vi "Civ idle3_1.vi"() -> ()   [LabVIEW 2013]
uses:
  <vilib>/Analysis/Matrix/Numeric/Conversions/Matrix To Array - RM.vi
  <vilib>/Analysis/Matrix/NI_Matrix.lvlib
panel:
  out "Base dissent":dbl format="%#_4g"
  out "Gold":i64 format="%^#.4g"
  out "Dissent \nmultiplication\nmodifier":dbl
  out "SP income":dbl format="%^#.3g"
  out "EP income":dbl format="%^#.3g"
  out "Land conversion rate":dbl format="%#_4e"
  out "BP income":dbl format="%^#.3g"
  in  "Ticks/s":i32
  out "Gold upkeep":dbl format="%^#_4g"
  out "Gold income/s":dbl format="%^#_4g"
  out "BP upkeep":dbl format="%^#.3g"
  out "Trading level":i32
  out "Build points":dbl format="%^#.3g"
  in  "?":T1(tab)
  out "%Hunters":dbl format="%#_3g"
  in  "%Crafters":dbl
  in  "%Engineers":dbl
  in  "%Scientists":dbl
  in  "%Builders":dbl
  in  "%Warriors":dbl
  in  "Taxes level 0":bool
  in  "Taxes level 1":bool
  in  "Taxes level 2":bool
  in  "Taxes level 3":bool
  out "Taxation\nlevel":dbl format="%#_13g"
  in  "Taxes level 4":bool
  out "Food consumption\nmultiplier":dbl
  out "Food dissent mod":dbl
  in  "Normal food\nconsumption":bool
  in  "Highest food\nconsumption":bool
  in  "Higher food\nconsumption":bool
  in  "Taxes level 5":bool
  in  "Taxes level 6":bool
  out "Military\nScience level":i32
  out "Governance\nlevel":i32
  in  "Military science":bool
  in  "Governance":bool
  in  "Physics":bool
  in  "Construction":bool
  out "Physics level":i32
  out "Construction\nlevel":i32
  out "Economics\nlevel":i32
  in  "Economics":bool
  in  "Biology":bool
  out "Biology\nlevel":i32
  out "# of level 1 sciences":i32
  out "# of level 2 sciences":i32
  out "# of level 3 sciences":i32
  out "# of level 4 sciences":i32
  out "# of level 5 sciences":i32
  out "# of level 6 sciences":i32
  out "# of level 7 sciences":i32
  out "# of level 8 sciences":i32
  out "# of level 9 sciences":i32
  out "# of level 10 sciences":i32
  out "Production\nlevel":i32
  in  "Production":bool
  out "Level 2 science price":i32 format="%^.0g"
  out "Level 1 science price":i32 format="%^.0g"
  out "Level 6 science price":i64 format="%^#.1g"
  out "Level 5 science price":i32 format="%^.0g"
  out "Level 4 science price":i32 format="%^.0g"
  out "Level 7 science price":i64 format="%^.0g"
  out "Level 3 science price":i32 format="%^#.1g"
  out "Level 8 science price":i64 format="%^.0g"
  out "Level 9 science price":i64 format="%^#.1g"
  out "Level 10 science price":i64 format="%.0g"
  out "Spear level":i32
  out "Net level":i32
  in  "Sharpened stick":bool
  in  "Net 1":bool
  in  "Net 2":bool
  in  "Stone\nspear":bool
  in  "Bronze\nSpear":bool
  in  "Iron\nSpear":bool
  out "Construction\ntools level":i32
  in  "Stone tools":bool
  in  "Basic\nmetal\ntools":bool
  in  "Advanced\nmetal\ntools":bool
  in  "Horses":bool
  in  "Selective\nbreeding":bool
  in  "Livestock":bool
  out "Animal\ndomestication\nlevel":i32
  in  "Parchment":bool
  in  "Paper":bool
  in  "Movable typeset":bool
  out "Writing level":i32
  in  "Medicine 3":bool
  in  "Medicine 2":bool
  in  "Medicine 1":bool
  out "Medicine level":i32
  in  "Medicine 4":bool
  in  "Printing\nPress":bool
  in  "Crossbow":bool
  out "Bow level":i32
  in  "Bow 1":bool
  in  "Bow 2":bool
  in  "Longbow":bool
  in  "Farming 1":bool
  out "Farming level":i32
  in  "Farming 2":bool
  out "Sword level":i32
  in  "Steel sword":bool
  in  "Iron sword":bool
  in  "Bronze sword":bool
  out "Tax method\nlevel":i32
  in  "Income tax":bool
  in  "Sales tax":bool
  in  "Tariffs":bool
  out "Siege weapon\nlevel":i32
  in  "Trebuchet":bool
  in  "Catapult":bool
  in  "Ballista":bool
  in  "Cannon":bool
  in  "Howitzer":bool
  in  "Rocket artillery":bool
  in  "Trireme":bool
  in  "Raft":bool
  out "Boat level":i32
  out "Chariot level":i32
  in  "Reinforced\nchariot":bool
  in  "Simple\nchariot":bool
  in  "Caravan":bool
  in  "Caravel":bool
  in  "Steamship":bool
  in  "Mechanical\nTelevision":bool
  out "Optics\nlevel":i32
  in  "Telescope":bool
  in  "Light bulb":bool
  in  "Camera":bool
  in  "LCD monitor":bool
  out "Electronics\nlevel":i32
  in  "Radio":bool
  in  "Computer":bool
  out "Vehicle\nlevel":i32
  in  "Steam Powered Train":bool
  in  "Internal combustion engine (cars)":bool
  in  "Aircraft":bool
  in  "Rocket":bool
  in  "Unlock brick house":bool
  in  "Unlock concrete house":bool
  in  "Unlock paved tar roads":bool
  in  "Unlock multilayer stone roads":bool
  in  "Democracy":bool
  in  "Theocracy":bool
  in  "Warrior\nSociety":bool
  in  "Democracy 2":bool
  in  "Theocracy 2":bool
  in  "Warrior\nSociety 2":bool
  in  "Kingdom":bool
  in  "Republic":bool
  in  "Confederacy":bool
  in  "Senate":bool
  in  "Caste system":bool
  in  "Feudalism":bool
  in  "Empire":bool
  in  "Imperialism":bool
  in  "Free market capitalism":bool
  in  "Harbor level 0":bool
  in  "Harbor level 3":bool
  in  "Harbor level 2":bool
  in  "Harbor level 1":bool
  out "Road level":i32
  out "Hut level":i32
  in  "Hut level 0":bool
  in  "Hut level 1":bool
  in  "Hut level 2":bool
  in  "Hut level 3":bool
  out "Road invested points":dbl
  out "Hut invested points":dbl
  in  "Road level 0":bool
  in  "Road level 3":bool
  in  "Road level 2":bool
  in  "Road level 1":bool
  out "Aqueduct level":i32
  out "Market\ninvested points":dbl
  out "Market level":i32
  out "Aqueduct\ninvested points":dbl
  out "Harbor\ninvested points":dbl
  out "Harbor level":i32
  in  "Aqueduct\nlevel 0":bool
  in  "Aqueduct\nlevel 3":bool
  in  "Aqueduct\nlevel 2":bool
  in  "Aqueduct\nlevel 1":bool
  in  "Switch to brick house":bool
  in  "Switch to hut":bool
  out "Brick house\nunlocked":bool=TRUE
  out "Concrete house\nunlocked":bool=TRUE
  in  "Switch to concrete housing":bool
  out "Paved tar roads\nunlocked":bool=TRUE
  out "Mutilayer\nStone roads\nunlocked":bool=TRUE
  in  "Switch to Paved tar roads":bool
  in  "Switch to Multilayer stone road":bool
  in  "Switch to Stone road":bool
  out "Housing type":string="a"
  out "Road type":string="a"
  in  "Market\nlevel 0":bool
  in  "Market\nlevel 3":bool
  in  "Market\nlevel 2":bool
  in  "Market\nlevel 1":bool
  out "School invested points":dbl
  in  "School\nlevel 1":bool
  in  "School\nlevel 2":bool
  in  "School\nlevel 3":bool
  in  "School\nlevel 0":bool
  out "School level":i32
  in  "Wall level 1":bool
  in  "Wall level 2":bool
  in  "Wall level 3":bool
  in  "Wall level 0":bool
  out "Barracks level":i32
  out "Walls level":i32
  out "Wall invested points":dbl
  out "Barracks\ninvested points":dbl
  in  "Barracks\nlevel 3":bool
  in  "Barracks\nlevel 1":bool
  in  "Barracks\nlevel 0":bool
  in  "Barracks\nlevel 2":bool
  out "University level":i32
  in  "University\nlevel 0":bool
  in  "University\nlevel 3":bool
  in  "University\nlevel 2":bool
  in  "University\nlevel 1":bool
  out "University\ninvested points":dbl
  out "Police force level":i32
  out "Temple level":i32
  out "Police force\ninvested points":dbl
  out "Temple\ninvested points":dbl
  in  "Temple\nlevel 0":bool
  in  "Temple\nlevel 3":bool
  in  "Temple\nlevel 2":bool
  in  "Temple\nlevel 1":bool
  in  "Police force 0":bool
  in  "Police force 3":bool
  in  "Police force 2":bool
  in  "Police force 1":bool
  in  "Make Tier 2\nproducts":bool
  out "Tier 2\nproducts\nupkeep":dbl format="%#_13g"
  out "Tier 3\nproducts\nupkeep":dbl format="%#_13g"
  out "Tier 4\nproducts\nupkeep":dbl format="%#_13g"
  out "Tier 1\nproducts":dbl format="%#_4p"
  out "Tier 2\nproducts":dbl format="%#_13g"
  out "Tier 3\nproducts":dbl format="%#_13g"
  out "Tier 4\nproducts":dbl format="%#_13g"
  out "Tier 1\nproducts\nupkeep":dbl format="%#_13g"
  in  "Make Tier3\nproducts":bool
  in  "Make Tier 4\nproducts":bool
  out "hunting b":dbl
  out "hunting a":dbl
  out "warrior a":dbl
  out "warrior b":dbl
  out "warrior c":dbl
  out "1-Dissent/100":dbl format="%#_13g"
  out "Land conv mult":dbl
  out "Warrior b Gov mult":dbl
  out "Gov Economy\nbuildings mod":dbl
  out "Dissent mult per\nmilitary building":dbl
  out "Gov food mult":dbl
  out "Temp land change/s":dbl
  out "Year":i32
  out "Day":i32
  out "Military Modifier":dbl format="%#_13g"
  out "Taxation\nModifier":dbl format="%#_13g"
  out "Non-land production multiplier":dbl
  out "Hut non-land prod mod":dbl
  out "Hut upkeep":dbl
  out "Hut dissent mod":dbl
  out "Road land prod mod":dbl
  out "Road upkeep":dbl
  out "Road expansion bonus":dbl
  out "Trading level no mod":i32
  out "Taxes dissent mod":dbl
  out "Barracks military bonus":dbl
  out "Barracks upkeep":dbl
  out "Wall upkeep":dbl
  out "Wall dissent mod":dbl
  out "Construction multiplier":dbl
  out "Wall warrior % equivalent":dbl
  out "Gov building\nupkeep mod":dbl
  out "School dissent mod":dbl
  out "School upkeep":dbl
  out "School engineer equivalent":dbl
  out "School SP/EP multiplier":dbl
  out "Medicine dissent mod":dbl
  out "Gov populist\nbuildings mod":dbl
  out "Gov elitist\nbuildings mod":dbl
  out "University SP multiplier":dbl
  out "University dissent mod":dbl
  out "University upkeep":dbl
  out "University scientist equivalent":dbl
  out "Food income":dbl
  out "Gold dbl":dbl format="%#_13g"
  out "Road trade modifier":dbl
  out "Market domestic gold mult":dbl
  out "Aqueduct dissent mod":dbl
  out "Aqueduct upkeep":dbl
  out "Police force dissent mult":dbl
  out "Police force upkeep":dbl
  out "Harbor expansion bonus":dbl
  out "Harbor upkeep":dbl
  out "Market trade gold mult":dbl
  out "Market upkeep":dbl
  out "Temple dissent mod":dbl
  out "Temple upkeep":dbl
  out "Harbor military mod":dbl
  out "SP/EP multiplier":dbl
  out "Temple SP/EP multiplier":dbl
  out "Aqueduct food multiplier":dbl
  out "Police force base dissent mod":dbl
  out "Government":string
  out "Dissent":dbl format="%#_4g"
  out "SP":dbl format="%^#.3g"
  out "EP":dbl format="%^#.3g"
  in  "Percentage or absolute":bool
  out "Engineers":i32 format="%^#.3g"
  out "Crafters":i32 format="%^#.3g"
  out "Scientists":i32 format="%^#.3g"
  in  "#Merchants":dbl
  in  "Assign Merchant":bool
  in  "#Engineers":dbl
  in  "Assign Engineer":bool
  in  "#Scientists":dbl
  in  "Assign Scientist":bool
  out "Warriors":i32 format="%^#.3g"
  in  "Assign Builder":bool
  in  "#Builders":dbl
  out "Builders":i32 format="%^#.3g"
  in  "Assign Warrior":bool
  in  "#Warriors":dbl
  out "Unassigned workers":i32
  in  "Assign Hunters":bool
  in  "#Hunters":dbl
  in  "# people":i32
  in  "Increase\nPopulation":bool
  out "Conquered\nland":dbl format="%^#.3g"
  out "Max hunters":i32 format="%^#.3g"
  out "Hunters":i32 format="%^#.3g"
  out "Food/s":dbl format="%^#_5g"
  out "Permanent\nland":dbl format="%^#.3g"
  out "People":i64 format="%^#.3g"
  in  "Stop Loop":bool
  out "Food":dbl format="%^#_5g"
  # "Produces food, but your permanent land cannot support too many hunters"
  # "Unlock after population hits 25"
  # "Conquers land, starting at 1km^2 per warrior, but has diminishing returns"
  # "Unlock after construction 1"
  # "Produces 1 BP/tick, needed for buildings\nand for building upkeep"
  # "Unlock after population hits 100"
  # "Produces 0.1 SP/tick, used for abstract research which unlock upgrades and provide bonuses"
  # "Unlock after population hits 50"
  # "Produces 0.1 EP/tick, used for designing useful tools and upgrades"
  # "Produces Products, used mostly for late game upgrades.  Production scales with permanent land"
  # "Not yet implemented"
  # "Small income from population, 8% dissent before modifiers"
  # "Medium income from population, 15% dissent before modifiers"
  # "Higher  income from population, 25% dissent before modifiers"
  # "Higher  income from population, 40% dissent before modifiers"
  # "Highest  income from population, 60% dissent before modifiers"
  # "No income from population, no dissent added"
  # "Lowest income from population, 3% dissent before modifiers"
  # "Requires Economics 1"
  # "2 food/s/person,\n-30% dissent"
  # "1 food/s/person, no dissent mod"
  # "1.5 food/s/person,\n-15% dissent"
  # "Requires Governance 2"
  # "Each level costs 1000 *10^current level SP"
  # "Reduces diminishing returns \nfrom military size, unlocks \nnew weapons/tactics"
  # "-5% dissent per level,\nunlocks new governments"
  # "Increases EP and SP generation, \nunlocks various upgrades"
  # "Decreases building upkeep costs,\nunlocks buildings"
  # "Increase gold generation,\nunlocks gold and taxation"
  # "Increase food production,\nunlocks farming and medicine"
  # "Increases production by 20%\nper tier per level"
  # "Costs 2M EP\nRequires military 4,\nWarriors are more effective"
  # "Costs 250EP\nHunters and warriors are more effective"
  # "Costs 3000EP\nRequires military 1,\nHunters and warriors are more effective"
  # "Costs 50k EP\nRequires military 2,\nWarriors are more effective"
  # "Costs 3k EP\nRequires biology 1,\nreduces dissent by 10%"
  # "Costs 30k EP\nRequires biology 2,\nreduces dissent by another 5% (15% total)"
  # "Costs 3M EP\nRequires biology 4,\nreduces dissent by another 5% (20% total)"
  # "Costs 300M EP\nRequires biology 6,\nreduces dissent by another 5% (25% total)"
  # "Costs 10k EP\nHunters can produce more food"
  # "Costs 100k EP\nHunters can produce more food"
  # "Costs 10k EP\nImproves EP and SP production by 10%"
  # "Costs 1M EP\nImproves EP and SP production by 10%"
  # "Costs 100M EP\nImproves EP and SP production by 10%"
  # "Costs 10B EP\nImproves EP and SP production by 10%"
  # "Costs 30k EP\nRequires physics 2, construction 2\nBuilders produce 0.25 more BP/tick"
  # "Costs 500k EP\nRequires physics 3,\nconstruction 3,Builders produce 0.25 more BP/tick"
  # "Costs 200M EP\nRequires physics 5,\nconstruction 5,Builders produce 0.5 more BP/tick"
  # "Costs 30M EP\nRequires Biology 3\nImproves warrior effectiveness,  builder BP/tick by 0.25"
  # "Costs 30k EP\nRequires Biology 1\nImproves hunter food production"
  # "Costs 1M EP\nRequires Biology 2\nImproves warrior effectiveness,  builder BP/tick by 0.25"
  # "Costs 200k EP\nRequires military 2,\nWarriors are much more effective, hunters can produce more food"
  # "Costs 300k EP\nRequires military 3, physics 3\nWarriors and Hunters are more effective"
  # "Costs 30M EP\nRequires military 5, physics 4\nWarriors are more effective"
  # "Costs 1B EP\nRequires military 6, physics 5\nWarriors are more effective"
  # "Costs 300k EP\nRequires physics 3,\nImproves trade and hunting"
  # "Costs 3M EP\nRequires physics 4, military 3\nImproves trade and warriors"
  # "Costs 10B EP\nRequires physics 7\nIncreases trade level by 2 and improves warriors"
  # "Costs 100B EP\nRequires physics 8, military 8\nIncreases trade level by 2 and improves warriors"
  # "Costs 500k EP\nRequires Military 3, Physics 3, Improves warrior effectiveness"
  # "Costs 5M EP\nRequires Military 3, Physics 4, Improves warrior effectiveness"
  # "Costs 10M EP\nRequires Economics 4, Physics 4, Increases trade level"
  # "Costs 1M EP\nRequires Military 3\nImproves warrior effectiveness"
  # "Costs 30M EP\nRequires Military 4\nImproves warrior effectiveness"
  # "Costs 1B EP\nRequires Military 6\nImproves warrior effectiveness"
  # "Costs 1M EP\nRequires Economics 3\nImproves taxation effectiveness by 50%"
  # "Costs 30M EP\nRequires Economics 4\nImproves taxation effectiveness by 50%"
  # "Costs 1B EP\nRequires Economics 6\nImproves taxation effectiveness by 50%"
  # "Costs 10M EP\nRequires Biology 3\nRenames hunters to farmers, massive improvements to food production, increases food from tribute"
  # "Costs 100M EP\nRequires Biology 4\nLarge improvements to food production, increases food from tribute"
  # "Costs 5M EP\nRequires Military 3, Physics 4, Improves\nwarrior effectiveness"
  # "Costs 30M EP\nRequires Military 3, Physics 5, Improves\nwarrior effectiveness"
  # "Costs 300M EP\nRequires Military 4, Physics 6, Improves\nwarrior effectiveness"
  # "Costs 3B EP\nRequires Military 6, Physics 7, Improves\nwarrior effectiveness"
  # "Costs 300B EP\nRequires Military 8, Physics 9, Improves\nwarrior effectiveness"
  # "Costs 3T EP\nRequires Military 9, Physics 9, Improves\nwarrior effectiveness"
  # "Internet, not sure if invention or building"
  # "Unlock sattelite network structure"
  # "Costs 300k, requires construction 3"
  # "Costs 10M, requires construction 5"
  # "Costs 1M, requires construction 3"
  # "Costs 30M, requires construction 5"
  # "Requires Governance 1"
  # "Costs 500M SP\nRequires Governance 6"
  # "Costs 100k SP\nRequires Governance 2"
  # "Costs 5M SP\nRequires Governance 4"
  # "All governments gain base dissent as population increases"
  # "Free market capitalism doubles domestic gold produced by the market"
  # "These 3 have not yet been rebalanced"
  # "Government descriptions"
  # "Government playstyle"
  # "Democracy focuses on permanent land and hunters for its main source of food, and will have to rely on taxes, and eventually markets, for its source of gold income.  Even though the military is weak, it is still necessary to be abel to convert land."
  # "Top row governments belong to the democracy path, and get a large bonus to land conversion, and dissent decreases as permanent land increases.  These governments have a slight reduction to their military effectiveness."
  # "Empire can focus either on benefits from conquered land, benefits from permanent land, or a combination of both.  The production bonuses allow you to maintain more high level buildings."
  # "Middle row governments belong to the empire path, and get bonuses to BP point production and food production.  Later levels get small military bonuses."
  # "Bottom row governments belong to the oligarchy path, and get a massive boost to their military, but have a very small land conversion rate.  Conquering more land reduces dissent for these governments."
  # "Oligarchies focus on their powerful military, and have an economy dependent on tribute and trade from conquered land.  Any sort of military upgrade will provide benefits to all parts of your economy, and the extra conquered land will decrease your dissent"
  # "Reduces dissent by 5,10,15%\nImproves non-land production by 10,20,30%\nRequires Construction 1"
  # "Upkeep:        0                          0.01BP                0.03BP              0.15BP"
  # "Cost:             0                          10k   BP              30k BP             150k BP"
  # "Multiply all hut bonuses by 1.2"
  # "Upkeep:        0                          0.015BP              0.045BP            0.225BP"
  # "Cost:             0                          100k   BP             300k BP           1.5M BP"
  # "Upkeep:        0                           0.01BP                0.03BP              0.15BP"
  # "Multiply all hut bonuses by 1.3"
  # "Cost:             0                          1M   BP               3M BP             15M BP"
  # "Increases trade level by 1,2,3\nImproves land production\n by 10,20,30%\nImproves land conversion\nrate by 20,50,100%\nRequires Construction 1"
  # "Upkeep:        0                          0.02BP                0.06BP              0.2BP"
  # "Cost:             0                          50k BP              150k BP             500k BP"
  # "Increases trade level by 2,4,6"
  # "Upkeep:        0                          0.04BP                0.12BP              0.4BP"
  # "Cost:             0                          500k BP             1.5M BP            5M BP"
  # "Increases trade level by 2,4,6\nImproves land production\nby 15,30,45%\nImproves land conversion by 30,75,150%"
  # "Upkeep:        0                          0.06BP                0.18BP              0.6BP"
  # "Cost:             0                          50M BP             150M BP           500M BP"
  # "Improves food output\n by 10,20,30%\nReduced dissent by 2,4,6%\nRequires Construction 3"
  # "Upkeep:              0                     0.01BP             0.03BP                0.15BP"
  # "Cost:                   0                     500k BP           1.5M BP             5M BP"
  # "Improves gold from trade by 15,30,45%\nGives a gold income from permanent land equal to 1,2,3 times the trade income from conquered land\nRequires construction 2, economics 3"
  # "Upkeep:              0                     0.04BP             0.12BP                0.4BP"
  # "Cost:                   0                     5M BP             15M BP              50M BP"
  # "Increases trade level by 1,2,3\nIncreases military effectiveness (b) by 10,20,30%\nImproves land conversion\nrate by 10,25,50%\nRequires Boat level 1"
  # "Upkeep:             0                     0.04BP                0.12BP              0.4BP"
  # "Cost:                  0                     500k BP              1.5M BP           5M BP"
  # "Increases military effectiveness (b) by 10,20,30%\nRequires Construction 2, Military 2"
  # "Upkeep:        0                          0.001GP             0.003GP           0.01GP"
  # "Cost:             0                          100k BP             300k BP            1M BP"
  # "Adds to the base strength of your military, giving the equivalent of 2,4,6% of your population as warriors\nReduces dissent by 5,10,15%\nRequires Construction 3, Military 2"
  # "Upkeep:        0                          0.002GP            0.006GP           0.02GP"
  # "Cost:             0                          1M BP              3M BP              10M BP"
  # "Provides a 5,10,15% bonus to SP/EP production, reduces dissent by 2,4,6%, adds 1,2,3% of population to base  engineers\nRequires Construction 2, Governance 2"
  # "Upkeep:        0                          0.001GP             0.003GP           0.01GP"
  # "Cost:             0                          200k BP             600k BP            2M BP"
  # "Provides a 15,30,45% bonus to SP production, reduces dissent by 2,4,6%, adds 2,4,6% of population to base  scientists\nRequires Construction 2, Governance 2"
  # "Upkeep:        0                          0.005GP             0.015GP          0.05GP"
  # "Cost:             0                          600k BP             2M BP             5M BP"
  # "Use only when base dissent is high"
  # "Increases base dissent by 5, 20, 50%\nDecreases dissent multiplier by 13, 26, 40%\nRequires Governance 3"
  # "Upkeep:        0                          0.002GP             0.006GP          0.02 GP"
  # "Cost:             0                          100k GP             1M GP             10M GP"
  # "Reduces dissent by 3,6,9%,\nRequires Construction 1\n3 times as effective if you\nare a theocracy"
  # "Upkeep:        0                          0.001GP             0.003GP           0.01GP"
  # "Cost:             0                          500 GP               10k GP             500k GP"
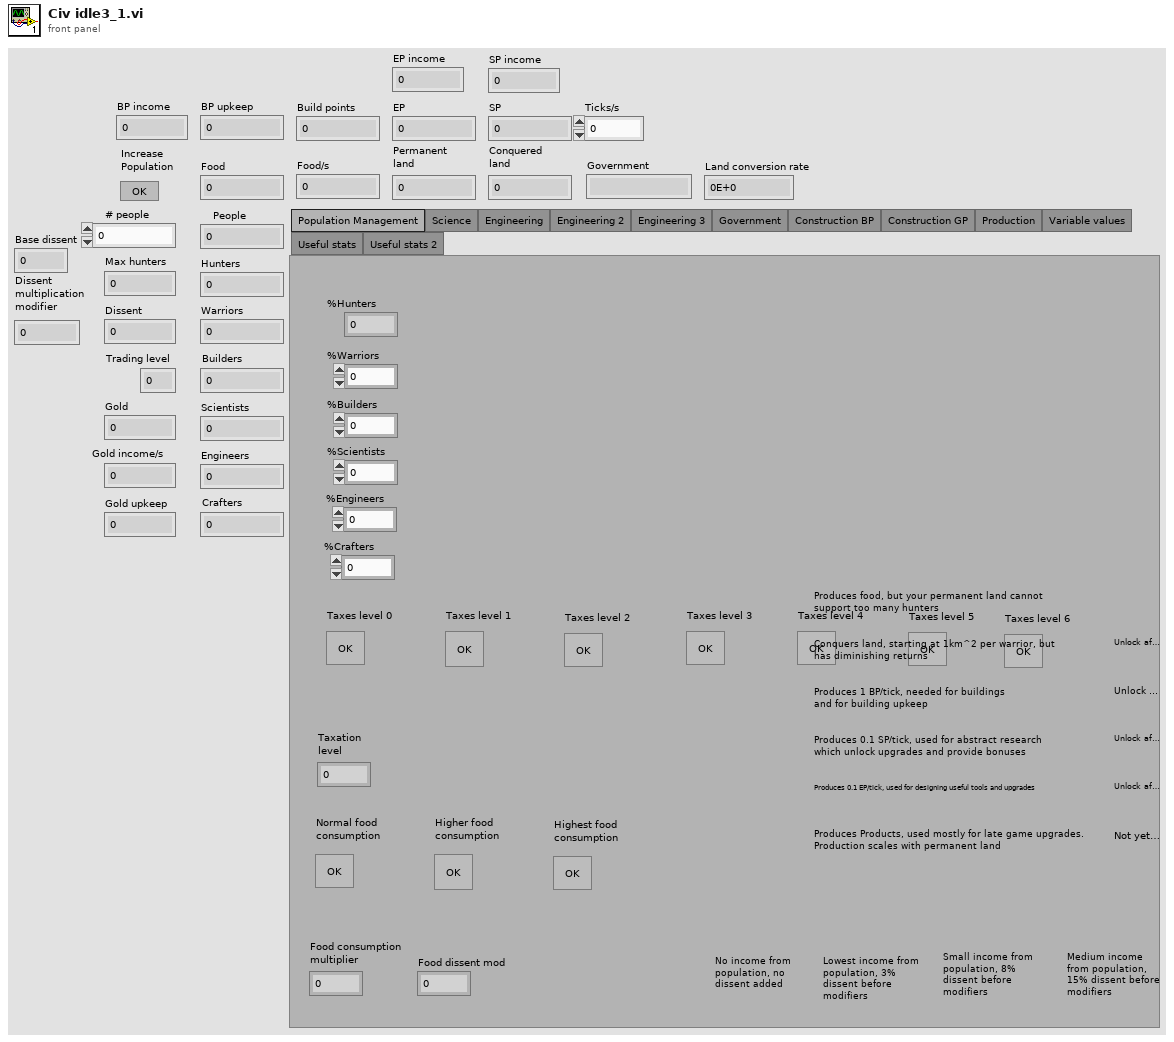
[diagram p1: front panel]
types:
  T1 = enum32{"Population Management", "Science", "Engineering", "Engineering 2", "Engineering 3", "Government", "Construction BP", "Construction GP", "Production", "Variable values", "Useful stats", "Useful stats 2"}
  T2 = typedef "NI_Matrix.lvlib/RealMatrix.ctl" = dbl[][]
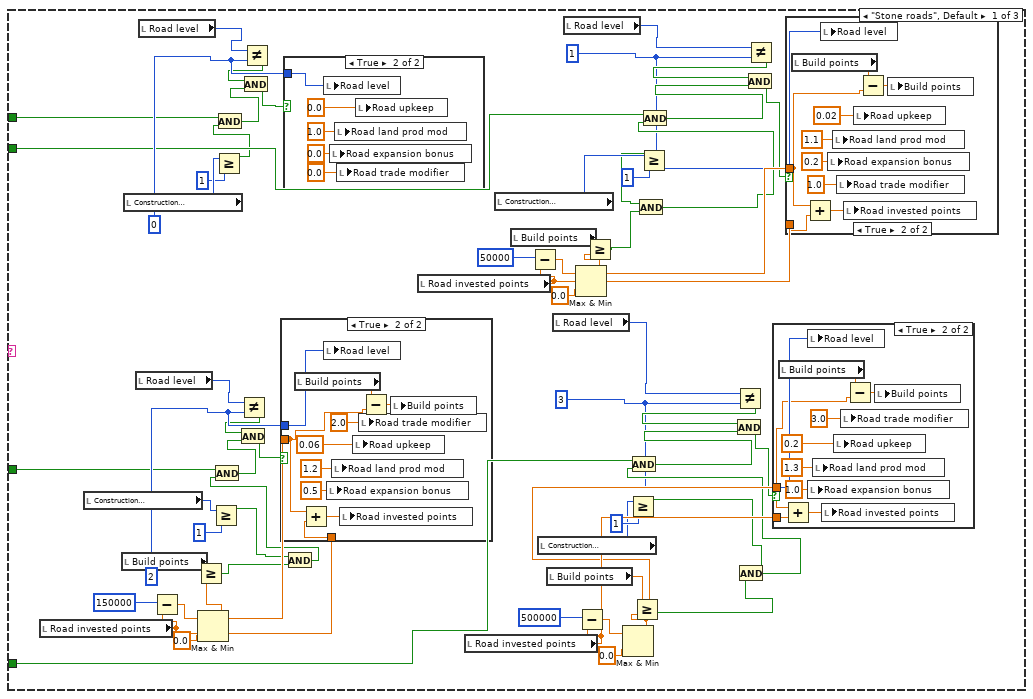
[diagram p18: hidden frame]
diagram:
  n1 = while {
    i -> [w2088]
    stop <- "Stop Loop" stop-if-true
    w220 = 0 ("y")
    w219 = 3 ("y")
    w202 = 2 ("y")
    w201 = 1 ("y")
    w234 = 0 ("y")
    w235 = 3 ("y")
    w252 = 2 ("y")
    w253 = 1 ("y")
    w296 = 500000000 ("y")
    w331 = "Empire" ("y")
    w295 = 500000000 ("y")
    w309 = "Imperialism" ("y")
    w294 = 500000000 ("y")
    w297 = "Free market capitalism" ("y")
    w355 = 30000000 ("y")
    w334 = 1000000 ("y")
    w373 = 10000000 ("y")
    w396 = 300000 ("y")
    w413 = 30000000 ("y")
    w422 = 30000000 ("y")
    w439 = 30000000 ("y")
    w448 = 30000000 ("y")
    w465 = 30000000 ("y")
    w480 = 30000000 ("y")
    w499 = 300000000 ("y")
    w510 = 300000000 ("y")
    w537 = 300000000 ("y")
    w548 = 30000000 ("y")
    w557 = 5000000 ("y")
    w588 = 3000000 ("y")
    w577 = 300000 ("y")
    w603 = 100000000 ("y")
    w614 = 300000000 ("y")
    w569 = 1000000000 ("y")
    w652 = 6 ("y")
    w655 = 5 ("y")
    w715 = 0 ("y")
    w714 = 3 ("y")
    w697 = 2 ("y")
    w696 = 1 ("y")
    w731 = 0 ("y")
    w732 = 3 ("y")
    w749 = 2 ("y")
    w750 = 1 ("y")
    w839 = 0 ("y")
    w838 = 3 ("y")
    w821 = 2 ("y")
    w820 = 1 ("y")
    w873 = i64 3000000000000 ("y")
    w884 = i64 300000000000 ("y")
    w905 = i64 3000000000 ("y")
    w942 = 300000000 ("y")
    w931 = 30000000 ("y")
    w922 = 5000000 ("y")
    w975 = 10000000 ("y")
    w986 = 5000000 ("y")
    w995 = 500000 ("y")
    w1011 = 1000000000 ("y")
    w1022 = 30000000 ("y")
    w1031 = 1000000 ("y")
    w1089 = 1000000000 ("y")
    w1078 = 30000000 ("y")
    w1069 = 1000000 ("y")
    w1098 = 30000000 ("y")
    w1109 = 1000000 ("y")
    w1118 = 30000 ("y")
    w1149 = 100000000 ("y")
    w1138 = 1000000 ("y")
    w1129 = 10000 ("y")
    w1177 = 1 ("y")
    w1169 = 2 ("y")
    w1168 = 1.5 ("y")
    w1209 = 0 ("y")
    w1210 = 3 ("y")
    w1229 = 2 ("y")
    w1230 = 1 ("y")
    w1268 = 30000000 ("y")
    w1284 = 500000 ("y")
    w1302 = 3000000 ("y")
    w1313 = 30000 ("y")
    w1328 = 3000 ("y")
    w1385 = 0 ("y")
    w1384 = 3 ("y")
    w1365 = 2 ("y")
    w1364 = 1 ("y")
    w1408 = "Senate" ("y")
    w1432 = "Caste system" ("y")
    w1445 = "Feudalism" ("y")
    w1483 = "Kingdom" ("y")
    w1459 = "Republic" ("y")
    w1446 = "Confederacy" ("y")
    w1498 = 4 ("y")
    w1515 = 500000 ("y")
    w1526 = 30000 ("y")
    w1571 = 0 ("y")
    w1572 = 3 ("y")
    w1591 = 2 ("y")
    w1592 = 1 ("y")
    w1634 = 0 ("y")
    w1635 = 3 ("y")
    w1650 = 2 ("y")
    w1651 = 1 ("y")
    w1766 = 0 ("y")
    w1765 = 3 ("y")
    w1746 = 2 ("y")
    w1745 = 1 ("y")
    w1781 = 100000000 ("y")
    w1807 = 10000000 ("y")
    w1830 = 3000000 ("y")
    w1841 = 300000 ("y")
    w1873 = 300000 ("y")
    w1899 = 200000 ("y")
    w1902 = 2000000 ("y")
    w1901 = 50000 ("y")
    w1965 = "Warrior Society 2" ("y")
    w1989 = "Theocracy 2" ("y")
    w2002 = "Democracy 2" ("y")
    w2008 = "Warrior Society" ("y")
    w2021 = "Theocracy" ("y")
    w2035 = "Democracy" ("y")
    w2058 = 250 ("y")
    # "SCIENCES"
    # "GOVERNMENTS"
    # "ENGINEERING"
    n2 = local read "Police force\ninvested points"() -> (w274:dbl)
    n3 = local read "Barracks\ninvested points"() -> (w1666:dbl)
    n4 = local read "Food consumption\nmultiplier"() -> (w1178:dbl)
    n5 = local read "Wall invested points"() -> (w1615:dbl)
    n6 = local read "Aqueduct\ninvested points"() -> (w674:dbl)
    n7 = local read "Food consumption\nmultiplier"() -> (w1170:dbl)
    n8 = local read "Governance\nlevel"() -> (w1175:i32)
    n9 = local read "Governance\nlevel"() -> (w1183:i32)
    n10 = local read "Governance\nlevel"() -> (w245:i32)
    n11 = local read "Construction\nlevel"() -> (w1754:i32)
    n12 = local read "Construction\nlevel"() -> (w1774:i32)
    n13 = local read "Construction\nlevel"() -> (w1583:i32)
    n14 = local read "Military\nScience level"() -> (w1560:i32)
    n15 = local read "Construction\nlevel"() -> (w704:i32)
    n16 = local read "Police force level"() -> (w249:i32)
    n17 = local read "Gold dbl"() -> (w641:dbl)
    n18 = local read "Police force level"() -> (w233:i32)
    n19 = local read "Governance\nlevel"() -> (w229:i32)
    n20 = local read "Build points"() -> (w1670:dbl)
    n21 = local read "Military\nScience level"() -> (w1547:i32)
    n22 = local read "Gold dbl"() -> (w270:dbl)
    n23 = local read "Construction\nlevel"() -> (w1563:i32)
    n24 = local read "Barracks level"() -> (w1749:i32)
    n25 = local read "Build points"() -> (w1611:dbl)
    n26 = local read "Barracks level"() -> (w1769:i32)
    n27 = Subtract(x=1000000 ("y"), y=w274) -> (x-y=w267:dbl)
    n28 = local read "Military\nScience level"() -> (w1541:i32)
    n29 = local read "Walls level"() -> (w1568:i32)
    n30 = Subtract(x=300000 ("y"), y=w1666) -> (x-y=w1673:dbl)
    n31 = local read "Walls level"() -> (w1588:i32)
    n32 = local read "Build points"() -> (w678:dbl)
    n33 = Subtract(x=3000000 ("y"), y=w1615) -> (x-y=w1608:dbl)
    n34 = local read "Construction\nlevel"() -> (w720:i32)
    n35 = local read "Aqueduct level"() -> (w700:i32)
    n36 = local read "Aqueduct level"() -> (w716:i32)
    n37 = Greater Or Equal?(x=w1183, y=2) -> (x >= y?=w1185:bool)
    n38 = And(x="Normal food\nconsumption", y=w1185) -> (x .and. y?=w1181:bool)
    n39 = Subtract(x=1500000 ("y"), y=w674) -> (x-y=w681:dbl)
    n40 = Greater Or Equal?(x=w1175, y=2) -> (x >= y?=w1187:bool)
    n41 = And(x="Highest food\nconsumption", y=w1187) -> (x .and. y?=w1173:bool)
    n42 = local read "Ticks/s"() -> (w1489:i32)
    n43 = Not Equal?(x=w1178, y=w1177) -> (x != y?=w1180:bool)
    n44 = And(x=w1180, y=w1181) -> (x .and. y?=w1179:bool)
    n45 = Max & Min(x=w1673, y=0.0) -> (max(x,y)=w1668:dbl)  [unwired: 1 out]
    n46 = Max & Min(x=w1608, y=0.0) -> (max(x,y)=w1613:dbl)  [unwired: 1 out]
    n47 = Not Equal?(x=w1170, y=w1169) -> (x != y?=w1172:bool)
    n48 = And(x=w1172, y=w1173) -> (x .and. y?=w1171:bool)
    n49 = Max & Min(x=w267, y=0.0) -> (max(x,y)=w272:dbl)  [unwired: 1 out]
    n50 = Greater Or Equal?(x=w1611, y=w1613) -> (x >= y?=w1612:bool)
    n51 = for {
      N: 1 -> [_]
      tunnel: [w3602] -> w1735 mode=indexing
      n52 = local read "Market domestic gold mult"() -> (w3547:dbl)
      n53 = local read "Permanent\nland"() -> (w3541:dbl)
      n54 = local read "Gov building\nupkeep mod"() -> (w3537:dbl)
      n55 = local read "Market trade gold mult"() -> (w3543:dbl)
      n56 = local read "Conquered\nland"() -> (w3546:dbl)
      n57 = local read "Construction multiplier"() -> (w3624:dbl)
      n58 = local read "Production\nlevel"() -> (w3598:i32)
      n59 = local read "Permanent\nland"() -> (w3599:dbl)
      n60 = local read "University scientist equivalent"() -> (w3615:dbl)
      n61 = local read "Taxation\nlevel"() -> (w3659:dbl)
      n62 = local read "1-Dissent/100"() -> (w3597:dbl)
      n63 = local read "Conquered\nland"() -> (w3673:dbl)
      n64 = local read "Government"() -> (w3539:string)
      n65 = case shown="\"Free market capitalism\"" w3539 {
        tunnel: [1.0 2.0] -> w3538
        frame "False", Default {
        }
        frame "Free market capitalism" {
        }
      }
      n66 = Multiply(x=w3538, y=w3541) -> (x*y=w3540:dbl)
      n67 = Multiply(x=w3547, y=w3540) -> (x*y=w3545:dbl)
      n68 = local read "Non-land production multiplier"() -> (w3573:dbl)
      n69 = local read "Tier 2\nproducts"() -> (w3588:dbl)
      n70 = local read "SP/EP multiplier"() -> (w3618:dbl)
      n71 = local read "University SP multiplier"() -> (w3612:dbl)
      n72 = local read "Economics\nlevel"() -> (w3660:i32)
      n73 = local read "People"() -> (w3602:i64)
      n74 = local read "Crafters"() -> (w3603:i32)
      n75 = Add(x=w3546, y=w3545) -> (x+y=w3544:dbl)
      n76 = local read "Economics\nlevel"() -> (w3664:i32)
      n77 = local read "Trading level"() -> (w3663:i32)
      n78 = Divide(x=1.0, y=w3537) -> (x/y=w3535:dbl)
      n79 = local read "Taxation\nModifier"() -> (w3657:dbl)
      n80 = local read "Tax method\nlevel"() -> (w3606:i32)
      n81 = local read "Non-land production multiplier"() -> (w3648:dbl)
      n82 = local read "School engineer equivalent"() -> (w3621:dbl)
      n83 = Multiply(x=w3543, y=w3544) -> (x*y=w3542:dbl)
      n84 = local read "1-Dissent/100"() -> (w3650:dbl)
      n85 = local read "Physics level"() -> (w3651:i32)
      n86 = local read "Tier 2\nproducts\nupkeep"() -> (w3579:dbl)
      n87 = case shown="\"Confederacy\"" w3539 {
        tunnel: w3602 -> [w3726 w3737 w3759 w3778 w3787 w3807 w3819 w3842 w3858 w3881 w3895 w3916 w3932 w3962 w3975 w3991 _ _ _ _ _ _ _ _ _ _ _ _]
        tunnel: w3599 -> [_ w3746 w3760 _ _ _ _ w3847 w3857 _ w3900 _ w3934 _ _ w3993 _ _ _ _ _ _ _ _ _ _ _ _]
        tunnel: [w3729 w3731 w3750 w3775 w3790 w3800 w3821 w3839 w3856 w3870 w3888 w3910 w3925 w3950 w3971 w3976 _ _ _ _ _ _ _ _ _ _ _ _] -> w3674
        tunnel: w3673 -> [_ _ _ _ _ w3811 w3820 w3846 _ _ w3899 w3919 _ w3958 _ _ _ _ _ _ _ _ _ _ _ _ _ _]
        tunnel: [1.0 0.85 0.7 1 1 2 3 1.5 ("y") 1.0 ("y") 1.5 ("y") 3.0 ("y") 4.0 ("y") 0.7 ("y") 5.0 ("y") 2.0 ("y") 0.8 ("y") _ _ _ _ _ _ _ _ _ _ _ _] -> w3672
        tunnel: [1.0 2.0 4.0 1.0 1.0 0.1 0.025 1.5 ("y") 3.0 ("y") 1.0 ("y") 0.1 ("y") 0.025 ("y") 8.0 ("y") 0.015 ("y") 1.0 ("y") 8.0 ("y") _ _ _ _ _ _ _ _ _ _ _ _] -> w3671
        tunnel: [1 1 1 0.666 0.5 1 1 1.0 ("y") 0.5 ("y") 0.5 ("y") 1.0 ("y") 1.0 ("y") 1.0 ("y") 1.0 ("y") 0.5 ("y") 1.0 ("y") _ _ _ _ _ _ _ _ _ _ _ _] -> w3550
        tunnel: [1.0 ("y") 1.25 ("y") 1.5 ("y") 0.75 ("y") 0.5 ("y") 0.8 ("y") 0.7 ("y") 1.25 ("y") 2.0 ("y") 1.0 ("y") 0.5 ("y") 0.5 ("y") 2.5 ("y") 0.5 ("y") 1.0 ("y") 2.5 ("y") _ _ _ _ _ _ _ _ _ _ _ _] -> _
        tunnel: [1.0 ("y") 0.75 ("y") 0.5 ("y") 1.5 ("y") 2.0 ("y") 1.5 ("y") 1.5 ("y") 1.25 ("y") 0.5 ("y") 1.0 ("y") 1.5 ("y") 2.0 ("y") 0.5 ("y") 2.0 ("y") 1.0 ("y") 0.5 ("y") _ _ _ _ _ _ _ _ _ _ _ _] -> _
        tunnel: [1.0 ("y") 1.0 ("y") 1.0 ("y") 0.98 ("y") 0.98 ("y") 0.96 ("y") 0.96 ("y") 0.96 ("y") 1.0 ("y") 0.98 ("y") 0.96 ("y") 1.0 ("y") 1.0 ("y") 1.0 ("y") 0.98 ("y") 1.0 ("y") _ _ _ _ _ _ _ _ _ _ _ _] -> _
        tunnel: [1.0 ("y") _ _ _ _ _ _ 1.25 ("y") 1.5 ("y") 0.7 ("y") 0.5 ("y") 0.5 ("y") 1.0 ("y") 0.5 ("y") 0.7 ("y") 2.0 ("y") _ _ _ _ _ _ _ _ _ _ _ _] -> _
        tunnel: [1.0 ("y") 1.0 ("y") 1.0 ("y") 1.1 ("y") 1.15 ("y") 1.0 ("y") 1.0 ("y") 1.0 ("y") 1.0 ("y") 1.15 ("y") 1.0 ("y") 1.0 ("y") 1.0 ("y") 1.0 ("y") 1.2 ("y") 1.0 ("y") _ _ _ _ _ _ _ _ _ _ _ _] -> w3549
        frame "Tribe", Default {
          n88 = Divide(x=w3726, y=i64 4) -> (x/y=w3724:dbl)
          n89 = Subtract(x=w3724, y=i64 25) -> (x-y=w3729:dbl)
        }
        frame "Democracy" {
          n90 = Power Of X(1:w3737, 2:1.1 ("y")) -> (0:w3735:dbl)
          n91 = Square Root(x=w3746) -> (sqrt(x)=w3745:dbl)
          n92 = Divide(x=w3735, y=w3745) -> (x/y=w3744:dbl)
          n93 = Square Root(x=w3744) -> (sqrt(x)=w3748:dbl)
          n94 = Multiply(x=2, y=w3748) -> (x*y=w3733:dbl)
          n95 = Subtract(x=w3733, y=10.0) -> (x-y=w3731:dbl)
        }
        frame "Democracy 2" {
          n96 = Square Root(x=w3760) -> (sqrt(x)=w3764:dbl)
          n97 = Divide(x=w3759, y=w3764) -> (x/y=w3763:dbl)
          n98 = Square Root(x=w3763) -> (sqrt(x)=w3754:dbl)
          n99 = Multiply(x=w3754, y=1.9) -> (x*y=w3751:dbl)
          n100 = Subtract(x=w3751, y=10.0) -> (x-y=w3750:dbl)
        }
        frame "Theocracy" {
          n101 = Y-th Root of X(1:w3778, 2:2.8 ("y")) -> (0:w3768:dbl)
          n102 = Multiply(x=w3768, y=2.0) -> (x*y=w3766:dbl)
          n103 = Add(x=w3766, y=10.0) -> (x+y=w3775:dbl)
        }
        frame "Theocracy 2" {
          n104 = Y-th Root of X(1:w3787, 2:3.3 ("y")) -> (0:w3781:dbl)
          n105 = Multiply(x=w3781, y=1.5) -> (x*y=w3782:dbl)
          n106 = Add(x=w3782, y=15.0) -> (x+y=w3790:dbl)
        }
        frame "Warrior Society" {
          n107 = Y-th Root of X(1:w3807, 2:i64 3 ("y")) -> (0:w3804:dbl)
          n108 = Y-th Root of X(1:w3811, 2:3.0 ("y")) -> (0:w3810:dbl)
          n109 = Multiply(x=3.5, y=w3804) -> (x*y=w3803:dbl)
          n110 = Add(x=w3803, y=5.0) -> (x+y=w3802:dbl)
          n111 = Multiply(x=w3810, y=2.0) -> (x*y=w3801:dbl)
          n112 = Subtract(x=w3802, y=w3801) -> (x-y=w3800:dbl)
        }
        frame "Warrior Society 2" {
          n113 = Y-th Root of X(1:w3819, 2:i64 3 ("y")) -> (0:w3829:dbl)
          n114 = Y-th Root of X(1:w3820, 2:3.0 ("y")) -> (0:w3825:dbl)
          n115 = Multiply(x=2.2, y=w3829) -> (x*y=w3830:dbl)
          n116 = Add(x=w3830, y=5.0) -> (x+y=w3831:dbl)
          n117 = Multiply(x=w3825, y=2.0) -> (x*y=w3832:dbl)
          n118 = Subtract(x=w3831, y=w3832) -> (x-y=w3821:dbl)
        }
        frame "Senate" {
          n119 = Multiply(x=w3847, y=w3846) -> (x*y=w3845:dbl)
          n120 = Power Of X(1:w3845, 2:0.3 ("y")) -> (0:w3843:dbl)
          n121 = Divide(x=w3842, y=w3843) -> (x/y=w3841:dbl)
          n122 = Y-th Root of X(1:w3841, 2:2.0 ("y")) -> (0:w3837:dbl)
          n123 = Multiply(x=1.5, y=w3837) -> (x*y=w3839:dbl)
        }
        frame "Republic" {
          n124 = Power Of X(1:w3857, 2:0.6 ("y")) -> (0:w3863:dbl)
          n125 = Divide(x=w3858, y=w3863) -> (x/y=w3862:dbl)
          n126 = Y-th Root of X(1:w3862, 2:2.0 ("y")) -> (0:w3859:dbl)
          n127 = Multiply(x=1.5, y=w3859) -> (x*y=w3856:dbl)
        }
        frame "Kingdom" {
          n128 = Y-th Root of X(1:w3881, 2:3.8 ("y")) -> (0:w3872:dbl)
          n129 = Multiply(x=2.0, y=w3872) -> (x*y=w3870:dbl)
        }
        frame "Feudalism" {
          n130 = Multiply(x=w3900, y=w3899) -> (x*y=w3898:dbl)
          n131 = Y-th Root of X(1:w3895, 2:3.0 ("y")) -> (0:w3894:dbl)
          n132 = Y-th Root of X(1:w3898, 2:7.0 ("y")) -> (0:w3889:dbl)
          n133 = Divide(x=w3894, y=2.0) -> (x/y=w3892:dbl)
          n134 = Add(x=w3892, y=5.0) -> (x+y=w3890:dbl)
          n135 = Subtract(x=w3890, y=w3889) -> (x-y=w3888:dbl)
        }
        frame "Caste system" {
          n136 = Y-th Root of X(1:w3919, 2:3.5 ("y")) -> (0:w3906:dbl)
          n137 = Y-th Root of X(1:w3916, 2:3.5 ("y")) -> (0:w3915:dbl)
          n138 = Multiply(x=w3915, y=2.5) -> (x*y=w3913:dbl)
          n139 = Multiply(x=w3906, y=2.0) -> (x*y=w3905:dbl)
          n140 = Add(x=w3913, y=5.0) -> (x+y=w3911:dbl)
          n141 = Subtract(x=w3911, y=w3905) -> (x-y=w3910:dbl)
        }
        frame "Confederacy" {
          n142 = Power Of X(1:w3934, 2:0.58 ("y")) -> (0:w3931:dbl)
          n143 = Divide(x=w3932, y=w3931) -> (x/y=w3930:dbl)
          n144 = Square Root(x=w3930) -> (sqrt(x)=w3929:dbl)
          n145 = Multiply(x=1.7, y=w3929) -> (x*y=w3926:dbl)
          n146 = Subtract(x=w3926, y=10.0) -> (x-y=w3925:dbl)
        }
        frame "Imperialism" {
          n147 = Y-th Root of X(1:w3962, 2:3.75 ("y")) -> (0:w3960:dbl)
          n148 = Y-th Root of X(1:w3958, 2:3.75 ("y")) -> (0:w3956:dbl)
          n149 = Multiply(x=w3960, y=2.5) -> (x*y=w3954:dbl)
          n150 = Multiply(x=w3956, y=2.2) -> (x*y=w3953:dbl)
          n151 = Subtract(x=w3954, y=w3953) -> (x-y=w3952:dbl)
          n152 = Add(x=w3952, y=5.0) -> (x+y=w3950:dbl)
        }
        frame "Empire" {
          n153 = Y-th Root of X(1:w3975, 2:4.0 ("y")) -> (0:w3973:dbl)
          n154 = Multiply(x=w3973, y=1.5) -> (x*y=w3971:dbl)
        }
        frame "Free market capitalism" {
          n155 = Power Of X(1:w3993, 2:0.6 ("y")) -> (0:w3990:dbl)
          n156 = Divide(x=w3991, y=w3990) -> (x/y=w3989:dbl)
          n157 = Square Root(x=w3989) -> (sqrt(x)=w3988:dbl)
          n158 = Multiply(x=1.3, y=w3988) -> (x*y=w3978:dbl)
          n159 = Subtract(x=w3978, y=10.0) -> (x-y=w3976:dbl)
        }
        frame "Corporatism" {
        }
        frame "Fascism" {
        }
        frame "Communist dictatorship" {
        }
        frame "Socialism" {
        }
        frame "Advanced democracy?" {
        }
        frame "Advanced imperialism?" {
        }
        frame "Meritocracy" {
        }
        frame "Genetically optimized workforce" {
        }
        frame "Future democracy?" {
        }
        frame "Hivemind" {
        }
        frame "AI overlord" {
        }
        frame "Robots do all work" {
        }
      }
      n160 = local read "Builders"() -> (w3634:i32)
      n161 = Power Of X(1:w3602, 2:-0.5 ("y")) -> (0:w3600:dbl)
      n162 = Power Of X(1:1.2 ("x"), 2:w3598) -> (0:w3587:dbl)
      n163 = local read "Build points"() -> (w3626:dbl)
      n164 = local read "Build points"() -> (w3632:dbl)
      n165 = Compound Arithmetic op=MULTIPLY(w3603, w3573, w3600, w3599, w3587, w3597, 0.001 ("x")) -> (w3595:dbl)
      n166 = local read "Tier 3\nproducts"() -> (w3585:dbl)
      n167 = local read "Tier 1\nproducts"() -> (w3594:dbl)
      n168 = Add(x=w3595, y=w3594) -> (x+y=w3592:dbl)
      n169 = local read "Tier 1\nproducts\nupkeep"() -> (w3591:dbl)
      n170 = local read "Dissent"() -> (w3668:dbl)
      n171 = local read "Tier 3\nproducts\nupkeep"() -> (w3577:dbl)
      n172 = Power Of X(1:1.5 ("x"), 2:w3606) -> (0:w3604:dbl)
      n173 = local read "Tier 4\nproducts\nupkeep"() -> (w3576:dbl)
      n174 = Compound Arithmetic op=MULTIPLY(w3664, w3663, w3542, 0.001 ("value")) -> (w3631:dbl)
      n175 = local write "Dissent mult per\nmilitary building"(1.0 ("y")) -> ()
      n176 = local read "Gold dbl"() -> (w3661:dbl)
      n177 = Compound Arithmetic op=MULTIPLY(w3602, w3660, w3659, w3657, 0.0005 ("value"), w3604) -> (w3630:dbl)
      n178 = local write "Gov populist\nbuildings mod"(1.0 ("y")) -> ()
      n179 = local write "Gov elitist\nbuildings mod"(1.0 ("y")) -> ()
      n180 = Power Of X(1:1.1 ("x"), 2:w3651) -> (0:w3636:dbl)
      n181 = Subtract(x=w3592, y=w3591) -> (x-y=w3572:dbl)
      n182 = Divide(x=w3626, y=10.0) -> (x/y=w3625:dbl)
      n183 = Compound Arithmetic op=ADD(w3661, w3631, w3630) -> (w3652:dbl)
      n184 = Divide(x=w3668, y=100.0) -> (x/y=w3670:dbl)
      n185 = local write "Gov food mult"(w3549) -> ()
      n186 = local read "Dissent \nmultiplication\nmodifier"() -> (w3645:dbl)
      n187 = Compound Arithmetic op=MULTIPLY(w3636, w3650, 0.1, w3648, w3618) -> (w3637:dbl)
      n188 = Divide(x=w3637, y=w3636) -> (x/y=w3635:dbl)
      n189 = Compound Arithmetic op=MULTIPLY(w3635, 10.0 ("value"), w3634, w3624, w3535) -> (w3623:dbl)
      n190 = Add(x=w3623, y=w3632) -> (x+y=w3633:dbl)
      n191 = Less?(x=w3652, y=-50.0) -> (x < y?=w3655:bool)
      n192 = local read "Tier 4\nproducts"() -> (w3582:dbl)
      n193 = Greater?(x=w3572, y=0.0) -> (0:w3570:bool)
      n194 = Subtract(x=1.0, y=w3670) -> (x-y=w3666:dbl)
      n195 = Add(x=w3631, y=w3630) -> (x+y=w3629:dbl)
      n196 = local read "Engineers"() -> (w3620:i32)
      n197 = And(x="Make Tier 2\nproducts", y=w3570) -> (x .and. y?=w3568:bool)
      n198 = local write "Build points"(w3633) -> ()
      n199 = local write "Gold dbl"(w3652) -> ()
      n200 = local write "Gold income/s"(w3629) -> ()
      n201 = case shown="True" w3655 {
        tunnel: w3652 -> [_ w3713]
        tunnel: w3602 -> [_ w3717]
        tunnel: [0 w3714] -> w3642
        frame False {
        }
        frame True {
          n202 = Negate(x=w3713) -> (-x=w3712:dbl)
          n203 = Divide(x=w3712, y=w3717) -> (x/y=w3716:dbl)
          n204 = Max & Min(x=w3716, y=20.0) -> (min(x,y)=w3714:dbl)  [unwired: 1 out]
        }
      }
      n205 = local read "Scientists"() -> (w3616:i32)
      n206 = local read "Police force base dissent mod"() -> (w3548:dbl)
      n207 = Less?(x=w3625, y=-50.0) -> (x < y?=w3644:bool)
      n208 = local write "1-Dissent/100"(w3666) -> ()
      n209 = local read "Taxes dissent mod"() -> (w3675:dbl)
      n210 = local write "Warrior b Gov mult"(w3672) -> ()
      n211 = case shown="True" w3568 {
        tunnel: w3572 -> [w3697 w3703]
        tunnel: w3587 -> [_ w3700]
        tunnel: [w3697 w3699] -> w3593
        tunnel: [0.0 w3698] -> w3589
        frame False {
        }
        frame True {
          n212 = Divide(x=100.0 ("y"), y=w3700) -> (x/y=w3702:dbl)
          n213 = Quotient & Remainder(x=w3703, y=w3702) -> (x-y*floor(x/y)=w3699:dbl, floor(x/y)=w3698:dbl)
        }
      }
      n214 = Add(x=w3589, y=w3588) -> (x+y=w3580:dbl)
      n215 = Subtract(x=w3580, y=w3579) -> (x-y=w3566:dbl)
      n216 = Greater?(x=w3566, y=0.0) -> (0:w3565:bool)
      n217 = And(x="Make Tier3\nproducts", y=w3565) -> (x .and. y?=w3563:bool)
      n218 = case shown="True" w3563 {
        tunnel: w3566 -> [w3689 w3695]
        tunnel: w3587 -> [_ w3692]
        tunnel: [w3689 w3691] -> w3586
        tunnel: [0.0 w3690] -> w3584
        frame False {
        }
        frame True {
          n219 = Divide(x=100.0 ("y"), y=w3692) -> (x/y=w3694:dbl)
          n220 = Quotient & Remainder(x=w3695, y=w3694) -> (x-y*floor(x/y)=w3691:dbl, floor(x/y)=w3690:dbl)
        }
      }
      n221 = local write "Tier 2\nproducts"(w3586) -> ()
      n222 = Add(x=w3584, y=w3585) -> (x+y=w3578:dbl)
      n223 = Subtract(x=w3578, y=w3577) -> (x-y=w3558:dbl)
      n224 = Greater?(x=w3558, y=0.0) -> (0:w3562:bool)
      n225 = And(x="Make Tier 4\nproducts", y=w3562) -> (x .and. y?=w3559:bool)
      n226 = case shown="True" w3559 {
        tunnel: w3558 -> [w3681 w3687]
        tunnel: w3587 -> [_ w3685]
        tunnel: [w3681 w3684] -> w3583
        tunnel: [0.0 w3683] -> w3575
        frame False {
        }
        frame True {
          n227 = Divide(x=100.0 ("y"), y=w3685) -> (x/y=w3682:dbl)
          n228 = Quotient & Remainder(x=w3687, y=w3682) -> (x-y*floor(x/y)=w3684:dbl, floor(x/y)=w3683:dbl)
        }
      }
      n229 = Compound Arithmetic op=ADD(w3674, w3675, w3548) -> (w3557:dbl)
      n230 = local write "Land conv mult"(w3671) -> ()
      n231 = Multiply(x=w3602, y=w3615) -> (x*y=w3614:dbl)
      n232 = case shown="True" w3644 {
        tunnel: w3602 -> [_ w3710]
        tunnel: [0 w3707] -> w3638
        tunnel: w3625 -> [_ w3705]
        frame False {
        }
        frame True {
          n233 = Negate(x=w3705) -> (-x=w3706:dbl)
          n234 = Divide(x=w3706, y=w3710) -> (x/y=w3709:dbl)
          n235 = Max & Min(x=w3709, y=20.0) -> (min(x,y)=w3707:dbl)  [unwired: 1 out]
        }
      }
      n236 = Add(x=w3642, y=w3638) -> (x+y=w3641:dbl)
      n237 = Multiply(x=w3557, y=w3645) -> (x*y=w3646:dbl)
      n238 = local read "EP"() -> (w3677:dbl)
      n239 = Multiply(x=w3621, y=w3602) -> (x*y=w3622:dbl)
      n240 = Subtract(x=w3575, y=w3576) -> (x-y=w3574:dbl)
      n241 = Add(x=w3574, y=w3582) -> (x+y=w3581:dbl)
      n242 = local read "SP"() -> (w3617:dbl)
      n243 = local write "Gov Economy\nbuildings mod"(1.0 ("y")) -> ()
      n244 = Add(x=w3620, y=w3622) -> (x+y=w3619:dbl)
      n245 = Multiply(x=w3637, y=w3619) -> (x*y=w3611:dbl)
      n246 = local write "Gov building\nupkeep mod"(w3550) -> ()
      n247 = Max & Min(x=0.0, y=w3646) -> (max(x,y)=w3653:dbl)  [unwired: 1 out]
      n248 = Add(x=w3614, y=w3616) -> (x+y=w3613:dbl)
      n249 = Compound Arithmetic op=MULTIPLY(w3637, w3612, w3613) -> (w3610:dbl)
      n250 = Max & Min(x=w3641, y=20.0) -> (min(x,y)=w3639:dbl)  [unwired: 1 out]
      n251 = Add(x=w3639, y=w3653) -> (x+y=w3609:dbl)
      n252 = Add(x=w3677, y=w3611) -> (x+y=w3676:dbl)
      n253 = Add(x=w3617, y=w3610) -> (x+y=w3647:dbl)
      n254 = local write "Tier 3\nproducts"(w3583) -> ()
      n255 = Max & Min(x=99.0, y=w3609) -> (min(x,y)=w3607:dbl)  [unwired: 1 out]
      n256 = local write "Tier 4\nproducts"(w3581) -> ()
      n257 = local write "Tier 1\nproducts"(w3593) -> ()
      n258 = local write "BP income"(w3623) -> ()
      n259 = local write "EP"(w3676) -> ()
      n260 = local write "SP"(w3647) -> ()
      n261 = local write "SP income"(w3610) -> ()
      n262 = local write "EP income"(w3611) -> ()
      n263 = local write "Dissent"(w3607) -> ()
      n264 = Max & Min(x=w3557, y=0.0) -> (max(x,y)=→"Base dissent":dbl)  [unwired: 1 out]
    }
    n265 = local read "Food consumption\nmultiplier"() -> (w1159:dbl)
    n266 = Greater Or Equal?(x=w270, y=w272) -> (x >= y?=w271:bool)
    n267 = local read "Aqueduct food multiplier"() -> (w722:dbl)
    n268 = Greater Or Equal?(x=w245, y=3) -> (x >= y?=w250:bool)
    n269 = Greater Or Equal?(x=w229, y=3) -> (x >= y?=w286:bool)
    n270 = And(x="Police force 0", y=w286) -> (x .and. y?=w230:bool)
    n271 = local write "Gold"(w641) -> ()
    n272 = local read "Military\nScience level"() -> (w1554:i32)
    n273 = Max & Min(x=w681, y=0.0) -> (max(x,y)=w676:dbl)  [unwired: 1 out]
    n274 = Greater Or Equal?(x=w678, y=w676) -> (x >= y?=w677:bool)
    n275 = Greater Or Equal?(x=w1670, y=w1668) -> (x >= y?=w1669:bool)
    n276 = Not Equal?(x=w249, y=w252) -> (x != y?=w247:bool)
    n277 = Greater Or Equal?(x=w1560, y=2) -> (x >= y?=w1558:bool)
    n278 = Not Equal?(x=w233, y=w234) -> (x != y?=w231:bool)
    n279 = And(x=w231, y=w230) -> (x .and. y?=w232:bool)
    n280 = Greater Or Equal?(x=w704, y=3) -> (x >= y?=w699:bool)
    n281 = Greater Or Equal?(x=w720, y=3) -> (x >= y?=w290:bool)
    n282 = And(x="Aqueduct\nlevel 0", y=w290) -> (x .and. y?=w719:bool)
    n283 = Greater Or Equal?(x=w1754, y=2) -> (x >= y?=w1748:bool)
    n284 = Greater Or Equal?(x=w1774, y=2) -> (x >= y?=w1768:bool)
    n285 = Greater Or Equal?(x=w1563, y=3) -> (x >= y?=w1569:bool)
    n286 = Greater Or Equal?(x=w1583, y=3) -> (x >= y?=w1589:bool)
    n287 = Greater Or Equal?(x=w1547, y=2) -> (x >= y?=w1546:bool)
    n288 = case shown="True" w232 {
      tunnel: w234 -> [_ w2161]
      frame False {
      }
      frame True {
        n289 = local write "Police force level"(w2161) -> ()
        n290 = local write "Police force base dissent mod"(0.0 ("Hut dissent add mod")) -> ()
        n291 = local write "Police force dissent mult"(1.0 ("Aqueduct dissent mod")) -> ()
        n292 = local write "Police force upkeep"(0.0 ("Hut non-land prod mod")) -> ()
      }
    }
    n293 = Not Equal?(x=w1749, y=w1746) -> (x != y?=w1751:bool)
    n294 = Not Equal?(x=w700, y=w697) -> (x != y?=w702:bool)
    n295 = Not Equal?(x=w1769, y=w1766) -> (x != y?=w1771:bool)
    n296 = Not Equal?(x=w1568, y=w1571) -> (x != y?=w1566:bool)
    n297 = Greater Or Equal?(x=w1541, y=2) -> (x >= y?=w1540:bool)
    n298 = Not Equal?(x=w716, y=w715) -> (x != y?=w718:bool)
    n299 = And(x=w718, y=w719) -> (x .and. y?=w717:bool)
    n300 = Not Equal?(x=w1588, y=w1591) -> (x != y?=w1586:bool)
    n301 = case shown="True" w717 {
      tunnel: w715 -> [_ w2840]
      frame False {
      }
      frame True {
        n302 = local write "Aqueduct level"(w2840) -> ()
        n303 = local write "Aqueduct food multiplier"(1.0 ("Hut dissent add mod")) -> ()
        n304 = local write "Aqueduct dissent mod"(1.0 ("Aqueduct dissent mod")) -> ()
        n305 = local write "Aqueduct upkeep"(0.0 ("Hut non-land prod mod")) -> ()
      }
    }
    n306 = case shown="True" w1179 {
      tunnel: w1177 -> [_ w3029]
      frame False {
      }
      frame True {
        n307 = local write "Food consumption\nmultiplier"(w3029) -> ()
        n308 = local write "Food dissent mod"(1.0 ("Taxes dissent add mod")) -> ()
      }
    }
    n309 = case shown="True" w1171 {
      tunnel: w1169 -> [_ w3031]
      frame False {
      }
      frame True {
        n310 = local write "Food consumption\nmultiplier"(w3031) -> ()
        n311 = local write "Food dissent mod"(0.7 ("Taxes dissent add mod")) -> ()
      }
    }
    n312 = And(x=w250, y=w271) -> (x .and. y?=w251:bool)
    n313 = And(x="Police force 2", y=w251) -> (x .and. y?=w246:bool)
    n314 = And(x=w247, y=w246) -> (x .and. y?=w248:bool)
    n315 = local read "Road land prod mod"() -> (w1732:dbl)
    n316 = local read "Gov food mult"() -> (w292:dbl)
    n317 = case shown="True" w248 {
      tunnel: w252 -> [_ w2179]
      tunnel: w272 -> [_ w2172]
      tunnel: w274 -> [_ w2171]
      frame False {
      }
      frame True {
        n318 = Add(x=w2172, y=w2171) -> (x+y=w2174:dbl)
        n319 = local read "Gold dbl"() -> (w2178:dbl)
        n320 = local write "Police force level"(w2179) -> ()
        n321 = local write "Police force base dissent mod"(20.0 ("Hut dissent add mod")) -> ()
        n322 = local write "Police force dissent mult"(0.74 ("Hut dissent add mod")) -> ()
        n323 = local write "Police force\ninvested points"(w2174) -> ()
        n324 = local write "Police force upkeep"(0.006 ("Hut non-land prod mod")) -> ()
        n325 = Subtract(x=w2178, y=w2172) -> (x-y=w2177:dbl)
        n326 = local write "Gold dbl"(w2177) -> ()
      }
    }
    n327 = Max & Min(x=w1489, y=0.1) -> (max(x,y)=w1488:dbl)  [unwired: 1 out]
    n328 = local read "People"() -> (w1160:i64)
    n329 = local read "hunting b"() -> (w293:dbl)
    n330 = local read "Biology\nlevel"() -> (w1792:i32)
    n331 = And(x=w699, y=w677) -> (x .and. y?=w698:bool)
    n332 = And(x="Aqueduct\nlevel 2", y=w698) -> (x .and. y?=w703:bool)
    n333 = And(x=w702, y=w703) -> (x .and. y?=w701:bool)
    n334 = Compound Arithmetic op=AND(w1569, w1546) -> (w1570:bool)
    n335 = And(x="Wall level 0", y=w1570) -> (x .and. y?=w1565:bool)
    n336 = And(x=w1566, y=w1565) -> (x .and. y?=w1567:bool)
    n337 = Compound Arithmetic op=AND(w1589, w1612, w1540) -> (w1590:bool)
    n338 = And(x="Wall level 2", y=w1590) -> (x .and. y?=w1585:bool)
    n339 = And(x=w1586, y=w1585) -> (x .and. y?=w1587:bool)
    n340 = local read "1-Dissent/100"() -> (w1957:dbl)
    n341 = local read "Road land prod mod"() -> (w158:dbl)
    n342 = case shown="True" w701 {
      tunnel: w697 -> [_ w2858]
      tunnel: w676 -> [_ w2851]
      tunnel: w674 -> [_ w2850]
      frame False {
      }
      frame True {
        n343 = local read "Build points"() -> (w2857:dbl)
        n344 = Add(x=w2851, y=w2850) -> (x+y=w2853:dbl)
        n345 = local write "Aqueduct level"(w2858) -> ()
        n346 = local write "Aqueduct food multiplier"(1.2 ("Hut dissent add mod")) -> ()
        n347 = local write "Aqueduct dissent mod"(0.96 ("Hut dissent add mod")) -> ()
        n348 = local write "Aqueduct\ninvested points"(w2853) -> ()
        n349 = local write "Aqueduct upkeep"(0.03 ("Hut non-land prod mod")) -> ()
        n350 = Subtract(x=w2857, y=w2851) -> (x-y=w2856:dbl)
        n351 = local write "Build points"(w2856) -> ()
      }
    }
    n352 = case shown="True" w1587 {
      tunnel: w1591 -> [_ w3198]
      tunnel: w1613 -> [_ w3194]
      tunnel: w1615 -> [_ w3193]
      frame False {
      }
      frame True {
        n353 = local read "Build points"() -> (w3197:dbl)
        n354 = Add(x=w3194, y=w3193) -> (x+y=w3195:dbl)
        n355 = local write "Wall warrior % equivalent"(4.0 ("Hut dissent add mod")) -> ()
        n356 = local write "Walls level"(w3198) -> ()
        n357 = local write "Wall dissent mod"(0.9 ("Hut non-land prod mod")) -> ()
        n358 = local write "Wall invested points"(w3195) -> ()
        n359 = local write "Wall upkeep"(0.006 ("Hut non-land prod mod")) -> ()
        n360 = Subtract(x=w3197, y=w3194) -> (x-y=w3196:dbl)
        n361 = local write "Build points"(w3196) -> ()
      }
    }
    n362 = case shown="True" w1567 {
      tunnel: w1571 -> [_ w3180]
      frame False {
      }
      frame True {
        n363 = local write "Wall warrior % equivalent"(0.0 ("Hut dissent add mod")) -> ()
        n364 = local write "Walls level"(w3180) -> ()
        n365 = local write "Wall dissent mod"(1.0 ("Hut non-land prod mod")) -> ()
        n366 = local write "Wall upkeep"(0.0 ("Hut non-land prod mod")) -> ()
      }
    }
    n367 = Reciprocal(x=w1488) -> (1/x=w1485:dbl)
    n368 = case shown="False" "Percentage or absolute" {
      frame False {
        n369 = Max & Min(x="%Scientists", y=0.0) -> (max(x,y)=w4000:dbl)  [unwired: 1 out]
        n370 = Max & Min(x="%Engineers", y=0.0) -> (max(x,y)=w3997:dbl)  [unwired: 1 out]
        n371 = Max & Min(x="%Crafters", y=0.0) -> (max(x,y)=w3994:dbl)  [unwired: 1 out]
        n372 = Max & Min(x="%Warriors", y=0.0) -> (max(x,y)=w4006:dbl)  [unwired: 1 out]
        n373 = Max & Min(x="%Builders", y=0.0) -> (max(x,y)=w4003:dbl)  [unwired: 1 out]
        n374 = Compound Arithmetic op=ADD(w4006, w4003, w4000, w3997, w3994) -> (w4009:dbl)
        n375 = Less Or Equal?(x=w4009, y=100.0) -> (x <= y?=w4011:bool)
        n376 = case shown="True" w4011 {
          tunnel: w4006 -> [_ w4039]
          tunnel: w4003 -> [_ w4038]
          tunnel: w4000 -> [_ w4037]
          tunnel: w3997 -> [_ w4036]
          tunnel: w3994 -> [_ w4035]
          frame False {
          }
          frame True {
            n377 = local read "People"() -> (w4031:i64)
            n378 = Divide(x=w4031, y=100.0) -> (x/y=w4033:dbl)
            n379 = local read "Max hunters"() -> (w4019:i32)
            n380 = Multiply(x=w4038, y=w4033) -> (x*y=w4026:dbl)
            n381 = Multiply(x=w4039, y=w4033) -> (x*y=w4016:dbl)
            n382 = Multiply(x=w4033, y=w4037) -> (x*y=w4025:dbl)
            n383 = Multiply(x=w4033, y=w4036) -> (x*y=w4024:dbl)
            n384 = Multiply(x=w4033, y=w4035) -> (x*y=w4028:dbl)
            n385 = local write "Scientists"(w4025) -> ()
            n386 = local write "Builders"(w4026) -> ()
            n387 = local write "Engineers"(w4024) -> ()
            n388 = local write "Crafters"(w4028) -> ()
            n389 = To Long Integer(number=w4024) -> (32bit integer=w4023:i32)
            n390 = To Long Integer(number=w4026) -> (32bit integer=w4021:i32)
            n391 = To Long Integer(number=w4025) -> (32bit integer=w4022:i32)
            n392 = To Long Integer(number=w4016) -> (32bit integer=w4012:i32)
            n393 = To Long Integer(number=w4028) -> (32bit integer=w4027:i32)
            n394 = Compound Arithmetic op=ADD(w4012, w4021, w4022, w4023, w4027) -> (w4032:i32)
            n395 = Subtract(x=w4031, y=w4032) -> (x-y=w4018:i64)
            n396 = Greater?(x=w4018, y=w4019) -> (0:w4020:bool)
            n397 = case shown="True" w4020 {
              tunnel: w4019 -> [_ w4044]
              tunnel: w4018 -> [w4041 w4043]
              tunnel: [w4041 w4044] -> w4013
              tunnel: [i64 0 w4042] -> w4014
              frame False {
              }
              frame True {
                n398 = Subtract(x=w4043, y=w4044) -> (x-y=w4042:i64)
              }
            }
            n399 = Divide(x=w4013, y=w4031) -> (x/y=w4030:dbl)
            n400 = Multiply(x=w4030, y=100.0) -> (x*y=→"%Hunters":dbl)
            n401 = Add(x=w4014, y=w4012) -> (x+y=w4015:i64)
            n402 = local write "Warriors"(w4015) -> ()
            n403 = local write "Hunters"(w4013) -> ()
          }
        }
      }
      frame True {
        n404 = local read "Unassigned workers"() -> (w4108:i32)
        n405 = local read "Unassigned workers"() -> (w4117:i32)
        n406 = local read "Unassigned workers"() -> (w4082:i32)
        n407 = local read "Unassigned workers"() -> (w4072:i32)
        n408 = local read "Unassigned workers"() -> (w4101:i32)
        n409 = local read "Unassigned workers"() -> (w4062:i32)
        n410 = local read "Hunters"() -> (w4085:i32)
        n411 = local read "Scientists"() -> (w4073:i32)
        n412 = local read "Engineers"() -> (w4063:i32)
        n413 = local read "Warriors"() -> (w4087:i32)
        n414 = local read "Builders"() -> (w4086:i32)
        n415 = local read "Crafters"() -> (w4053:i32)
        n416 = Greater Or Equal?(x="#Hunters", y=0.0) -> (x >= y?=w4114:bool)
        n417 = Greater Or Equal?(x="#Scientists", y=0.0) -> (x >= y?=w4079:bool)
        n418 = Greater Or Equal?(x="#Warriors", y=0.0) -> (x >= y?=w4105:bool)
        n419 = Greater Or Equal?(x="#Engineers", y=0.0) -> (x >= y?=w4069:bool)
        n420 = Greater Or Equal?(x="#Builders", y=0.0) -> (x >= y?=w4098:bool)
        n421 = Greater Or Equal?(x="#Merchants", y=0.0) -> (x >= y?=w4059:bool)
        n422 = Add(x=w4117, y=w4085) -> (x+y=w4116:i32)
        n423 = Add(x=w4082, y=w4073) -> (x+y=w4081:i32)
        n424 = Add(x=w4108, y=w4087) -> (x+y=w4107:i32)
        n425 = Add(x=w4072, y=w4063) -> (x+y=w4071:i32)
        n426 = Add(x=w4101, y=w4086) -> (x+y=w4100:i32)
        n427 = Add(x=w4062, y=w4053) -> (x+y=w4061:i32)
        n428 = Greater Or Equal?(x=w4116, y="#Hunters") -> (x >= y?=w4113:bool)
        n429 = Greater Or Equal?(x=w4081, y="#Scientists") -> (x >= y?=w4078:bool)
        n430 = Greater Or Equal?(x=w4107, y="#Warriors") -> (x >= y?=w4104:bool)
        n431 = Greater Or Equal?(x=w4071, y="#Engineers") -> (x >= y?=w4068:bool)
        n432 = Greater Or Equal?(x=w4100, y="#Builders") -> (x >= y?=w4097:bool)
        n433 = Greater Or Equal?(x=w4061, y="#Merchants") -> (x >= y?=w4058:bool)
        n434 = And(x=w4113, y=w4114) -> (x .and. y?=w4112:bool)
        n435 = And(x=w4078, y=w4079) -> (x .and. y?=w4077:bool)
        n436 = And(x=w4104, y=w4105) -> (x .and. y?=w4103:bool)
        n437 = And(x=w4068, y=w4069) -> (x .and. y?=w4067:bool)
        n438 = And(x=w4097, y=w4098) -> (x .and. y?=w4096:bool)
        n439 = And(x=w4058, y=w4059) -> (x .and. y?=w4057:bool)
        n440 = And(x=w4112, y="Assign Hunters") -> (x .and. y?=w4110:bool)
        n441 = And(x=w4077, y="Assign Scientist") -> (x .and. y?=w4075:bool)
        n442 = And(x=w4103, y="Assign Warrior") -> (x .and. y?=w4102:bool)
        n443 = And(x=w4067, y="Assign Engineer") -> (x .and. y?=w4065:bool)
        n444 = And(x=w4096, y="Assign Builder") -> (x .and. y?=w4095:bool)
        n445 = And(x=w4057, y="Assign Merchant") -> (x .and. y?=w4055:bool)
        n446 = case shown="True" w4110 {
          tunnel: "#Hunters" -> [_ w4129]
          tunnel: [w4128 w4129] -> w4093
          tunnel: w4085 -> [w4128 _]
          frame False {
          }
          frame True {
            n447 = local write "Hunters"(w4129) -> ()
          }
        }
        n448 = case shown="True" w4075 {
          tunnel: "#Scientists" -> [_ w4123]
          tunnel: [w4122 w4123] -> w4050
          tunnel: w4073 -> [w4122 _]
          frame False {
          }
          frame True {
            n449 = local write "Scientists"(w4123) -> ()
          }
        }
        n450 = case shown="True" w4102 {
          tunnel: "#Warriors" -> [_ w4127]
          tunnel: [w4126 w4127] -> w4088
          tunnel: w4087 -> [w4126 _]
          frame False {
          }
          frame True {
            n451 = local write "Warriors"(w4127) -> ()
          }
        }
        n452 = case shown="True" w4065 {
          tunnel: "#Engineers" -> [_ w4121]
          tunnel: [w4120 w4121] -> w4049
          tunnel: w4063 -> [w4120 _]
          frame False {
          }
          frame True {
            n453 = local write "Engineers"(w4121) -> ()
          }
        }
        n454 = case shown="True" w4095 {
          tunnel: "#Builders" -> [_ w4125]
          tunnel: [w4124 w4125] -> w4051
          tunnel: w4086 -> [w4124 _]
          frame False {
          }
          frame True {
            n455 = local write "Builders"(w4125) -> ()
          }
        }
        n456 = case shown="True" w4055 {
          tunnel: "#Merchants" -> [_ w4119]
          tunnel: [w4118 w4119] -> w4048
          tunnel: w4053 -> [w4118 _]
          frame False {
          }
          frame True {
            n457 = local write "Crafters"(w4119) -> ()
          }
        }
        n458 = local read "People"() -> (w4090:i64)
        n459 = Add(x=w4049, y=w4048) -> (x+y=w4047:dbl)
        n460 = Add(x=w4051, y=w4050) -> (x+y=w4046:dbl)
        n461 = Add(x=w4093, y=w4088) -> (x+y=w4092:dbl)
        n462 = Add(x=w4046, y=w4047) -> (x+y=w4045:dbl)
        n463 = Add(x=w4092, y=w4045) -> (x+y=w4091:dbl)
        n464 = Subtract(x=w4090, y=w4091) -> (x-y=w4089:dbl)
        n465 = local write "Unassigned workers"(w4089) -> ()
      }
    }
    n466 = Greater Or Equal?(x=w1554, y=2) -> (x >= y?=w1552:bool)
    n467 = Compound Arithmetic op=AND(w1748, w1669, w1552) -> (w1747:bool)
    n468 = And(x="Barracks\nlevel 2", y=w1747) -> (x .and. y?=w1752:bool)
    n469 = And(x=w1751, y=w1752) -> (x .and. y?=w1750:bool)
    n470 = case shown="True" w1750 {
      tunnel: w1746 -> [_ w3283]
      tunnel: w1668 -> [_ w3279]
      tunnel: w1666 -> [_ w3278]
      frame False {
      }
      frame True {
        n471 = local read "Build points"() -> (w3282:dbl)
        n472 = Add(x=w3279, y=w3278) -> (x+y=w3280:dbl)
        n473 = local write "Barracks level"(w3283) -> ()
        n474 = local write "Barracks military bonus"(1.2 ("Hut dissent add mod")) -> ()
        n475 = local write "Barracks\ninvested points"(w3280) -> ()
        n476 = local write "Barracks upkeep"(0.003 ("Hut non-land prod mod")) -> ()
        n477 = Subtract(x=w3282, y=w3279) -> (x-y=w3281:dbl)
        n478 = local write "Build points"(w3281) -> ()
      }
    }
    n479 = Compound Arithmetic op=AND(w1768, w1558) -> (w1767:bool)
    n480 = And(x="Barracks\nlevel 0", y=w1767) -> (x .and. y?=w1772:bool)
    n481 = And(x=w1771, y=w1772) -> (x .and. y?=w1770:bool)
    n482 = case shown="True" w1770 {
      tunnel: w1766 -> [_ w3267]
      frame False {
      }
      frame True {
        n483 = local write "Barracks level"(w3267) -> ()
        n484 = local write "Barracks military bonus"(1.0 ("Hut dissent add mod")) -> ()
        n485 = local write "Barracks upkeep"(0.0 ("Hut non-land prod mod")) -> ()
      }
    }
    n486 = Multiply(x=w1160, y=w1159) -> (x*y=w1157:dbl)
    n487 = local read "Military\nScience level"() -> (w1543:i32)
    n488 = local read "Permanent\nland"() -> (w1822:dbl)
    n489 = local read "Food"() -> (w2107:dbl)
    n490 = local read "Hunters"() -> (w1958:i32)
    n491 = Multiply(x=w293, y=w292) -> (x*y=w291:dbl)
    n492 = local read "Police force\ninvested points"() -> (w273:dbl)
    n493 = Multiply(x=w1485, y=1000.0) -> (x*y=w1487:dbl)
    n494 = local read "hunting a"() -> (w2106:dbl)
    n495 = Power Of X(1:1.05 ("x"), 2:w1792) -> (0:w724:dbl)
    n496 = Wait (ms)(milliseconds to wait=w1487) -> ()  [unwired: 1 out]
    n497 = local read "Wall invested points"() -> (w1614:dbl)
    n498 = local read "Police force\ninvested points"() -> (w281:dbl)
    n499 = local read "Aqueduct\ninvested points"() -> (w675:dbl)
    n500 = Greater Or Equal?(x=w1543, y=2) -> (x >= y?=w1544:bool)
    n501 = local read "Military\nScience level"() -> (w1556:i32)
    n502 = Compound Arithmetic op=MULTIPLY(w1958, w1732, w1957) -> (w1956:dbl)
    n503 = local read "Barracks\ninvested points"() -> (w1667:dbl)
    n504 = local read "Barracks\ninvested points"() -> (w1659:dbl)
    n505 = Multiply(x=w724, y=w722) -> (x*y=w723:dbl)
    n506 = local read "1-Dissent/100"() -> (w1963:dbl)
    n507 = local read "hunting a"() -> (w1964:dbl)
    n508 = local read "Wall invested points"() -> (w1622:dbl)
    n509 = local read "Aqueduct\ninvested points"() -> (w667:dbl)
    n510 = Multiply(x=w1822, y=w291) -> (x*y=w2122:dbl)
    n511 = local read "Governance\nlevel"() -> (w1162:i32)
    n512 = local read "Governance\nlevel"() -> (w260:i32)
    n513 = local read "Construction\nlevel"() -> (w1600:i32)
    n514 = Multiply(x=w2106, y=w1956) -> (x*y=w2115:dbl)
    n515 = local read "Food consumption\nmultiplier"() -> (w1167:dbl)
    n516 = Multiply(x=w2122, y=5) -> (x*y=w2120:dbl)
    n517 = local read "Gold dbl"() -> (w224:dbl)
    n518 = local read "Build points"() -> (w1605:dbl)
    n519 = local read "Construction\nlevel"() -> (w1737:i32)
    n520 = local read "Construction\nlevel"() -> (w689:i32)
    n521 = Subtract(x=100000 ("y"), y=w273) -> (x-y=w262:dbl)
    n522 = local read "Police force level"() -> (w238:i32)
    n523 = Multiply(x=w2115, y=0.1 ("x")) -> (x*y=w2125:dbl)
    n524 = Subtract(x=1000000 ("y"), y=w1614) -> (x-y=w1602:dbl)
    n525 = local read "Governance\nlevel"() -> (w242:i32)
    n526 = local read "Build points"() -> (w684:dbl)
    n527 = local read "Police force level"() -> (w256:i32)
    n528 = local read "Construction\nlevel"() -> (w1757:i32)
    n529 = local read "Wall warrior % equivalent"() -> (w1501:dbl)
    n530 = Compound Arithmetic op=MULTIPLY(w1964, w158, w1963) -> (w1962:dbl)
    n531 = Quotient & Remainder(x=w2120, y=w1962) -> (floor(x/y)=→"Max hunters":dbl)  [unwired: 1 out]
    n532 = local read "Barracks level"() -> (w1762:i32)
    n533 = local read "Construction\nlevel"() -> (w1580:i32)
    n534 = local read "Gold dbl"() -> (w275:dbl)
    n535 = local read "Build points"() -> (w1676:dbl)
    n536 = local read "Build points"() -> (w1665:dbl)
    n537 = local read "Build points"() -> (w1616:dbl)
    n538 = Subtract(x=500000 ("y"), y=w675) -> (x-y=w687:dbl)
    n539 = Subtract(x=10000000 ("y"), y=w281) -> (x-y=w278:dbl)
    n540 = local read "Barracks level"() -> (w1742:i32)
    n541 = Divide(x=w2125, y=w1822) -> (x/y=w2124:dbl)
    n542 = local read "Walls level"() -> (w1575:i32)
    n543 = local read "Construction\nlevel"() -> (w707:i32)
    n544 = local read "Walls level"() -> (w1595:i32)
    n545 = local read "Aqueduct level"() -> (w711:i32)
    n546 = Subtract(x=100000 ("y"), y=w1667) -> (x-y=w1679:dbl)
    n547 = Subtract(x=1000000 ("y"), y=w1659) -> (x-y=w1662:dbl)
    n548 = local read "Build points"() -> (w673:dbl)
    n549 = Greater Or Equal?(x=w1737, y=2) -> (x >= y?=w1743:bool)
    n550 = Subtract(x=10000000 ("y"), y=w1622) -> (x-y=w1619:dbl)
    n551 = local read "Aqueduct level"() -> (w693:i32)
    n552 = Max & Min(x=w262, y=0.0) -> (max(x,y)=w266:dbl)  [unwired: 1 out]
    n553 = Greater Or Equal?(x=w224, y=w266) -> (x >= y?=w265:bool)
    n554 = Max & Min(x=w1602, y=0.0) -> (max(x,y)=w1607:dbl)  [unwired: 1 out]
    n555 = Multiply(x=100, y="# people") -> (x*y=w2093:i32)
    n556 = Subtract(x=w291, y=w2124) -> (x-y=w2123:dbl)
    n557 = local read "Conquered\nland"() -> (w1821:dbl)
    n558 = Greater Or Equal?(x=w1605, y=w1607) -> (x >= y?=w1606:bool)
    n559 = Multiply(x=w2115, y=w2123) -> (x*y=w2114:dbl)
    n560 = Subtract(x=5000000 ("y"), y=w667) -> (x-y=w670:dbl)
    n561 = local read "Farming level"() -> (w227:i32)
    n562 = local read "Trading level"() -> (w1730:i32)
    n563 = Max & Min(x=w687, y=0.0) -> (max(x,y)=w682:dbl)  [unwired: 1 out]
    n564 = Max & Min(x=w278, y=0.0) -> (max(x,y)=w280:dbl)  [unwired: 1 out]
    n565 = Greater Or Equal?(x=w1556, y=2) -> (x >= y?=w1555:bool)
    n566 = Greater Or Equal?(x=w684, y=w682) -> (x >= y?=w683:bool)
    n567 = Greater Or Equal?(x=w275, y=w280) -> (x >= y?=w279:bool)
    n568 = Max & Min(x=w1679, y=0.0) -> (max(x,y)=w1674:dbl)  [unwired: 1 out]
    n569 = Max & Min(x=w1662, y=0.0) -> (max(x,y)=w1660:dbl)  [unwired: 1 out]
    n570 = local read "Road land prod mod"() -> (w1731:dbl)
    n571 = Greater Or Equal?(x=w242, y=3) -> (x >= y?=w237:bool)
    n572 = Max & Min(x=w1619, y=0.0) -> (max(x,y)=w1621:dbl)  [unwired: 1 out]
    n573 = Greater Or Equal?(x=w1676, y=w1674) -> (x >= y?=w1675:bool)
    n574 = Greater Or Equal?(x=w1665, y=w1660) -> (x >= y?=w1661:bool)
    n575 = Greater Or Equal?(x=w1162, y=2) -> (x >= y?=w1186:bool)
    n576 = Greater Or Equal?(x=w1757, y=2) -> (x >= y?=w1763:bool)
    n577 = Greater Or Equal?(x=w1616, y=w1621) -> (x >= y?=w1620:bool)
    n578 = And(x="Higher food\nconsumption", y=w1186) -> (x .and. y?=w1164:bool)
    n579 = Greater Or Equal?(x=w260, y=3) -> (x >= y?=w255:bool)
    n580 = And(x=w255, y=w265) -> (x .and. y?=w254:bool)
    n581 = And(x="Police force 1", y=w254) -> (x .and. y?=w259:bool)
    n582 = Greater Or Equal?(x=w1580, y=3) -> (x >= y?=w1574:bool)
    n583 = Max & Min(x=w670, y=0.0) -> (max(x,y)=w668:dbl)  [unwired: 1 out]
    n584 = Greater Or Equal?(x=w1600, y=3) -> (x >= y?=w1594:bool)
    n585 = Compound Arithmetic op=AND(w1594, w1606, w1544) -> (w1593:bool)
    n586 = And(x="Wall level 1", y=w1593) -> (x .and. y?=w1598:bool)
    n587 = Not Equal?(x=w238, y=w235) -> (x != y?=w240:bool)
    n588 = And(x=w237, y=w279) -> (x .and. y?=w236:bool)
    n589 = And(x="Police force 3", y=w236) -> (x .and. y?=w241:bool)
    n590 = And(x=w240, y=w241) -> (x .and. y?=w239:bool)
    n591 = Greater Or Equal?(x=w673, y=w668) -> (x >= y?=w669:bool)
    n592 = Not Equal?(x=w1167, y=w1168) -> (x != y?=w1165:bool)
    n593 = And(x=w1165, y=w1164) -> (x .and. y?=w1166:bool)
    n594 = Not Equal?(x=w1762, y=w1765) -> (x != y?=w1760:bool)
    n595 = Greater Or Equal?(x=w707, y=3) -> (x >= y?=w712:bool)
    n596 = Not Equal?(x=w1575, y=w1572) -> (x != y?=w1577:bool)
    n597 = Not Equal?(x=w256, y=w253) -> (x != y?=w258:bool)
    n598 = And(x=w258, y=w259) -> (x .and. y?=w257:bool)
    n599 = Not Equal?(x=w1742, y=w1745) -> (x != y?=w1740:bool)
    n600 = Not Equal?(x=w1595, y=w1592) -> (x != y?=w1597:bool)
    n601 = And(x=w1597, y=w1598) -> (x .and. y?=w1596:bool)
    n602 = Greater Or Equal?(x=w689, y=3) -> (x >= y?=w694:bool)
    n603 = And(x=w694, y=w683) -> (x .and. y?=w695:bool)
    n604 = And(x="Aqueduct\nlevel 1", y=w695) -> (x .and. y?=w690:bool)
    n605 = case shown="True" w239 {
      tunnel: w235 -> [_ w2170]
      tunnel: w280 -> [_ w2163]
      tunnel: w281 -> [_ w2162]
      frame False {
      }
      frame True {
        n606 = Add(x=w2163, y=w2162) -> (x+y=w2164:dbl)
        n607 = local read "Gold dbl"() -> (w2169:dbl)
        n608 = local write "Police force base dissent mod"(50.0 ("Hut dissent add mod")) -> ()
        n609 = local write "Police force level"(w2170) -> ()
        n610 = local write "Police force dissent mult"(0.6 ("Hut dissent add mod")) -> ()
        n611 = local write "Police force\ninvested points"(w2164) -> ()
        n612 = local write "Police force upkeep"(0.02 ("Hut non-land prod mod")) -> ()
        n613 = Subtract(x=w2169, y=w2163) -> (x-y=w2168:dbl)
        n614 = local write "Gold dbl"(w2168) -> ()
      }
    }
    n615 = Greater?(x="# people", y=0.0) -> (0:w846:bool)
    n616 = Compound Arithmetic op=AND(w1743, w1675, w1555) -> (w1744:bool)
    n617 = And(x="Barracks\nlevel 1", y=w1744) -> (x .and. y?=w1739:bool)
    n618 = And(x=w1740, y=w1739) -> (x .and. y?=w1741:bool)
    n619 = Not Equal?(x=w711, y=w714) -> (x != y?=w709:bool)
    n620 = And(x=w712, y=w669) -> (x .and. y?=w713:bool)
    n621 = And(x="Aqueduct\nlevel 3", y=w713) -> (x .and. y?=w708:bool)
    n622 = And(x=w709, y=w708) -> (x .and. y?=w710:bool)
    n623 = Not Equal?(x=w693, y=w696) -> (x != y?=w691:bool)
    n624 = And(x=w691, y=w690) -> (x .and. y?=w692:bool)
    n625 = case shown="True" w710 {
      tunnel: w714 -> [_ w2849]
      tunnel: w668 -> [_ w2842]
      tunnel: w667 -> [_ w2841]
      frame False {
      }
      frame True {
        n626 = local read "Build points"() -> (w2848:dbl)
        n627 = Add(x=w2842, y=w2841) -> (x+y=w2843:dbl)
        n628 = local write "Aqueduct level"(w2849) -> ()
        n629 = local write "Aqueduct food multiplier"(1.3 ("Hut dissent add mod")) -> ()
        n630 = local write "Aqueduct dissent mod"(0.94 ("Hut dissent add mod")) -> ()
        n631 = local write "Aqueduct\ninvested points"(w2843) -> ()
        n632 = local write "Aqueduct upkeep"(0.15 ("Hut non-land prod mod")) -> ()
        n633 = Subtract(x=w2848, y=w2842) -> (x-y=w2847:dbl)
        n634 = local write "Build points"(w2847) -> ()
      }
    }
    n635 = Multiply(x=w227, y=0.25) -> (x*y=w226:dbl)
    n636 = case shown="True" w1166 {
      tunnel: w1168 -> [_ w3033]
      frame False {
      }
      frame True {
        n637 = local write "Food consumption\nmultiplier"(w3033) -> ()
        n638 = local write "Food dissent mod"(0.85 ("Taxes dissent add mod")) -> ()
      }
    }
    n639 = local read "Military\nScience level"() -> (w1550:i32)
    n640 = local read "1-Dissent/100"() -> (w1960:dbl)
    n641 = local read "Military\nScience level"() -> (w1539:i32)
    n642 = Multiply(x=w1730, y=0.25) -> (x*y=w1729:dbl)
    n643 = Increment(x=w226) -> (x+1=w1789:dbl)
    n644 = case shown="True" w257 {
      tunnel: w253 -> [_ w2188]
      tunnel: w273 -> [_ w2183]
      tunnel: w266 -> [_ w2181]
      tunnel: w224 -> [_ w2180]
      frame False {
      }
      frame True {
        n645 = local write "Police force level"(w2188) -> ()
        n646 = Add(x=w2181, y=w2183) -> (x+y=w2182:dbl)
        n647 = local write "Police force base dissent mod"(5.0 ("Hut dissent add mod")) -> ()
        n648 = local write "Police force\ninvested points"(w2182) -> ()
        n649 = local write "Police force dissent mult"(0.87 ("Hut dissent add mod")) -> ()
        n650 = local write "Police force upkeep"(0.002 ("Hut non-land prod mod")) -> ()
        n651 = Subtract(x=w2180, y=w2181) -> (x-y=w2187:dbl)
        n652 = local write "Gold dbl"(w2187) -> ()
      }
    }
    n653 = case shown="True" w1741 {
      tunnel: w1745 -> [_ w3291]
      tunnel: w1667 -> [_ w3288]
      tunnel: w1674 -> [_ w3286]
      frame False {
      }
      frame True {
        n654 = local read "Build points"() -> (w3290:dbl)
        n655 = Add(x=w3286, y=w3288) -> (x+y=w3287:dbl)
        n656 = local write "Barracks level"(w3291) -> ()
        n657 = local write "Barracks military bonus"(1.1 ("Hut dissent add mod")) -> ()
        n658 = local write "Barracks\ninvested points"(w3287) -> ()
        n659 = local write "Barracks upkeep"(0.001 ("Hut non-land prod mod")) -> ()
        n660 = Subtract(x=w3290, y=w3286) -> (x-y=w3289:dbl)
        n661 = local write "Build points"(w3289) -> ()
      }
    }
    n662 = case shown="True" w1596 {
      tunnel: w1592 -> [_ w3207]
      tunnel: w1614 -> [_ w3204]
      tunnel: w1607 -> [_ w3202]
      frame False {
      }
      frame True {
        n663 = local read "Build points"() -> (w3206:dbl)
        n664 = Add(x=w3202, y=w3204) -> (x+y=w3203:dbl)
        n665 = local write "Walls level"(w3207) -> ()
        n666 = local write "Wall warrior % equivalent"(2.0 ("Hut dissent add mod")) -> ()
        n667 = local write "Wall invested points"(w3203) -> ()
        n668 = local write "Wall dissent mod"(0.95 ("Hut non-land prod mod")) -> ()
        n669 = Subtract(x=w3206, y=w3202) -> (x-y=w3205:dbl)
        n670 = local write "Wall upkeep"(0.002 ("Hut non-land prod mod")) -> ()
        n671 = local write "Build points"(w3205) -> ()
      }
    }
    n672 = local read "Warriors"() -> (w1504:i32)
    n673 = Increment(x=w1729) -> (x+1=w1790:dbl)
    n674 = local read "warrior a"() -> (w1961:dbl)
    n675 = case shown="True" w692 {
      tunnel: w696 -> [_ w2867]
      tunnel: w675 -> [_ w2861]
      tunnel: w682 -> [_ w2859]
      frame False {
      }
      frame True {
        n676 = local read "Build points"() -> (w2866:dbl)
        n677 = Add(x=w2859, y=w2861) -> (x+y=w2860:dbl)
        n678 = local write "Aqueduct level"(w2867) -> ()
        n679 = local write "Aqueduct food multiplier"(1.1 ("Hut dissent add mod")) -> ()
        n680 = local write "Aqueduct\ninvested points"(w2860) -> ()
        n681 = local write "Aqueduct dissent mod"(0.98 ("Hut dissent add mod")) -> ()
        n682 = local write "Aqueduct upkeep"(0.01 ("Hut non-land prod mod")) -> ()
        n683 = Subtract(x=w2866, y=w2859) -> (x-y=w2865:dbl)
        n684 = local write "Build points"(w2865) -> ()
      }
    }
    n685 = Compound Arithmetic op=MULTIPLY(w1821, w1789, w1790) -> (w1156:dbl)
    n686 = Add(x=w2114, y=w1156) -> (x+y=w1155:dbl)
    n687 = Multiply(x=w723, y=w1155) -> (x*y=w1154:dbl)
    n688 = Subtract(x=w1154, y=w1157) -> (x-y=w1158:dbl)
    "Food/s" <- w1158
    n689 = Add(x=w2107, y=w1158) -> (x+y=w2092:dbl)
    n690 = Greater?(x=w2092, y=w2093) -> (0:w2096:bool)
    n691 = Compound Arithmetic op=AND(w2096, w846, "Increase\nPopulation") -> (w2095:bool)
    n692 = case shown="False" w2095 {
      tunnel: w1160 -> [_ w4173]
      tunnel: w2093 -> [_ w4171]
      tunnel: w2092 -> [w4155 w4170]
      tunnel: [w4154 w4169] -> w2090
      tunnel: "# people" -> [_ w4168]
      frame False {
        n693 = Less?(x=w4155, y=-100.0) -> (x < y?=w4157:bool)
        n694 = case shown="True" w4157 {
          tunnel: w4155 -> [w4158 w4162]
          tunnel: [w4158 w4159] -> w4154
          frame False {
          }
          frame True {
            n695 = local read "People"() -> (w4160:i64)
            n696 = Quotient & Remainder(x=w4162, y=100.0) -> (floor(x/y)=w4166:dbl)  [unwired: 1 out]
            n697 = Increment(x=w4166) -> (x+1=w4163:dbl)
            n698 = Add(x=w4160, y=w4163) -> (x+y=w4165:dbl)
            n699 = local write "People"(w4165) -> ()
            n700 = Multiply(x=w4163, y=-50.0) -> (x*y=w4161:dbl)
            n701 = Add(x=w4161, y=w4162) -> (x+y=w4159:dbl)
          }
        }
      }
      frame True {
        n702 = Add(x=w4173, y=w4168) -> (x+y=w4172:i64)
        n703 = Subtract(x=w4170, y=w4171) -> (x-y=w4169:dbl)
        n704 = local write "People"(w4172) -> ()
      }
    }
    n705 = Compound Arithmetic op=MULTIPLY(w1160, 0.01 ("value"), w1501) -> (w1500:dbl)
    n706 = local write "Food income"(w1154) -> ()
    n707 = Greater Or Equal?(x=w1539, y=2) -> (x >= y?=w1537:bool)
    n708 = Compound Arithmetic op=AND(w1574, w1620, w1537) -> (w1573:bool)
    n709 = And(x="Wall level 3", y=w1573) -> (x .and. y?=w1578:bool)
    n710 = And(x=w1577, y=w1578) -> (x .and. y?=w1576:bool)
    n711 = case shown="True" w1576 {
      tunnel: w1572 -> [_ w3189]
      tunnel: w1621 -> [_ w3185]
      tunnel: w1622 -> [_ w3184]
      frame False {
      }
      frame True {
        n712 = local read "Build points"() -> (w3188:dbl)
        n713 = Add(x=w3185, y=w3184) -> (x+y=w3186:dbl)
        n714 = local write "Walls level"(w3189) -> ()
        n715 = local write "Wall warrior % equivalent"(6.0 ("Hut dissent add mod")) -> ()
        n716 = local write "Wall invested points"(w3186) -> ()
        n717 = local write "Wall dissent mod"(0.85 ("Hut non-land prod mod")) -> ()
        n718 = Subtract(x=w3188, y=w3185) -> (x-y=w3187:dbl)
        n719 = local write "Wall upkeep"(0.02 ("Hut non-land prod mod")) -> ()
        n720 = local write "Build points"(w3187) -> ()
      }
    }
    n721 = Add(x=w1500, y=w1504) -> (x+y=w1503:dbl)
    n722 = Compound Arithmetic op=MULTIPLY(w1961, w1731, w1960) -> (w1959:dbl)
    n723 = local read "Housing type"() -> (w400:string)
    n724 = Multiply(x=w1503, y=w1959) -> (x*y=w2119:dbl)
    n725 = Greater Or Equal?(x=w1550, y=2) -> (x >= y?=w1549:bool)
    n726 = Compound Arithmetic op=AND(w1763, w1661, w1549) -> (w1764:bool)
    n727 = And(x="Barracks\nlevel 3", y=w1764) -> (x .and. y?=w1759:bool)
    n728 = And(x=w1760, y=w1759) -> (x .and. y?=w1761:bool)
    n729 = case shown="True" w1761 {
      tunnel: w1765 -> [_ w3275]
      tunnel: w1660 -> [_ w3271]
      tunnel: w1659 -> [_ w3270]
      frame False {
      }
      frame True {
        n730 = local read "Build points"() -> (w3274:dbl)
        n731 = Add(x=w3271, y=w3270) -> (x+y=w3272:dbl)
        n732 = local write "Barracks level"(w3275) -> ()
        n733 = local write "Barracks\ninvested points"(w3272) -> ()
        n734 = local write "Barracks military bonus"(1.3 ("Hut dissent add mod")) -> ()
        n735 = local write "Barracks upkeep"(0.01 ("Hut non-land prod mod")) -> ()
        n736 = Subtract(x=w3274, y=w3271) -> (x-y=w3273:dbl)
        n737 = local write "Build points"(w3273) -> ()
      }
    }
    n738 = local read "School invested points"() -> (w1341:dbl)
    n739 = local read "Construction\nlevel"() -> (w1373:i32)
    n740 = local read "Road type"() -> (w371:string)
    n741 = case shown="\"Concrete Housing\"" w400 {
      tunnel: "Hut level 0" -> [w2503 w2598 w2693]
      tunnel: "Hut level 1" -> [w2502 w2597 w2692]
      tunnel: "Hut level 2" -> [w2501 w2596 w2691]
      tunnel: "Hut level 3" -> [w2500 w2595 w2690]
      frame "Hut", Default {
        w2525 = 3 ("y")
        w2536 = 2 ("y")
        w2547 = 0 ("y")
        w2548 = 1 ("y")
        # "Constructions initial build"
        n742 = local read "Hut invested points"() -> (w2513:dbl)
        n743 = local read "Construction\nlevel"() -> (w2542:i32)
        n744 = local read "Construction\nlevel"() -> (w2532:i32)
        n745 = local read "Build points"() -> (w2515:dbl)
        n746 = local read "Hut level"() -> (w2546:i32)
        n747 = local read "Hut level"() -> (w2535:i32)
        n748 = Subtract(x=30000 ("y"), y=w2513) -> (x-y=w2518:dbl)
        n749 = Max & Min(x=w2518, y=0.0) -> (max(x,y)=w2512:dbl)  [unwired: 1 out]
        n750 = Greater Or Equal?(x=w2542, y=1) -> (x >= y?=w2540:bool)
        n751 = Greater Or Equal?(x=w2515, y=w2512) -> (x >= y?=w2514:bool)
        n752 = And(x=w2503, y=w2540) -> (x .and. y?=w2543:bool)
        n753 = Greater Or Equal?(x=w2532, y=1) -> (x >= y?=w2537:bool)
        n754 = Not Equal?(x=w2546, y=w2547) -> (x != y?=w2544:bool)
        n755 = And(x=w2544, y=w2543) -> (x .and. y?=w2545:bool)
        n756 = Not Equal?(x=w2535, y=w2536) -> (x != y?=w2533:bool)
        n757 = Compound Arithmetic op=AND(w2533, w2501, w2537, w2514) -> (w2534:bool)
        n758 = local read "Gov populist\nbuildings mod"() -> (w2506:dbl)
        n759 = case shown="True" w2534 {
          tunnel: w2536 -> [_ w2578]
          tunnel: w2513 -> [_ w2573]
          tunnel: w2512 -> [_ w2572]
          tunnel: w2506 -> [_ w2568]
          frame False {
          }
          frame True {
            n760 = local read "Build points"() -> (w2577:dbl)
            n761 = Multiply(x=w2568, y=0.2) -> (x*y=w2570:dbl)
            n762 = Add(x=w2572, y=w2573) -> (x+y=w2574:dbl)
            n763 = local write "Hut level"(w2578) -> ()
            n764 = Increment(x=w2570) -> (x+1=w2571:dbl)
            n765 = local write "Hut upkeep"(0.03 ("Hut dissent add mod")) -> ()
            n766 = local write "Hut non-land prod mod"(w2571) -> ()
            n767 = Subtract(x=w2577, y=w2572) -> (x-y=w2576:dbl)
            n768 = local write "Hut invested points"(w2574) -> ()
            n769 = local write "Hut dissent mod"(0.9 ("Hut dissent add mod")) -> ()
            n770 = local write "Build points"(w2576) -> ()
          }
        }
        n771 = case shown="True" w2545 {
          tunnel: w2547 -> [_ w2582]
          frame False {
          }
          frame True {
            n772 = local write "Hut non-land prod mod"(1.0 ("Hut non-land prod mod")) -> ()
            n773 = local write "Hut dissent mod"(1.0 ("Hut dissent add mod")) -> ()
            n774 = local write "Hut level"(w2582) -> ()
            n775 = local write "Hut upkeep"(0.0 ("Hut dissent add mod")) -> ()
          }
        }
        n776 = local read "Hut invested points"() -> (w2519:dbl)
        n777 = local read "Hut invested points"() -> (w2505:dbl)
        n778 = local read "Construction\nlevel"() -> (w2553:i32)
        n779 = local read "Construction\nlevel"() -> (w2529:i32)
        n780 = local read "Build points"() -> (w2549:dbl)
        n781 = local read "Hut level"() -> (w2550:i32)
        n782 = local read "Build points"() -> (w2511:dbl)
        n783 = Subtract(x=10000 ("y"), y=w2519) -> (x-y=w2521:dbl)
        n784 = local read "Hut level"() -> (w2526:i32)
        n785 = Subtract(x=150000 ("y"), y=w2505) -> (x-y=w2509:dbl)
        n786 = Max & Min(x=w2521, y=0.0) -> (max(x,y)=w2520:dbl)  [unwired: 1 out]
        n787 = Max & Min(x=w2509, y=0.0) -> (max(x,y)=w2507:dbl)  [unwired: 1 out]
        n788 = Greater Or Equal?(x=w2549, y=w2520) -> (x >= y?=w2538:bool)
        n789 = Greater Or Equal?(x=w2553, y=1) -> (x >= y?=w2539:bool)
        n790 = Greater Or Equal?(x=w2511, y=w2507) -> (x >= y?=w2508:bool)
        n791 = Greater Or Equal?(x=w2529, y=1) -> (x >= y?=w2524:bool)
        n792 = Not Equal?(x=w2550, y=w2548) -> (x != y?=w2552:bool)
        n793 = Compound Arithmetic op=AND(w2552, w2502, w2539, w2538) -> (w2551:bool)
        n794 = Not Equal?(x=w2526, y=w2525) -> (x != y?=w2528:bool)
        n795 = Compound Arithmetic op=AND(w2528, w2500, w2524, w2508) -> (w2527:bool)
        n796 = case shown="True" w2551 {
          tunnel: w2548 -> [_ w2594]
          tunnel: w2520 -> [_ w2589]
          tunnel: w2519 -> [_ w2590]
          tunnel: w2506 -> [_ w2584]
          frame False {
          }
          frame True {
            n797 = local read "Build points"() -> (w2593:dbl)
            n798 = Multiply(x=0.1, y=w2584) -> (x*y=w2585:dbl)
            n799 = local write "Hut level"(w2594) -> ()
            n800 = Add(x=w2589, y=w2590) -> (x+y=w2588:dbl)
            n801 = Increment(x=w2585) -> (x+1=w2587:dbl)
            n802 = local write "Hut upkeep"(0.01 ("Hut dissent add mod")) -> ()
            n803 = Subtract(x=w2593, y=w2589) -> (x-y=w2592:dbl)
            n804 = local write "Hut non-land prod mod"(w2587) -> ()
            n805 = local write "Build points"(w2592) -> ()
            n806 = local write "Hut invested points"(w2588) -> ()
            n807 = local write "Hut dissent mod"(0.95 ("Hut dissent add mod")) -> ()
          }
        }
        n808 = case shown="True" w2527 {
          tunnel: w2525 -> [_ w2566]
          tunnel: w2505 -> [_ w2561]
          tunnel: w2507 -> [_ w2560]
          tunnel: w2506 -> [_ w2556]
          frame False {
          }
          frame True {
            n809 = Multiply(x=w2556, y=0.3) -> (x*y=w2558:dbl)
            n810 = Increment(x=w2558) -> (x+1=w2559:dbl)
            n811 = local read "Build points"() -> (w2565:dbl)
            n812 = Add(x=w2560, y=w2561) -> (x+y=w2562:dbl)
            n813 = local write "Hut non-land prod mod"(w2559) -> ()
            n814 = local write "Hut level"(w2566) -> ()
            n815 = local write "Hut upkeep"(0.15 ("Hut dissent add mod")) -> ()
            n816 = Subtract(x=w2565, y=w2560) -> (x-y=w2564:dbl)
            n817 = local write "Hut invested points"(w2562) -> ()
            n818 = local write "Build points"(w2564) -> ()
            n819 = local write "Hut dissent mod"(0.85 ("Hut dissent add mod")) -> ()
          }
        }
      }
      frame "Brick House" {
        w2620 = 3 ("y")
        w2631 = 2 ("y")
        w2642 = 0 ("y")
        w2643 = 1 ("y")
        # "Constructions initial build"
        n820 = local read "Hut invested points"() -> (w2608:dbl)
        n821 = local read "Construction\nlevel"() -> (w2637:i32)
        n822 = local read "Construction\nlevel"() -> (w2627:i32)
        n823 = local read "Build points"() -> (w2610:dbl)
        n824 = local read "Hut level"() -> (w2641:i32)
        n825 = local read "Hut level"() -> (w2630:i32)
        n826 = Subtract(x=300000 ("y"), y=w2608) -> (x-y=w2613:dbl)
        n827 = Max & Min(x=w2613, y=0.0) -> (max(x,y)=w2607:dbl)  [unwired: 1 out]
        n828 = Greater Or Equal?(x=w2637, y=1) -> (x >= y?=w2635:bool)
        n829 = Greater Or Equal?(x=w2610, y=w2607) -> (x >= y?=w2609:bool)
        n830 = And(x=w2598, y=w2635) -> (x .and. y?=w2638:bool)
        n831 = Greater Or Equal?(x=w2627, y=1) -> (x >= y?=w2632:bool)
        n832 = Not Equal?(x=w2641, y=w2642) -> (x != y?=w2639:bool)
        n833 = And(x=w2639, y=w2638) -> (x .and. y?=w2640:bool)
        n834 = Not Equal?(x=w2630, y=w2631) -> (x != y?=w2628:bool)
        n835 = Compound Arithmetic op=AND(w2628, w2596, w2632, w2609) -> (w2629:bool)
        n836 = local read "Gov populist\nbuildings mod"() -> (w2601:dbl)
        n837 = case shown="True" w2629 {
          tunnel: w2631 -> [_ w2673]
          tunnel: w2608 -> [_ w2668]
          tunnel: w2607 -> [_ w2667]
          tunnel: w2601 -> [_ w2663]
          frame False {
          }
          frame True {
            n838 = local read "Build points"() -> (w2672:dbl)
            n839 = Multiply(x=w2663, y=0.24) -> (x*y=w2665:dbl)
            n840 = Add(x=w2667, y=w2668) -> (x+y=w2669:dbl)
            n841 = local write "Hut level"(w2673) -> ()
            n842 = Increment(x=w2665) -> (x+1=w2666:dbl)
            n843 = local write "Hut upkeep"(0.045 ("Hut dissent add mod")) -> ()
            n844 = local write "Hut non-land prod mod"(w2666) -> ()
            n845 = Subtract(x=w2672, y=w2667) -> (x-y=w2671:dbl)
            n846 = local write "Hut invested points"(w2669) -> ()
            n847 = local write "Hut dissent mod"(0.86 ("Hut dissent add mod")) -> ()
            n848 = local write "Build points"(w2671) -> ()
          }
        }
        n849 = case shown="True" w2640 {
          tunnel: w2642 -> [_ w2677]
          frame False {
          }
          frame True {
            n850 = local write "Hut non-land prod mod"(1.0 ("Hut non-land prod mod")) -> ()
            n851 = local write "Hut dissent mod"(1.0 ("Hut dissent add mod")) -> ()
            n852 = local write "Hut level"(w2677) -> ()
            n853 = local write "Hut upkeep"(0.0 ("Hut dissent add mod")) -> ()
          }
        }
        n854 = local read "Hut invested points"() -> (w2614:dbl)
        n855 = local read "Hut invested points"() -> (w2600:dbl)
        n856 = local read "Construction\nlevel"() -> (w2648:i32)
        n857 = local read "Construction\nlevel"() -> (w2624:i32)
        n858 = local read "Build points"() -> (w2644:dbl)
        n859 = local read "Hut level"() -> (w2645:i32)
        n860 = local read "Build points"() -> (w2606:dbl)
        n861 = Subtract(x=100000 ("y"), y=w2614) -> (x-y=w2616:dbl)
        n862 = local read "Hut level"() -> (w2621:i32)
        n863 = Subtract(x=1500000 ("y"), y=w2600) -> (x-y=w2604:dbl)
        n864 = Max & Min(x=w2616, y=0.0) -> (max(x,y)=w2615:dbl)  [unwired: 1 out]
        n865 = Max & Min(x=w2604, y=0.0) -> (max(x,y)=w2602:dbl)  [unwired: 1 out]
        n866 = Greater Or Equal?(x=w2644, y=w2615) -> (x >= y?=w2633:bool)
        n867 = Greater Or Equal?(x=w2648, y=1) -> (x >= y?=w2634:bool)
        n868 = Greater Or Equal?(x=w2606, y=w2602) -> (x >= y?=w2603:bool)
        n869 = Greater Or Equal?(x=w2624, y=1) -> (x >= y?=w2619:bool)
        n870 = Not Equal?(x=w2645, y=w2643) -> (x != y?=w2647:bool)
        n871 = Compound Arithmetic op=AND(w2647, w2597, w2634, w2633) -> (w2646:bool)
        n872 = Not Equal?(x=w2621, y=w2620) -> (x != y?=w2623:bool)
        n873 = Compound Arithmetic op=AND(w2623, w2595, w2619, w2603) -> (w2622:bool)
        n874 = case shown="True" w2646 {
          tunnel: w2643 -> [_ w2689]
          tunnel: w2615 -> [_ w2684]
          tunnel: w2614 -> [_ w2685]
          tunnel: w2601 -> [_ w2679]
          frame False {
          }
          frame True {
            n875 = local read "Build points"() -> (w2688:dbl)
            n876 = Multiply(x=0.12, y=w2679) -> (x*y=w2680:dbl)
            n877 = local write "Hut level"(w2689) -> ()
            n878 = Add(x=w2684, y=w2685) -> (x+y=w2683:dbl)
            n879 = Increment(x=w2680) -> (x+1=w2682:dbl)
            n880 = local write "Hut upkeep"(0.015 ("Hut dissent add mod")) -> ()
            n881 = Subtract(x=w2688, y=w2684) -> (x-y=w2687:dbl)
            n882 = local write "Hut non-land prod mod"(w2682) -> ()
            n883 = local write "Build points"(w2687) -> ()
            n884 = local write "Hut invested points"(w2683) -> ()
            n885 = local write "Hut dissent mod"(0.93 ("Hut dissent add mod")) -> ()
          }
        }
        n886 = case shown="True" w2622 {
          tunnel: w2620 -> [_ w2661]
          tunnel: w2600 -> [_ w2656]
          tunnel: w2602 -> [_ w2655]
          tunnel: w2601 -> [_ w2651]
          frame False {
          }
          frame True {
            n887 = Multiply(x=w2651, y=0.36) -> (x*y=w2653:dbl)
            n888 = Increment(x=w2653) -> (x+1=w2654:dbl)
            n889 = local read "Build points"() -> (w2660:dbl)
            n890 = Add(x=w2655, y=w2656) -> (x+y=w2657:dbl)
            n891 = local write "Hut non-land prod mod"(w2654) -> ()
            n892 = local write "Hut level"(w2661) -> ()
            n893 = local write "Hut upkeep"(0.225 ("Hut dissent add mod")) -> ()
            n894 = Subtract(x=w2660, y=w2655) -> (x-y=w2659:dbl)
            n895 = local write "Hut invested points"(w2657) -> ()
            n896 = local write "Build points"(w2659) -> ()
            n897 = local write "Hut dissent mod"(0.79 ("Hut dissent add mod")) -> ()
          }
        }
      }
      frame "Concrete Housing" {
        w2715 = 3 ("y")
        w2726 = 2 ("y")
        w2737 = 0 ("y")
        w2738 = 1 ("y")
        # "Constructions initial build"
        n898 = local read "Hut invested points"() -> (w2703:dbl)
        n899 = local read "Construction\nlevel"() -> (w2732:i32)
        n900 = local read "Construction\nlevel"() -> (w2722:i32)
        n901 = local read "Build points"() -> (w2705:dbl)
        n902 = local read "Hut level"() -> (w2736:i32)
        n903 = local read "Hut level"() -> (w2725:i32)
        n904 = Subtract(x=30000 ("y"), y=w2703) -> (x-y=w2708:dbl)
        n905 = Max & Min(x=w2708, y=0.0) -> (max(x,y)=w2702:dbl)  [unwired: 1 out]
        n906 = Greater Or Equal?(x=w2732, y=1) -> (x >= y?=w2730:bool)
        n907 = Greater Or Equal?(x=w2705, y=w2702) -> (x >= y?=w2704:bool)
        n908 = And(x=w2693, y=w2730) -> (x .and. y?=w2733:bool)
        n909 = Greater Or Equal?(x=w2722, y=1) -> (x >= y?=w2727:bool)
        n910 = Not Equal?(x=w2736, y=w2737) -> (x != y?=w2734:bool)
        n911 = And(x=w2734, y=w2733) -> (x .and. y?=w2735:bool)
        n912 = Not Equal?(x=w2725, y=w2726) -> (x != y?=w2723:bool)
        n913 = Compound Arithmetic op=AND(w2723, w2691, w2727, w2704) -> (w2724:bool)
        n914 = local read "Gov populist\nbuildings mod"() -> (w2696:dbl)
        n915 = case shown="True" w2724 {
          tunnel: w2726 -> [_ w2768]
          tunnel: w2703 -> [_ w2763]
          tunnel: w2702 -> [_ w2762]
          tunnel: w2696 -> [_ w2758]
          frame False {
          }
          frame True {
            n916 = local read "Build points"() -> (w2767:dbl)
            n917 = Multiply(x=w2758, y=0.26) -> (x*y=w2760:dbl)
            n918 = Add(x=w2762, y=w2763) -> (x+y=w2764:dbl)
            n919 = local write "Hut level"(w2768) -> ()
            n920 = Increment(x=w2760) -> (x+1=w2761:dbl)
            n921 = local write "Hut upkeep"(0.03 ("Hut dissent add mod")) -> ()
            n922 = local write "Hut non-land prod mod"(w2761) -> ()
            n923 = Subtract(x=w2767, y=w2762) -> (x-y=w2766:dbl)
            n924 = local write "Hut invested points"(w2764) -> ()
            n925 = local write "Hut dissent mod"(0.84 ("Hut dissent add mod")) -> ()
            n926 = local write "Build points"(w2766) -> ()
          }
        }
        n927 = case shown="True" w2735 {
          tunnel: w2737 -> [_ w2772]
          frame False {
          }
          frame True {
            n928 = local write "Hut non-land prod mod"(1.0 ("Hut non-land prod mod")) -> ()
            n929 = local write "Hut dissent mod"(1.0 ("Hut dissent add mod")) -> ()
            n930 = local write "Hut level"(w2772) -> ()
            n931 = local write "Hut upkeep"(0.0 ("Hut dissent add mod")) -> ()
          }
        }
        n932 = local read "Hut invested points"() -> (w2709:dbl)
        n933 = local read "Hut invested points"() -> (w2695:dbl)
        n934 = local read "Construction\nlevel"() -> (w2743:i32)
        n935 = local read "Construction\nlevel"() -> (w2719:i32)
        n936 = local read "Build points"() -> (w2739:dbl)
        n937 = local read "Hut level"() -> (w2740:i32)
        n938 = local read "Build points"() -> (w2701:dbl)
        n939 = Subtract(x=10000 ("y"), y=w2709) -> (x-y=w2711:dbl)
        n940 = local read "Hut level"() -> (w2716:i32)
        n941 = Subtract(x=150000 ("y"), y=w2695) -> (x-y=w2699:dbl)
        n942 = Max & Min(x=w2711, y=0.0) -> (max(x,y)=w2710:dbl)  [unwired: 1 out]
        n943 = Max & Min(x=w2699, y=0.0) -> (max(x,y)=w2697:dbl)  [unwired: 1 out]
        n944 = Greater Or Equal?(x=w2739, y=w2710) -> (x >= y?=w2728:bool)
        n945 = Greater Or Equal?(x=w2743, y=1) -> (x >= y?=w2729:bool)
        n946 = Greater Or Equal?(x=w2701, y=w2697) -> (x >= y?=w2698:bool)
        n947 = Greater Or Equal?(x=w2719, y=1) -> (x >= y?=w2714:bool)
        n948 = Not Equal?(x=w2740, y=w2738) -> (x != y?=w2742:bool)
        n949 = Compound Arithmetic op=AND(w2742, w2692, w2729, w2728) -> (w2741:bool)
        n950 = Not Equal?(x=w2716, y=w2715) -> (x != y?=w2718:bool)
        n951 = Compound Arithmetic op=AND(w2718, w2690, w2714, w2698) -> (w2717:bool)
        n952 = case shown="True" w2741 {
          tunnel: w2738 -> [_ w2784]
          tunnel: w2710 -> [_ w2779]
          tunnel: w2709 -> [_ w2780]
          tunnel: w2696 -> [_ w2774]
          frame False {
          }
          frame True {
            n953 = local read "Build points"() -> (w2783:dbl)
            n954 = Multiply(x=0.13, y=w2774) -> (x*y=w2775:dbl)
            n955 = local write "Hut level"(w2784) -> ()
            n956 = Add(x=w2779, y=w2780) -> (x+y=w2778:dbl)
            n957 = Increment(x=w2775) -> (x+1=w2777:dbl)
            n958 = local write "Hut upkeep"(0.01 ("Hut dissent add mod")) -> ()
            n959 = Subtract(x=w2783, y=w2779) -> (x-y=w2782:dbl)
            n960 = local write "Hut non-land prod mod"(w2777) -> ()
            n961 = local write "Build points"(w2782) -> ()
            n962 = local write "Hut invested points"(w2778) -> ()
            n963 = local write "Hut dissent mod"(0.92 ("Hut dissent add mod")) -> ()
          }
        }
        n964 = case shown="True" w2717 {
          tunnel: w2715 -> [_ w2756]
          tunnel: w2695 -> [_ w2751]
          tunnel: w2697 -> [_ w2750]
          tunnel: w2696 -> [_ w2746]
          frame False {
          }
          frame True {
            n965 = Multiply(x=w2746, y=0.39) -> (x*y=w2748:dbl)
            n966 = Increment(x=w2748) -> (x+1=w2749:dbl)
            n967 = local read "Build points"() -> (w2755:dbl)
            n968 = Add(x=w2750, y=w2751) -> (x+y=w2752:dbl)
            n969 = local write "Hut non-land prod mod"(w2749) -> ()
            n970 = local write "Hut level"(w2756) -> ()
            n971 = local write "Hut upkeep"(0.15 ("Hut dissent add mod")) -> ()
            n972 = Subtract(x=w2755, y=w2750) -> (x-y=w2754:dbl)
            n973 = local write "Hut invested points"(w2752) -> ()
            n974 = local write "Build points"(w2754) -> ()
            n975 = local write "Hut dissent mod"(0.76 ("Hut dissent add mod")) -> ()
          }
        }
      }
    }
    n976 = local read "Construction\nlevel"() -> (w1393:i32)
    n977 = local read "School level"() -> (w1388:i32)
    n978 = local read "Temple\ninvested points"() -> (w772:dbl)
    n979 = for {
      tunnel: w1735 -> [w3393] mode=indexing
      w3292 = 1.0 ("value")
      # "Science prices"
      # "Construction upkeep"
      n980 = local read "# of level 1 sciences"() -> (w3349:i32)
      n981 = local read "Aqueduct upkeep"() -> (w3358:dbl)
      n982 = local read "# of level 2 sciences"() -> (w3343:i32)
      n983 = local read "# of level 3 sciences"() -> (w3341:i32)
      n984 = local read "Harbor upkeep"() -> (w3363:dbl)
      n985 = local read "Road upkeep"() -> (w3396:dbl)
      n986 = local read "Market upkeep"() -> (w3296:dbl)
      n987 = local read "Police force upkeep"() -> (w3297:dbl)
      n988 = local read "Barracks upkeep"() -> (w3392:dbl)
      n989 = local read "Hut upkeep"() -> (w3397:dbl)
      n990 = local read "Construction\nlevel"() -> (w3295:i32)
      n991 = local read "University upkeep"() -> (w3373:dbl)
      n992 = local read "School upkeep"() -> (w3374:dbl)
      n993 = local read "Temple upkeep"() -> (w3360:dbl)
      n994 = local read "Wall upkeep"() -> (w3391:dbl)
      n995 = local read "Build points"() -> (w3403:dbl)
      n996 = Compound Arithmetic op=ADD(w3397, w3296, w3396, w3363, w3358) -> (w3395:dbl)
      n997 = Power Of 2(x=w3349) -> (2^x=w3348:dbl)
      n998 = Power Of 2(x=w3343) -> (2^x=w3344:dbl)
      n999 = Power Of 2(x=w3341) -> (2^x=w3340:dbl)
      n1000 = Compound Arithmetic op=ADD(w3392, w3391, w3374, w3373, w3360, w3297) -> (w3390:dbl)
      n1001 = Multiply(x=w3393, y=w3395) -> (x*y=w3394:dbl)
      n1002 = Power Of X(1:0.9 ("x"), 2:w3295) -> (0:w3293:dbl)
      n1003 = Multiply(x=w3393, y=w3390) -> (x*y=w3389:dbl)
      n1004 = local read "Government"() -> (w3304:string)
      n1005 = Multiply(x=w3348, y=1000.0) -> (x*y=→"Level 1 science price":dbl)
      n1006 = Multiply(x=w3344, y=10000.0) -> (x*y=→"Level 2 science price":dbl)
      n1007 = Multiply(x=w3340, y=100000.0) -> (x*y=→"Level 3 science price":dbl)
      n1008 = Compound Arithmetic op=MULTIPLY(w3394, w3293, w3292) -> (w3382:dbl)
      n1009 = Subtract(x=w3403, y=w3382) -> (x-y=w3399:dbl)
      n1010 = local read "Gold dbl"() -> (w3388:dbl)
      n1011 = Compound Arithmetic op=MULTIPLY(w3293, w3292, w3389) -> (w3386:dbl)
      n1012 = local write "Build points"(w3399) -> ()
      n1013 = local write "BP upkeep"(w3382) -> ()
      n1014 = local write "Gold upkeep"(w3386) -> ()
      n1015 = Subtract(x=w3388, y=w3386) -> (x-y=w3387:dbl)
      n1016 = case shown="\"Theocracy 2\"" w3304 {
        tunnel: [0.0 ("x") 1.0 ("x") 1.0 ("x")] -> w3303
        frame "False", Default {
        }
        frame "Theocracy" {
        }
        frame "Theocracy 2" {
        }
      }
      n1017 = local read "# of level 6 sciences"() -> (w3327:i32)
      n1018 = local read "# of level 5 sciences"() -> (w3333:i32)
      n1019 = local write "Gold dbl"(w3387) -> ()
      n1020 = local read "# of level 4 sciences"() -> (w3335:i32)
      n1021 = local read "Temple dissent mod"() -> (w3306:dbl)
      n1022 = local read "Police force dissent mult"() -> (w3298:dbl)
      n1023 = local read "Dissent mult per\nmilitary building"() -> (w3352:dbl)
      n1024 = local read "School dissent mod"() -> (w3381:dbl)
      n1025 = local read "Governance\nlevel"() -> (w3355:i32)
      n1026 = local read "Barracks level"() -> (w3378:i32)
      n1027 = local read "Harbor level"() -> (w3362:i32)
      n1028 = local read "Walls level"() -> (w3379:i32)
      n1029 = local read "Gov elitist\nbuildings mod"() -> (w3376:dbl)
      n1030 = local read "Aqueduct dissent mod"() -> (w3357:dbl)
      n1031 = local read "University dissent mod"() -> (w3309:dbl)
      n1032 = local read "Hut dissent mod"() -> (w3398:dbl)
      n1033 = local read "Gov populist\nbuildings mod"() -> (w3385:dbl)
      n1034 = Add(x=1.0, y=w3303) -> (x+y=w3302:dbl)
      n1035 = Power Of 2(x=w3327) -> (2^x=w3328:dbl)
      n1036 = Power Of 2(x=w3333) -> (2^x=w3332:dbl)
      n1037 = local read "Medicine dissent mod"() -> (w3369:dbl)
      n1038 = Subtract(x=1.0, y=w3306) -> (x-y=w3308:dbl)
      n1039 = Power Of 2(x=w3335) -> (2^x=w3336:dbl)
      n1040 = Multiply(x=w3328, y=100000000.0) -> (x*y=→"Level 6 science price":dbl)
      n1041 = Multiply(x=w3332, y=10000000.0) -> (x*y=→"Level 5 science price":dbl)
      n1042 = Multiply(x=w3308, y=w3302) -> (x*y=w3300:dbl)
      n1043 = Multiply(x=w3336, y=1000000.0) -> (x*y=→"Level 4 science price":dbl)
      n1044 = Subtract(x=1.0, y=w3300) -> (x-y=w3299:dbl)
      n1045 = local read "Wall dissent mod"() -> (w3380:dbl)
      n1046 = Compound Arithmetic op=ADD(w3379, w3378, w3362) -> (w3351:i32)
      n1047 = Compound Arithmetic op=MULTIPLY(w3309, w3299) -> (w3377:dbl)
      n1048 = Compound Arithmetic op=MULTIPLY(w3398, w3381) -> (w3356:dbl)
      n1049 = Power Of X(1:0.95 ("x"), 2:w3355) -> (0:w3353:dbl)
      n1050 = Power Of X(1:w3377, 2:w3376) -> (0:w3375:dbl)
      n1051 = Power Of X(1:w3352, 2:w3351) -> (0:w3350:dbl)
      n1052 = Power Of X(1:w3356, 2:w3385) -> (0:w3384:dbl)
      n1053 = local read "# of level 10 sciences"() -> (w3311:i32)
      n1054 = local read "# of level 8 sciences"() -> (w3319:i32)
      n1055 = local read "# of level 9 sciences"() -> (w3317:i32)
      n1056 = local read "# of level 7 sciences"() -> (w3325:i32)
      n1057 = local read "Writing level"() -> (w3365:i32)
      n1058 = local read "Temple SP/EP multiplier"() -> (w3359:dbl)
      n1059 = local read "School SP/EP multiplier"() -> (w3368:dbl)
      n1060 = local read "Trading level no mod"() -> (w3402:i32)
      n1061 = local read "Road trade modifier"() -> (w3401:dbl)
      n1062 = local read "Food dissent mod"() -> (w3372:dbl)
      n1063 = Compound Arithmetic op=MULTIPLY(w3384, w3369, w3372, w3353, w3357, w3380, w3350, w3375, w3298) -> (w3383:dbl)
      n1064 = local read "Hut non-land prod mod"() -> (w3371:dbl)
      n1065 = local read "Harbor level"() -> (w3361:i32)
      n1066 = Power Of 2(x=w3311) -> (2^x=w3312:dbl)
      n1067 = Power Of 2(x=w3319) -> (2^x=w3320:dbl)
      n1068 = Power Of 2(x=w3317) -> (2^x=w3316:dbl)
      n1069 = local write "Dissent \nmultiplication\nmodifier"(w3383) -> ()
      n1070 = Power Of 2(x=w3325) -> (2^x=w3324:dbl)
      n1071 = Power Of X(1:1.1 ("x"), 2:w3365) -> (0:w3364:dbl)
      n1072 = Multiply(x=w3312, y=1000000000000.0) -> (x*y=→"Level 10 science price":dbl)
      n1073 = Multiply(x=w3320, y=10000000000.0) -> (x*y=→"Level 8 science price":dbl)
      n1074 = Multiply(x=w3316, y=100000000000.0) -> (x*y=→"Level 9 science price":dbl)
      n1075 = Multiply(x=w3324, y=1000000000.0) -> (x*y=→"Level 7 science price":dbl)
      n1076 = Compound Arithmetic op=ADD(w3402, w3401, w3361) -> (w3400:dbl)
      n1077 = Compound Arithmetic op=MULTIPLY(w3368, w3359, w3364) -> (w3367:dbl)
      n1078 = Compound Arithmetic op=ADD(w3371) -> (w3370:dbl)
      n1079 = local write "Non-land production multiplier"(w3370) -> ()
      n1080 = local write "SP/EP multiplier"(w3367) -> ()
      n1081 = local write "Trading level"(w3400) -> ()
    }
    n1082 = local read "Build points"() -> (w1345:dbl)
    n1083 = local read "Governance\nlevel"() -> (w1396:i32)
    n1084 = local read "Market\ninvested points"() -> (w179:dbl)
    n1085 = local read "School level"() -> (w1368:i32)
    n1086 = Subtract(x=600000 ("y"), y=w1341) -> (x-y=w1348:dbl)
    n1087 = local read "Governance\nlevel"() -> (w1402:i32)
    n1088 = local read "Barracks military bonus"() -> (w1561:dbl)
    n1089 = local read "Harbor military mod"() -> (w786:dbl)
    n1090 = local read "warrior c"() -> (w2102:dbl)
    n1091 = local read "Harbor\ninvested points"() -> (w798:dbl)
    n1092 = local read "Warrior b Gov mult"() -> (w1887:dbl)
    n1093 = local read "Economics\nlevel"() -> (w1644:i32)
    n1094 = local read "Construction\nlevel"() -> (w168:i32)
    n1095 = Max & Min(x=w1348, y=0.0) -> (max(x,y)=w1343:dbl)  [unwired: 1 out]
    n1096 = Multiply(x=w2090, y=0.999) -> (x*y=w2089:dbl)
    n1097 = Add(x=w2119, y=50.0) -> (x+y=w2117:dbl)
    n1098 = Greater Or Equal?(x=w1393, y=2) -> (x >= y?=w1387:bool)
    n1099 = Greater Or Equal?(x=w1345, y=w1343) -> (x >= y?=w1344:bool)
    n1100 = local read "Economics\nlevel"() -> (w209:i32)
    n1101 = local read "Construction\nlevel"() -> (w726:i32)
    n1102 = local read "Brick house\nunlocked"() -> (w391:bool)
    n1103 = local read "Taxation\nlevel"() -> (w1633:dbl)
    n1104 = local read "Economics\nlevel"() -> (w1628:i32)
    n1105 = local read "Construction\nlevel"() -> (w742:i32)
    n1106 = local read "Brick house\nunlocked"() -> (w359:bool)
    n1107 = local read "Taxation\nlevel"() -> (w1649:dbl)
    n1108 = Greater Or Equal?(x=w1373, y=3) -> (x >= y?=w1367:bool)
    n1109 = local write "Food"(w2089) -> ()
    n1110 = Not Equal?(x=w1388, y=w1385) -> (x != y?=w1390:bool)
    n1111 = Greater Or Equal?(x=w1396, y=2) -> (x >= y?=w1397:bool)
    n1112 = Reciprocal(x=w2102) -> (1/x=w643:dbl)
    n1113 = Greater Or Equal?(x=w1402, y=2) -> (x >= y?=w1403:bool)
    n1114 = local read "Build points"() -> (w183:dbl)
    n1115 = Not Equal?(x=w1368, y=w1365) -> (x != y?=w1370:bool)
    n1116 = local read "Market level"() -> (w205:i32)
    n1117 = local read "Market level"() -> (w221:i32)
    n1118 = local read "Conquered\nland"() -> (w637:dbl)
    n1119 = local read "warrior b"() -> (w1888:dbl)
    n1120 = Subtract(x=15000000 ("y"), y=w179) -> (x-y=w186:dbl)
    n1121 = local read "Temple level"() -> (w746:i32)
    n1122 = Power Of X(1:w2117, 2:w643) -> (0:w2116:dbl)
    n1123 = local read "Gold dbl"() -> (w768:dbl)
    n1124 = local read "Boat level"() -> (w828:i32)
    n1125 = local read "Temple level"() -> (w730:i32)
    n1126 = Subtract(x=10000 ("y"), y=w772) -> (x-y=w765:dbl)
    n1127 = Compound Arithmetic op=AND(w1387, w1397) -> (w1386:bool)
    n1128 = And(x="School\nlevel 0", y=w1386) -> (x .and. y?=w1391:bool)
    n1129 = And(x=w1390, y=w1391) -> (x .and. y?=w1389:bool)
    n1130 = case shown="True" w1389 {
      tunnel: w1385 -> [_ w3101]
      frame False {
      }
      frame True {
        n1131 = local write "School engineer equivalent"(0.0 ("Hut dissent add mod")) -> ()
        n1132 = local write "School level"(w3101) -> ()
        n1133 = local write "School SP/EP multiplier"(1.0 ("Hut non-land prod mod")) -> ()
        n1134 = local write "School dissent mod"(1.0 ("Hut non-land prod mod")) -> ()
        n1135 = local write "School upkeep"(0.0 ("Hut non-land prod mod")) -> ()
      }
    }
    n1136 = local read "Build points"() -> (w802:dbl)
    n1137 = Power Of X(1:50.0 ("x"), 2:w643) -> (0:w642:dbl)
    n1138 = local read "Harbor level"() -> (w824:i32)
    n1139 = local read "Harbor level"() -> (w840:i32)
    n1140 = Compound Arithmetic op=AND(w1367, w1344, w1403) -> (w1366:bool)
    n1141 = And(x="School\nlevel 2", y=w1366) -> (x .and. y?=w1371:bool)
    n1142 = And(x=w1370, y=w1371) -> (x .and. y?=w1369:bool)
    n1143 = case shown="\"Paved tar roads\"" w371 {
      tunnel: "Road level 0" -> [w2212 w2307 w2402]
      tunnel: "Road level 1" -> [w2211 w2306 w2401]
      tunnel: "Road level 2" -> [w2210 w2305 w2400]
      tunnel: "Road level 3" -> [w2209 w2304 w2399]
      frame "Stone roads", Default {
        w2219 = 0 ("y")
        w2220 = 3 ("y")
        w2237 = 2 ("y")
        w2238 = 1 ("y")
        n1144 = local read "Road invested points"() -> (w2260:dbl)
        n1145 = local read "Construction\nlevel"() -> (w2230:i32)
        n1146 = local read "Build points"() -> (w2256:dbl)
        n1147 = local read "Construction\nlevel"() -> (w2214:i32)
        n1148 = local read "Road level"() -> (w2234:i32)
        n1149 = local read "Road level"() -> (w2218:i32)
        n1150 = Subtract(x=150000 ("y"), y=w2260) -> (x-y=w2253:dbl)
        n1151 = Max & Min(x=w2253, y=0.0) -> (max(x,y)=w2258:dbl)  [unwired: 1 out]
        n1152 = Greater Or Equal?(x=w2256, y=w2258) -> (x >= y?=w2257:bool)
        n1153 = Greater Or Equal?(x=w2230, y=1) -> (x >= y?=w2235:bool)
        n1154 = Greater Or Equal?(x=w2214, y=1) -> (x >= y?=w2208:bool)
        n1155 = And(x=w2212, y=w2208) -> (x .and. y?=w2215:bool)
        n1156 = Not Equal?(x=w2234, y=w2237) -> (x != y?=w2232:bool)
        n1157 = Not Equal?(x=w2218, y=w2219) -> (x != y?=w2216:bool)
        n1158 = And(x=w2216, y=w2215) -> (x .and. y?=w2217:bool)
        n1159 = case shown="True" w2217 {
          tunnel: w2219 -> [_ w2272]
          frame False {
          }
          frame True {
            n1160 = local write "Road level"(w2272) -> ()
            n1161 = local write "Road expansion bonus"(0.0 ("Hut dissent add mod")) -> ()
            n1162 = local write "Road land prod mod"(1.0 ("Hut dissent add mod")) -> ()
            n1163 = local write "Road trade modifier"(0.0 ("Hut dissent add mod")) -> ()
            n1164 = local write "Road upkeep"(0.0 ("Hut non-land prod mod")) -> ()
          }
        }
        n1165 = And(x=w2235, y=w2257) -> (x .and. y?=w2236:bool)
        n1166 = And(x=w2210, y=w2236) -> (x .and. y?=w2231:bool)
        n1167 = And(x=w2232, y=w2231) -> (x .and. y?=w2233:bool)
        n1168 = case shown="True" w2233 {
          tunnel: w2237 -> [_ w2292]
          tunnel: w2258 -> [_ w2285]
          tunnel: w2260 -> [_ w2284]
          frame False {
          }
          frame True {
            n1169 = local read "Build points"() -> (w2291:dbl)
            n1170 = Add(x=w2285, y=w2284) -> (x+y=w2287:dbl)
            n1171 = local write "Road level"(w2292) -> ()
            n1172 = local write "Road expansion bonus"(0.5 ("Hut dissent add mod")) -> ()
            n1173 = local write "Road land prod mod"(1.2 ("Hut dissent add mod")) -> ()
            n1174 = local write "Road invested points"(w2287) -> ()
            n1175 = local write "Road upkeep"(0.06 ("Hut non-land prod mod")) -> ()
            n1176 = local write "Road trade modifier"(2.0 ("Hut non-land prod mod")) -> ()
            n1177 = Subtract(x=w2291, y=w2285) -> (x-y=w2290:dbl)
            n1178 = local write "Build points"(w2290) -> ()
          }
        }
        n1179 = local read "Road invested points"() -> (w2259:dbl)
        n1180 = local read "Road invested points"() -> (w2267:dbl)
        n1181 = local read "Construction\nlevel"() -> (w2245:i32)
        n1182 = local read "Build points"() -> (w2250:dbl)
        n1183 = Subtract(x=50000 ("y"), y=w2259) -> (x-y=w2247:dbl)
        n1184 = local read "Construction\nlevel"() -> (w2227:i32)
        n1185 = local read "Build points"() -> (w2261:dbl)
        n1186 = local read "Road level"() -> (w2223:i32)
        n1187 = local read "Road level"() -> (w2241:i32)
        n1188 = Max & Min(x=w2247, y=0.0) -> (max(x,y)=w2252:dbl)  [unwired: 1 out]
        n1189 = Subtract(x=500000 ("y"), y=w2267) -> (x-y=w2264:dbl)
        n1190 = Greater Or Equal?(x=w2250, y=w2252) -> (x >= y?=w2251:bool)
        n1191 = Max & Min(x=w2264, y=0.0) -> (max(x,y)=w2266:dbl)  [unwired: 1 out]
        n1192 = Greater Or Equal?(x=w2227, y=1) -> (x >= y?=w2222:bool)
        n1193 = Greater Or Equal?(x=w2261, y=w2266) -> (x >= y?=w2265:bool)
        n1194 = Greater Or Equal?(x=w2245, y=1) -> (x >= y?=w2240:bool)
        n1195 = And(x=w2240, y=w2251) -> (x .and. y?=w2239:bool)
        n1196 = And(x=w2211, y=w2239) -> (x .and. y?=w2244:bool)
        n1197 = Not Equal?(x=w2223, y=w2220) -> (x != y?=w2225:bool)
        n1198 = And(x=w2222, y=w2265) -> (x .and. y?=w2221:bool)
        n1199 = And(x=w2209, y=w2221) -> (x .and. y?=w2226:bool)
        n1200 = And(x=w2225, y=w2226) -> (x .and. y?=w2224:bool)
        n1201 = Not Equal?(x=w2241, y=w2238) -> (x != y?=w2243:bool)
        n1202 = And(x=w2243, y=w2244) -> (x .and. y?=w2242:bool)
        n1203 = case shown="True" w2224 {
          tunnel: w2220 -> [_ w2282]
          tunnel: w2266 -> [_ w2275]
          tunnel: w2267 -> [_ w2274]
          frame False {
          }
          frame True {
            n1204 = local read "Build points"() -> (w2281:dbl)
            n1205 = Add(x=w2275, y=w2274) -> (x+y=w2276:dbl)
            n1206 = local write "Road level"(w2282) -> ()
            n1207 = local write "Road expansion bonus"(1.0 ("Hut dissent add mod")) -> ()
            n1208 = local write "Road land prod mod"(1.3 ("Hut dissent add mod")) -> ()
            n1209 = local write "Road invested points"(w2276) -> ()
            n1210 = local write "Road upkeep"(0.2 ("Hut non-land prod mod")) -> ()
            n1211 = local write "Road trade modifier"(3.0 ("Hut non-land prod mod")) -> ()
            n1212 = Subtract(x=w2281, y=w2275) -> (x-y=w2280:dbl)
            n1213 = local write "Build points"(w2280) -> ()
          }
        }
        n1214 = case shown="True" w2242 {
          tunnel: w2238 -> [_ w2302]
          tunnel: w2259 -> [_ w2296]
          tunnel: w2252 -> [_ w2294]
          frame False {
          }
          frame True {
            n1215 = local read "Build points"() -> (w2301:dbl)
            n1216 = Add(x=w2294, y=w2296) -> (x+y=w2295:dbl)
            n1217 = local write "Road level"(w2302) -> ()
            n1218 = local write "Road expansion bonus"(0.2 ("Hut dissent add mod")) -> ()
            n1219 = local write "Road land prod mod"(1.1 ("Hut dissent add mod")) -> ()
            n1220 = local write "Road trade modifier"(1.0 ("Hut dissent add mod")) -> ()
            n1221 = local write "Road invested points"(w2295) -> ()
            n1222 = local write "Road upkeep"(0.02 ("Hut non-land prod mod")) -> ()
            n1223 = Subtract(x=w2301, y=w2294) -> (x-y=w2300:dbl)
            n1224 = local write "Build points"(w2300) -> ()
          }
        }
      }
      frame "Multilayer stone roads" {
        w2314 = 0 ("y")
        w2315 = 3 ("y")
        w2332 = 2 ("y")
        w2333 = 1 ("y")
        n1225 = local read "Road invested points"() -> (w2355:dbl)
        n1226 = local read "Construction\nlevel"() -> (w2325:i32)
        n1227 = local read "Build points"() -> (w2351:dbl)
        n1228 = local read "Construction\nlevel"() -> (w2309:i32)
        n1229 = local read "Road level"() -> (w2329:i32)
        n1230 = Subtract(x=1500000 ("y"), y=w2355) -> (x-y=w2348:dbl)
        n1231 = local read "Road level"() -> (w2313:i32)
        n1232 = Max & Min(x=w2348, y=0.0) -> (max(x,y)=w2353:dbl)  [unwired: 1 out]
        n1233 = Greater Or Equal?(x=w2351, y=w2353) -> (x >= y?=w2352:bool)
        n1234 = Greater Or Equal?(x=w2325, y=1) -> (x >= y?=w2330:bool)
        n1235 = Greater Or Equal?(x=w2309, y=1) -> (x >= y?=w2303:bool)
        n1236 = And(x=w2307, y=w2303) -> (x .and. y?=w2310:bool)
        n1237 = Not Equal?(x=w2329, y=w2332) -> (x != y?=w2327:bool)
        n1238 = Not Equal?(x=w2313, y=w2314) -> (x != y?=w2311:bool)
        n1239 = And(x=w2311, y=w2310) -> (x .and. y?=w2312:bool)
        n1240 = case shown="True" w2312 {
          tunnel: w2314 -> [_ w2367]
          frame False {
          }
          frame True {
            n1241 = local write "Road level"(w2367) -> ()
            n1242 = local write "Road expansion bonus"(0.0 ("Hut dissent add mod")) -> ()
            n1243 = local write "Road land prod mod"(1.0 ("Hut dissent add mod")) -> ()
            n1244 = local write "Road trade modifier"(0.0 ("Hut dissent add mod")) -> ()
            n1245 = local write "Road upkeep"(0.0 ("Hut non-land prod mod")) -> ()
          }
        }
        n1246 = And(x=w2330, y=w2352) -> (x .and. y?=w2331:bool)
        n1247 = And(x=w2305, y=w2331) -> (x .and. y?=w2326:bool)
        n1248 = And(x=w2327, y=w2326) -> (x .and. y?=w2328:bool)
        n1249 = case shown="True" w2328 {
          tunnel: w2332 -> [_ w2387]
          tunnel: w2353 -> [_ w2380]
          tunnel: w2355 -> [_ w2379]
          frame False {
          }
          frame True {
            n1250 = local read "Build points"() -> (w2386:dbl)
            n1251 = Add(x=w2380, y=w2379) -> (x+y=w2382:dbl)
            n1252 = local write "Road level"(w2387) -> ()
            n1253 = local write "Road expansion bonus"(0.5 ("Hut dissent add mod")) -> ()
            n1254 = local write "Road land prod mod"(1.2 ("Hut dissent add mod")) -> ()
            n1255 = local write "Road invested points"(w2382) -> ()
            n1256 = local write "Road upkeep"(0.12 ("Hut non-land prod mod")) -> ()
            n1257 = Subtract(x=w2386, y=w2380) -> (x-y=w2385:dbl)
            n1258 = local write "Road trade modifier"(4.0 ("Hut non-land prod mod")) -> ()
            n1259 = local write "Build points"(w2385) -> ()
          }
        }
        n1260 = local read "Road invested points"() -> (w2354:dbl)
        n1261 = local read "Road invested points"() -> (w2362:dbl)
        n1262 = local read "Construction\nlevel"() -> (w2340:i32)
        n1263 = local read "Build points"() -> (w2345:dbl)
        n1264 = Subtract(x=500000 ("y"), y=w2354) -> (x-y=w2342:dbl)
        n1265 = local read "Construction\nlevel"() -> (w2322:i32)
        n1266 = local read "Build points"() -> (w2356:dbl)
        n1267 = local read "Road level"() -> (w2318:i32)
        n1268 = Max & Min(x=w2342, y=0.0) -> (max(x,y)=w2347:dbl)  [unwired: 1 out]
        n1269 = Subtract(x=5000000 ("y"), y=w2362) -> (x-y=w2359:dbl)
        n1270 = Greater Or Equal?(x=w2345, y=w2347) -> (x >= y?=w2346:bool)
        n1271 = Max & Min(x=w2359, y=0.0) -> (max(x,y)=w2361:dbl)  [unwired: 1 out]
        n1272 = Greater Or Equal?(x=w2322, y=1) -> (x >= y?=w2317:bool)
        n1273 = Greater Or Equal?(x=w2356, y=w2361) -> (x >= y?=w2360:bool)
        n1274 = Greater Or Equal?(x=w2340, y=1) -> (x >= y?=w2335:bool)
        n1275 = And(x=w2335, y=w2346) -> (x .and. y?=w2334:bool)
        n1276 = And(x=w2306, y=w2334) -> (x .and. y?=w2339:bool)
        n1277 = local read "Road level"() -> (w2336:i32)
        n1278 = Not Equal?(x=w2318, y=w2315) -> (x != y?=w2320:bool)
        n1279 = And(x=w2317, y=w2360) -> (x .and. y?=w2316:bool)
        n1280 = And(x=w2304, y=w2316) -> (x .and. y?=w2321:bool)
        n1281 = And(x=w2320, y=w2321) -> (x .and. y?=w2319:bool)
        n1282 = Not Equal?(x=w2336, y=w2333) -> (x != y?=w2338:bool)
        n1283 = And(x=w2338, y=w2339) -> (x .and. y?=w2337:bool)
        n1284 = case shown="True" w2319 {
          tunnel: w2315 -> [_ w2377]
          tunnel: w2361 -> [_ w2370]
          tunnel: w2362 -> [_ w2369]
          frame False {
          }
          frame True {
            n1285 = local read "Build points"() -> (w2376:dbl)
            n1286 = Add(x=w2370, y=w2369) -> (x+y=w2371:dbl)
            n1287 = local write "Road level"(w2377) -> ()
            n1288 = local write "Road expansion bonus"(1.0 ("Hut dissent add mod")) -> ()
            n1289 = local write "Road land prod mod"(1.3 ("Hut dissent add mod")) -> ()
            n1290 = local write "Road invested points"(w2371) -> ()
            n1291 = local write "Road upkeep"(0.4 ("Hut non-land prod mod")) -> ()
            n1292 = local write "Road trade modifier"(6.0 ("Hut non-land prod mod")) -> ()
            n1293 = Subtract(x=w2376, y=w2370) -> (x-y=w2375:dbl)
            n1294 = local write "Build points"(w2375) -> ()
          }
        }
        n1295 = case shown="True" w2337 {
          tunnel: w2333 -> [_ w2397]
          tunnel: w2354 -> [_ w2391]
          tunnel: w2347 -> [_ w2389]
          frame False {
          }
          frame True {
            n1296 = local read "Build points"() -> (w2396:dbl)
            n1297 = Add(x=w2389, y=w2391) -> (x+y=w2390:dbl)
            n1298 = local write "Road level"(w2397) -> ()
            n1299 = local write "Road expansion bonus"(0.2 ("Hut dissent add mod")) -> ()
            n1300 = local write "Road land prod mod"(1.1 ("Hut dissent add mod")) -> ()
            n1301 = local write "Road trade modifier"(2.0 ("Hut dissent add mod")) -> ()
            n1302 = local write "Road invested points"(w2390) -> ()
            n1303 = local write "Road upkeep"(0.04 ("Hut non-land prod mod")) -> ()
            n1304 = Subtract(x=w2396, y=w2389) -> (x-y=w2395:dbl)
            n1305 = local write "Build points"(w2395) -> ()
          }
        }
      }
      frame "Paved tar roads" {
        w2409 = 0 ("y")
        w2410 = 3 ("y")
        w2427 = 2 ("y")
        w2428 = 1 ("y")
        n1306 = local read "Road invested points"() -> (w2450:dbl)
        n1307 = local read "Construction\nlevel"() -> (w2420:i32)
        n1308 = local read "Build points"() -> (w2446:dbl)
        n1309 = local read "Construction\nlevel"() -> (w2404:i32)
        n1310 = local read "Road level"() -> (w2424:i32)
        n1311 = local read "Road level"() -> (w2408:i32)
        n1312 = Subtract(x=150000000 ("y"), y=w2450) -> (x-y=w2443:dbl)
        n1313 = Max & Min(x=w2443, y=0.0) -> (max(x,y)=w2448:dbl)  [unwired: 1 out]
        n1314 = Greater Or Equal?(x=w2446, y=w2448) -> (x >= y?=w2447:bool)
        n1315 = Greater Or Equal?(x=w2420, y=1) -> (x >= y?=w2425:bool)
        n1316 = Greater Or Equal?(x=w2404, y=1) -> (x >= y?=w2398:bool)
        n1317 = And(x=w2402, y=w2398) -> (x .and. y?=w2405:bool)
        n1318 = Not Equal?(x=w2424, y=w2427) -> (x != y?=w2422:bool)
        n1319 = Not Equal?(x=w2408, y=w2409) -> (x != y?=w2406:bool)
        n1320 = And(x=w2406, y=w2405) -> (x .and. y?=w2407:bool)
        n1321 = case shown="True" w2407 {
          tunnel: w2409 -> [_ w2462]
          frame False {
          }
          frame True {
            n1322 = local write "Road level"(w2462) -> ()
            n1323 = local write "Road expansion bonus"(0.0 ("Hut dissent add mod")) -> ()
            n1324 = local write "Road land prod mod"(1.0 ("Hut dissent add mod")) -> ()
            n1325 = local write "Road trade modifier"(0.0 ("Hut dissent add mod")) -> ()
            n1326 = local write "Road upkeep"(0.0 ("Hut non-land prod mod")) -> ()
          }
        }
        n1327 = And(x=w2425, y=w2447) -> (x .and. y?=w2426:bool)
        n1328 = And(x=w2400, y=w2426) -> (x .and. y?=w2421:bool)
        n1329 = And(x=w2422, y=w2421) -> (x .and. y?=w2423:bool)
        n1330 = case shown="True" w2423 {
          tunnel: w2427 -> [_ w2482]
          tunnel: w2448 -> [_ w2475]
          tunnel: w2450 -> [_ w2474]
          frame False {
          }
          frame True {
            n1331 = local read "Build points"() -> (w2481:dbl)
            n1332 = Add(x=w2475, y=w2474) -> (x+y=w2477:dbl)
            n1333 = local write "Road level"(w2482) -> ()
            n1334 = local write "Road expansion bonus"(0.75 ("Hut dissent add mod")) -> ()
            n1335 = local write "Road land prod mod"(1.3 ("Hut dissent add mod")) -> ()
            n1336 = local write "Road invested points"(w2477) -> ()
            n1337 = local write "Road upkeep"(0.18 ("Hut non-land prod mod")) -> ()
            n1338 = Subtract(x=w2481, y=w2475) -> (x-y=w2480:dbl)
            n1339 = local write "Road trade modifier"(4.0 ("Hut non-land prod mod")) -> ()
            n1340 = local write "Build points"(w2480) -> ()
          }
        }
        n1341 = local read "Road invested points"() -> (w2449:dbl)
        n1342 = local read "Road invested points"() -> (w2457:dbl)
        n1343 = local read "Construction\nlevel"() -> (w2435:i32)
        n1344 = local read "Build points"() -> (w2440:dbl)
        n1345 = Subtract(x=50000000 ("y"), y=w2449) -> (x-y=w2437:dbl)
        n1346 = local read "Construction\nlevel"() -> (w2417:i32)
        n1347 = local read "Build points"() -> (w2451:dbl)
        n1348 = local read "Road level"() -> (w2413:i32)
        n1349 = Max & Min(x=w2437, y=0.0) -> (max(x,y)=w2442:dbl)  [unwired: 1 out]
        n1350 = Subtract(x=500000000 ("y"), y=w2457) -> (x-y=w2454:dbl)
        n1351 = local read "Road level"() -> (w2431:i32)
        n1352 = Greater Or Equal?(x=w2440, y=w2442) -> (x >= y?=w2441:bool)
        n1353 = Max & Min(x=w2454, y=0.0) -> (max(x,y)=w2456:dbl)  [unwired: 1 out]
        n1354 = Greater Or Equal?(x=w2417, y=1) -> (x >= y?=w2412:bool)
        n1355 = Greater Or Equal?(x=w2451, y=w2456) -> (x >= y?=w2455:bool)
        n1356 = Greater Or Equal?(x=w2435, y=1) -> (x >= y?=w2430:bool)
        n1357 = And(x=w2430, y=w2441) -> (x .and. y?=w2429:bool)
        n1358 = And(x=w2401, y=w2429) -> (x .and. y?=w2434:bool)
        n1359 = Not Equal?(x=w2413, y=w2410) -> (x != y?=w2415:bool)
        n1360 = And(x=w2412, y=w2455) -> (x .and. y?=w2411:bool)
        n1361 = And(x=w2399, y=w2411) -> (x .and. y?=w2416:bool)
        n1362 = And(x=w2415, y=w2416) -> (x .and. y?=w2414:bool)
        n1363 = Not Equal?(x=w2431, y=w2428) -> (x != y?=w2433:bool)
        n1364 = And(x=w2433, y=w2434) -> (x .and. y?=w2432:bool)
        n1365 = case shown="True" w2414 {
          tunnel: w2410 -> [_ w2472]
          tunnel: w2456 -> [_ w2465]
          tunnel: w2457 -> [_ w2464]
          frame False {
          }
          frame True {
            n1366 = local read "Build points"() -> (w2471:dbl)
            n1367 = Add(x=w2465, y=w2464) -> (x+y=w2466:dbl)
            n1368 = local write "Road level"(w2472) -> ()
            n1369 = local write "Road expansion bonus"(1.5 ("Hut dissent add mod")) -> ()
            n1370 = local write "Road land prod mod"(1.45 ("Hut dissent add mod")) -> ()
            n1371 = local write "Road invested points"(w2466) -> ()
            n1372 = local write "Road upkeep"(0.6 ("Hut non-land prod mod")) -> ()
            n1373 = local write "Road trade modifier"(6.0 ("Hut non-land prod mod")) -> ()
            n1374 = Subtract(x=w2471, y=w2465) -> (x-y=w2470:dbl)
            n1375 = local write "Build points"(w2470) -> ()
          }
        }
        n1376 = case shown="True" w2432 {
          tunnel: w2428 -> [_ w2492]
          tunnel: w2449 -> [_ w2486]
          tunnel: w2442 -> [_ w2484]
          frame False {
          }
          frame True {
            n1377 = local read "Build points"() -> (w2491:dbl)
            n1378 = Add(x=w2484, y=w2486) -> (x+y=w2485:dbl)
            n1379 = local write "Road level"(w2492) -> ()
            n1380 = local write "Road expansion bonus"(0.3 ("Hut dissent add mod")) -> ()
            n1381 = local write "Road land prod mod"(1.15 ("Hut dissent add mod")) -> ()
            n1382 = local write "Road trade modifier"(2.0 ("Hut dissent add mod")) -> ()
            n1383 = local write "Road invested points"(w2485) -> ()
            n1384 = local write "Road upkeep"(0.06 ("Hut non-land prod mod")) -> ()
            n1385 = Subtract(x=w2491, y=w2484) -> (x-y=w2490:dbl)
            n1386 = local write "Build points"(w2490) -> ()
          }
        }
      }
    }
    n1387 = Subtract(x=1500000 ("y"), y=w798) -> (x-y=w805:dbl)
    n1388 = Greater Or Equal?(x=w1628, y=1) -> (x >= y?=w1626:bool)
    n1389 = And(x="Taxes level 0", y=w1626) -> (x .and. y?=w1630:bool)
    n1390 = local read "Boat level"() -> (w844:i32)
    n1391 = Max & Min(x=w186, y=0.0) -> (max(x,y)=w181:dbl)  [unwired: 1 out]
    n1392 = Greater Or Equal?(x=w1644, y=1) -> (x >= y?=w1623:bool)
    n1393 = And(x="Taxes level 2", y=w1623) -> (x .and. y?=w1646:bool)
    n1394 = Subtract(x=w2116, y=w642) -> (x-y=w1884:dbl)
    n1395 = Greater Or Equal?(x=w168, y=2) -> (x >= y?=w166:bool)
    n1396 = Greater Or Equal?(x=w183, y=w181) -> (x >= y?=w182:bool)
    n1397 = Quotient & Remainder(x=w2088, y=365.0) -> (x-y*floor(x/y)=→"Day":dbl, floor(x/y)=→"Year":dbl)
    n1398 = Not Equal?(x=w1633, y=w1634) -> (x != y?=w1631:bool)
    n1399 = And(x=w1631, y=w1630) -> (x .and. y?=w1632:bool)
    n1400 = Max & Min(x=w765, y=0.0) -> (max(x,y)=w770:dbl)  [unwired: 1 out]
    n1401 = local read "Military Modifier"() -> (w1886:dbl)
    n1402 = local read "Governance\nlevel"() -> (w1400:i32)
    n1403 = Greater Or Equal?(x=w768, y=w770) -> (x >= y?=w769:bool)
    n1404 = Greater Or Equal?(x=w209, y=3) -> (x >= y?=w204:bool)
    n1405 = Not Equal?(x=w1649, y=w1650) -> (x != y?=w1647:bool)
    n1406 = And(x=w1647, y=w1646) -> (x .and. y?=w1648:bool)
    n1407 = Greater Or Equal?(x=w742, y=1) -> (x >= y?=w747:bool)
    n1408 = Max & Min(x=w805, y=0.0) -> (max(x,y)=w800:dbl)  [unwired: 1 out]
    n1409 = Greater Or Equal?(x=w726, y=1) -> (x >= y?=w289:bool)
    n1410 = And(x="Temple\nlevel 0", y=w289) -> (x .and. y?=w727:bool)
    n1411 = Greater Or Equal?(x=w802, y=w800) -> (x >= y?=w801:bool)
    n1412 = Not Equal?(x=w205, y=w202) -> (x != y?=w207:bool)
    n1413 = Not Equal?(x=w221, y=w220) -> (x != y?=w223:bool)
    n1414 = And(x=w223, y="Market\nlevel 0") -> (x .and. y?=w222:bool)
    n1415 = local read "Gov populist\nbuildings mod"() -> (w1262:dbl)
    n1416 = case shown="True" w1369 {
      tunnel: w1365 -> [_ w3127]
      tunnel: w1343 -> [_ w3123]
      tunnel: w1341 -> [_ w3122]
      tunnel: w1262 -> [_ w3115]
      frame False {
      }
      frame True {
        n1417 = Multiply(x=w3115, y=0.1) -> (x*y=w3118:dbl)
        n1418 = Increment(x=w3118) -> (x+1=w3117:dbl)
        n1419 = local read "Build points"() -> (w3126:dbl)
        n1420 = Add(x=w3123, y=w3122) -> (x+y=w3124:dbl)
        n1421 = local write "School engineer equivalent"(0.02 ("Hut dissent add mod")) -> ()
        n1422 = local write "School level"(w3127) -> ()
        n1423 = local write "School dissent mod"(0.96 ("Hut non-land prod mod")) -> ()
        n1424 = local write "School SP/EP multiplier"(w3117) -> ()
        n1425 = local write "School invested points"(w3124) -> ()
        n1426 = local write "School upkeep"(0.003 ("Hut non-land prod mod")) -> ()
        n1427 = Subtract(x=w3126, y=w3123) -> (x-y=w3125:dbl)
        n1428 = local write "Build points"(w3125) -> ()
      }
    }
    n1429 = Greater Or Equal?(x=w828, y=1) -> (x >= y?=w823:bool)
    n1430 = And(x="Switch to Stone road", y=w359) -> (x .and. y?=w357:bool)
    n1431 = case shown="True" w1632 {
      tunnel: w1634 -> [_ w3209]
      frame False {
      }
      frame True {
        n1432 = local write "Taxation\nlevel"(w3209) -> ()
        n1433 = local write "Taxes dissent mod"(0.0 ("Taxes dissent add mod")) -> ()
      }
    }
    n1434 = case shown="True" w1648 {
      tunnel: w1650 -> [_ w3213]
      frame False {
      }
      frame True {
        n1435 = local write "Taxation\nlevel"(w3213) -> ()
        n1436 = local write "Taxes dissent mod"(8.0 ("Taxes dissent add mod")) -> ()
      }
    }
    n1437 = Not Equal?(x=w746, y=w749) -> (x != y?=w744:bool)
    n1438 = Greater Or Equal?(x=w844, y=1) -> (x >= y?=w288:bool)
    n1439 = And(x="Harbor level 0", y=w288) -> (x .and. y?=w843:bool)
    n1440 = And(x="Switch to brick house", y=w391) -> (x .and. y?=w399:bool)
    n1441 = Not Equal?(x=w730, y=w731) -> (x != y?=w728:bool)
    n1442 = And(x=w728, y=w727) -> (x .and. y?=w729:bool)
    n1443 = Compound Arithmetic op=MULTIPLY(w1886, w786, w1561, w1887, w1888, 0.064789, 2.0 ("y"), w1884) -> (w1885:dbl)
    n1444 = Add(x=w1885, y=w637) -> (x+y=w2101:dbl)
    n1445 = local read "School invested points"() -> (w1342:dbl)
    n1446 = Not Equal?(x=w824, y=w821) -> (x != y?=w826:bool)
    n1447 = Not Equal?(x=w840, y=w839) -> (x != y?=w842:bool)
    n1448 = And(x=w842, y=w843) -> (x .and. y?=w841:bool)
    n1449 = Greater Or Equal?(x=w1400, y=2) -> (x >= y?=w1399:bool)
    n1450 = case shown="True" w222 {
      tunnel: w220 -> [_ w2130]
      frame False {
      }
      frame True {
        n1451 = local write "Market domestic gold mult"(0.0 ("Hut dissent add mod")) -> ()
        n1452 = local write "Market level"(w2130) -> ()
        n1453 = local write "Market trade gold mult"(1.0 ("Hut dissent add mod")) -> ()
        n1454 = local write "Market upkeep"(0.0 ("Hut non-land prod mod")) -> ()
      }
    }
    n1455 = case shown="True" w399 {
      frame False {
      }
      frame True {
        n1456 = local write "Housing type"("Brick House" ("Housing type")) -> ()
      }
    }
    n1457 = Compound Arithmetic op=AND(w204, w182, w166) -> (w203:bool)
    n1458 = And(x="Market\nlevel 2", y=w203) -> (x .and. y?=w208:bool)
    n1459 = And(x=w207, y=w208) -> (x .and. y?=w206:bool)
    n1460 = case shown="True" w206 {
      tunnel: w202 -> [_ w2148]
      tunnel: w181 -> [_ w2140]
      tunnel: w179 -> [_ w2141]
      frame False {
      }
      frame True {
        n1461 = local read "Build points"() -> (w2147:dbl)
        n1462 = Add(x=w2140, y=w2141) -> (x+y=w2143:dbl)
        n1463 = local write "Market domestic gold mult"(4.0 ("Hut dissent add mod")) -> ()
        n1464 = local write "Market trade gold mult"(1.4 ("Hut dissent add mod")) -> ()
        n1465 = local write "Market\ninvested points"(w2143) -> ()
        n1466 = local write "Market upkeep"(0.12 ("Hut non-land prod mod")) -> ()
        n1467 = local write "Market level"(w2148) -> ()
        n1468 = Subtract(x=w2147, y=w2140) -> (x-y=w2146:dbl)
        n1469 = local write "Build points"(w2146) -> ()
      }
    }
    n1470 = case shown="True" w357 {
      frame False {
      }
      frame True {
        n1471 = local write "Road type"("Stone roads" ("Housing type")) -> ()
      }
    }
    n1472 = case shown="True" w729 {
      tunnel: w731 -> [_ w2871]
      frame False {
      }
      frame True {
        n1473 = local write "Temple level"(w2871) -> ()
        n1474 = local write "Temple SP/EP multiplier"(1.0 ("Hut dissent add mod")) -> ()
        n1475 = local write "Temple dissent mod"(1.0 ("Hut dissent add mod")) -> ()
        n1476 = local write "Temple upkeep"(0.0 ("Hut non-land prod mod")) -> ()
      }
    }
    n1477 = And(x=w747, y=w769) -> (x .and. y?=w748:bool)
    n1478 = And(x="Temple\nlevel 2", y=w748) -> (x .and. y?=w743:bool)
    n1479 = And(x=w744, y=w743) -> (x .and. y?=w745:bool)
    n1480 = case shown="True" w745 {
      tunnel: w749 -> [_ w2889]
      tunnel: w770 -> [_ w2881]
      tunnel: w772 -> [_ w2884]
      frame False {
      }
      frame True {
        n1481 = local read "Gold dbl"() -> (w2882:dbl)
        n1482 = Add(x=w2881, y=w2884) -> (x+y=w2886:dbl)
        n1483 = local write "Temple level"(w2889) -> ()
        n1484 = local write "Temple SP/EP multiplier"(1.0 ("Hut dissent add mod")) -> ()
        n1485 = local write "Temple dissent mod"(0.9 ("Hut dissent add mod")) -> ()
        n1486 = local write "Temple\ninvested points"(w2886) -> ()
        n1487 = local write "Temple upkeep"(0.003 ("Hut non-land prod mod")) -> ()
        n1488 = Subtract(x=w2882, y=w2881) -> (x-y=w2883:dbl)
        n1489 = local write "Gold dbl"(w2883) -> ()
      }
    }
    n1490 = local read "School invested points"() -> (w1334:dbl)
    n1491 = case shown="True" w841 {
      tunnel: w839 -> [_ w2902]
      frame False {
      }
      frame True {
        n1492 = local write "Harbor level"(w2902) -> ()
        n1493 = local write "Harbor expansion bonus"(0.0 ("Hut dissent add mod")) -> ()
        n1494 = local write "Harbor military mod"(1.0 ("Hut dissent add mod")) -> ()
        n1495 = local write "Harbor upkeep"(0.0 ("Hut non-land prod mod")) -> ()
      }
    }
    n1496 = And(x=w823, y=w801) -> (x .and. y?=w822:bool)
    n1497 = And(x="Harbor level 2", y=w822) -> (x .and. y?=w827:bool)
    n1498 = And(x=w826, y=w827) -> (x .and. y?=w825:bool)
    n1499 = case shown="True" w825 {
      tunnel: w821 -> [_ w2920]
      tunnel: w800 -> [_ w2913]
      tunnel: w798 -> [_ w2912]
      frame False {
      }
      frame True {
        n1500 = local read "Build points"() -> (w2919:dbl)
        n1501 = Add(x=w2913, y=w2912) -> (x+y=w2915:dbl)
        n1502 = local write "Harbor level"(w2920) -> ()
        n1503 = local write "Harbor expansion bonus"(0.25 ("Hut dissent add mod")) -> ()
        n1504 = local write "Harbor military mod"(1.2 ("Hut dissent add mod")) -> ()
        n1505 = local write "Harbor\ninvested points"(w2915) -> ()
        n1506 = local write "Harbor upkeep"(0.12 ("Hut non-land prod mod")) -> ()
        n1507 = Subtract(x=w2919, y=w2913) -> (x-y=w2918:dbl)
        n1508 = local write "Build points"(w2918) -> ()
      }
    }
    n1509 = local read "Permanent\nland"() -> (w287:dbl)
    n1510 = local read "People"() -> (w2112:i64)
    n1511 = local read "Construction\nlevel"() -> (w1356:i32)
    n1512 = local read "Build points"() -> (w1351:dbl)
    n1513 = local read "Market\ninvested points"() -> (w180:dbl)
    n1514 = local read "Temple\ninvested points"() -> (w771:dbl)
    n1515 = local read "Harbor expansion bonus"() -> (w785:dbl)
    n1516 = Subtract(x=200000 ("y"), y=w1342) -> (x-y=w1354:dbl)
    n1517 = local read "Road expansion bonus"() -> (w1734:dbl)
    n1518 = Divide(x=w2112, y=w287) -> (x/y=w2111:dbl)
    n1519 = Divide(x=w637, y=w287) -> (x/y=w2110:dbl)
    n1520 = local read "Construction\nlevel"() -> (w1376:i32)
    n1521 = local read "School level"() -> (w1361:i32)
    n1522 = local read "Build points"() -> (w1340:dbl)
    n1523 = local read "Temple\ninvested points"() -> (w779:dbl)
    n1524 = local read "Market\ninvested points"() -> (w172:dbl)
    n1525 = local read "School level"() -> (w1381:i32)
    n1526 = local read "Harbor\ninvested points"() -> (w799:dbl)
    n1527 = Subtract(x=2000000 ("y"), y=w1334) -> (x-y=w1337:dbl)
    n1528 = Square(x=w2111) -> (x^2=w2109:dbl)
    n1529 = Square(x=w2110) -> (x^2=w2108:dbl)
    n1530 = local read "Economics\nlevel"() -> (w1657:i32)
    n1531 = Max & Min(x=w1354, y=0.0) -> (max(x,y)=w1349:dbl)  [unwired: 1 out]
    n1532 = Greater Or Equal?(x=w1351, y=w1349) -> (x >= y?=w1350:bool)
    n1533 = local read "Harbor\ninvested points"() -> (w791:dbl)
    n1534 = local read "Land conv mult"() -> (w640:dbl)
    n1535 = local read "Economics\nlevel"() -> (w194:i32)
    n1536 = local read "Economics\nlevel"() -> (w1641:i32)
    n1537 = local read "Construction\nlevel"() -> (w757:i32)
    n1538 = local read "Build points"() -> (w189:dbl)
    n1539 = Max & Min(x=w1337, y=0.0) -> (max(x,y)=w1335:dbl)  [unwired: 1 out]
    n1540 = Greater Or Equal?(x=w1356, y=2) -> (x >= y?=w1362:bool)
    n1541 = Compound Arithmetic op=AND(w1362, w1350, w1399) -> (w1363:bool)
    n1542 = And(x="School\nlevel 1", y=w1363) -> (x .and. y?=w1358:bool)
    n1543 = local read "Taxation\nlevel"() -> (w1652:dbl)
    n1544 = local read "Taxation\nlevel"() -> (w1636:dbl)
    n1545 = Greater Or Equal?(x=w1340, y=w1335) -> (x >= y?=w1336:bool)
    n1546 = Greater Or Equal?(x=w1376, y=3) -> (x >= y?=w1382:bool)
    n1547 = Subtract(x=5000000 ("y"), y=w180) -> (x-y=w192:dbl)
    n1548 = local read "Gold dbl"() -> (w762:dbl)
    n1549 = Not Equal?(x=w1361, y=w1364) -> (x != y?=w1359:bool)
    n1550 = And(x=w1359, y=w1358) -> (x .and. y?=w1360:bool)
    n1551 = local read "Economics\nlevel"() -> (w212:i32)
    n1552 = local read "Construction\nlevel"() -> (w162:i32)
    n1553 = Multiply(x=w2109, y=w2108) -> (x*y=w2099:dbl)
    n1554 = Subtract(x=500 ("y"), y=w771) -> (x-y=w759:dbl)
    n1555 = Not Equal?(x=w1381, y=w1384) -> (x != y?=w1379:bool)
    n1556 = local read "Build points"() -> (w178:dbl)
    n1557 = local read "Build points"() -> (w808:dbl)
    n1558 = local read "Construction\nlevel"() -> (w739:i32)
    n1559 = local read "Boat level"() -> (w813:i32)
    n1560 = local read "Temple level"() -> (w735:i32)
    n1561 = Subtract(x=50000000 ("y"), y=w172) -> (x-y=w175:dbl)
    n1562 = Subtract(x=500000 ("y"), y=w799) -> (x-y=w811:dbl)
    n1563 = local read "Gold dbl"() -> (w773:dbl)
    n1564 = local read "Temple level"() -> (w753:i32)
    n1565 = Max & Min(x=w192, y=0.0) -> (max(x,y)=w187:dbl)  [unwired: 1 out]
    n1566 = Subtract(x=500000 ("y"), y=w779) -> (x-y=w776:dbl)
    n1567 = Y-th Root of X(1:w287, 2:4.0 ("y")) -> (0:w2098:dbl)
    n1568 = Multiply(x=w2099, y=w2098) -> (x*y=w2034:dbl)
    n1569 = local read "Governance\nlevel"() -> (w1404:i32)
    n1570 = Greater Or Equal?(x=w189, y=w187) -> (x >= y?=w188:bool)
    n1571 = local read "Build points"() -> (w797:dbl)
    n1572 = local read "Harbor level"() -> (w835:i32)
    n1573 = Max & Min(x=w759, y=0.0) -> (max(x,y)=w764:dbl)  [unwired: 1 out]
    n1574 = local read "Construction\nlevel"() -> (w164:i32)
    n1575 = local read "Harbor level"() -> (w817:i32)
    n1576 = Greater Or Equal?(x=w762, y=w764) -> (x >= y?=w763:bool)
    n1577 = local read "Boat level"() -> (w831:i32)
    n1578 = case shown="True" "Switch to Multilayer stone road" {
      frame False {
      }
      frame True {
        n1579 = local write "Road type"("Multilayer stone roads" ("Housing type")) -> ()
      }
    }
    n1580 = Subtract(x=5000000 ("y"), y=w791) -> (x-y=w794:dbl)
    n1581 = Greater Or Equal?(x=w1657, y=1) -> (x >= y?=w1625:bool)
    n1582 = Greater Or Equal?(x=w1641, y=1) -> (x >= y?=w1624:bool)
    n1583 = And(x="Taxes level 1", y=w1625) -> (x .and. y?=w1655:bool)
    n1584 = And(x="Taxes level 3", y=w1624) -> (x .and. y?=w1639:bool)
    n1585 = case shown="True" "Switch to hut" {
      frame False {
      }
      frame True {
        n1586 = local write "Housing type"("Hut" ("Housing type")) -> ()
      }
    }
    n1587 = Max & Min(x=w175, y=0.0) -> (max(x,y)=w173:dbl)  [unwired: 1 out]
    n1588 = Increment(x=w1734) -> (x+1=w1733:dbl)
    n1589 = Max & Min(x=w811, y=0.0) -> (max(x,y)=w806:dbl)  [unwired: 1 out]
    n1590 = Increment(x=w785) -> (x+1=w784:dbl)
    n1591 = Compound Arithmetic op=MULTIPLY(w784, w1733, w640, w2034, 1.5e-05 ("y")) -> (w638:dbl)
    "Land conversion rate" <- w638
    n1592 = Add(x=w1822, y=w638) -> (x+y=w2105:dbl)
    n1593 = local write "Permanent\nland"(w2105) -> ()
    n1594 = Greater Or Equal?(x=w178, y=w173) -> (x >= y?=w174:bool)
    n1595 = Greater Or Equal?(x=w808, y=w806) -> (x >= y?=w807:bool)
    n1596 = Not Equal?(x=w1652, y=w1651) -> (x != y?=w1654:bool)
    n1597 = And(x=w1654, y=w1655) -> (x .and. y?=w1653:bool)
    n1598 = Not Equal?(x=w1636, y=w1635) -> (x != y?=w1638:bool)
    n1599 = And(x=w1638, y=w1639) -> (x .and. y?=w1637:bool)
    n1600 = Max & Min(x=w776, y=0.0) -> (max(x,y)=w778:dbl)  [unwired: 1 out]
    n1601 = local read "Market level"() -> (w198:i32)
    n1602 = local read "Market level"() -> (w216:i32)
    n1603 = Greater Or Equal?(x=w773, y=w778) -> (x >= y?=w777:bool)
    n1604 = case shown="True" w1637 {
      tunnel: w1635 -> [_ w3211]
      frame False {
      }
      frame True {
        n1605 = local write "Taxation\nlevel"(w3211) -> ()
        n1606 = local write "Taxes dissent mod"(15.0 ("Taxes dissent add mod")) -> ()
      }
    }
    n1607 = Greater Or Equal?(x=w162, y=2) -> (x >= y?=w160:bool)
    n1608 = case shown="True" w1360 {
      tunnel: w1364 -> [_ w3140]
      tunnel: w1342 -> [_ w3137]
      tunnel: w1349 -> [_ w3135]
      tunnel: w1262 -> [_ w3128]
      frame False {
      }
      frame True {
        n1609 = Multiply(x=w3128, y=0.05) -> (x*y=w3130:dbl)
        n1610 = Increment(x=w3130) -> (x+1=w3131:dbl)
        n1611 = local read "Build points"() -> (w3139:dbl)
        n1612 = Add(x=w3135, y=w3137) -> (x+y=w3136:dbl)
        n1613 = local write "School level"(w3140) -> ()
        n1614 = local write "School engineer equivalent"(0.01 ("Hut dissent add mod")) -> ()
        n1615 = local write "School SP/EP multiplier"(w3131) -> ()
        n1616 = local write "School invested points"(w3136) -> ()
        n1617 = local write "School dissent mod"(0.98 ("Hut non-land prod mod")) -> ()
        n1618 = Subtract(x=w3139, y=w3135) -> (x-y=w3138:dbl)
        n1619 = local write "School upkeep"(0.001 ("Hut non-land prod mod")) -> ()
        n1620 = local write "Build points"(w3138) -> ()
      }
    }
    n1621 = Greater Or Equal?(x=w212, y=3) -> (x >= y?=w217:bool)
    n1622 = Greater Or Equal?(x=w164, y=2) -> (x >= y?=w163:bool)
    n1623 = Greater Or Equal?(x=w194, y=3) -> (x >= y?=w199:bool)
    n1624 = Compound Arithmetic op=AND(w199, w188, w163) -> (w200:bool)
    n1625 = And(x="Market\nlevel 1", y=w200) -> (x .and. y?=w195:bool)
    n1626 = Greater Or Equal?(x=w739, y=1) -> (x >= y?=w734:bool)
    n1627 = Subtract(x=w2101, y=w638) -> (x-y=w2006:dbl)
    n1628 = Max & Min(x=w794, y=0.0) -> (max(x,y)=w792:dbl)  [unwired: 1 out]
    n1629 = Greater Or Equal?(x=w757, y=1) -> (x >= y?=w752:bool)
    n1630 = And(x=w752, y=w763) -> (x .and. y?=w751:bool)
    n1631 = And(x="Temple\nlevel 1", y=w751) -> (x .and. y?=w756:bool)
    n1632 = Not Equal?(x=w216, y=w219) -> (x != y?=w214:bool)
    n1633 = Compound Arithmetic op=AND(w217, w174, w160) -> (w218:bool)
    n1634 = And(x="Market\nlevel 3", y=w218) -> (x .and. y?=w213:bool)
    n1635 = And(x=w214, y=w213) -> (x .and. y?=w215:bool)
    n1636 = Greater Or Equal?(x=w797, y=w792) -> (x >= y?=w793:bool)
    n1637 = case shown="True" w1653 {
      tunnel: w1651 -> [_ w3215]
      frame False {
      }
      frame True {
        n1638 = local write "Taxation\nlevel"(w3215) -> ()
        n1639 = local write "Taxes dissent mod"(3.0 ("Taxes dissent add mod")) -> ()
      }
    }
    n1640 = Not Equal?(x=w198, y=w201) -> (x != y?=w196:bool)
    n1641 = And(x=w196, y=w195) -> (x .and. y?=w197:bool)
    n1642 = Not Equal?(x=w735, y=w732) -> (x != y?=w737:bool)
    n1643 = Greater Or Equal?(x=w831, y=1) -> (x >= y?=w836:bool)
    n1644 = Not Equal?(x=w753, y=w750) -> (x != y?=w755:bool)
    n1645 = And(x=w755, y=w756) -> (x .and. y?=w754:bool)
    n1646 = Greater Or Equal?(x=w1404, y=2) -> (x >= y?=w1406:bool)
    n1647 = Compound Arithmetic op=AND(w1382, w1336, w1406) -> (w1383:bool)
    n1648 = And(x="School\nlevel 3", y=w1383) -> (x .and. y?=w1378:bool)
    n1649 = And(x=w1379, y=w1378) -> (x .and. y?=w1380:bool)
    n1650 = case shown="True" w1380 {
      tunnel: w1384 -> [_ w3114]
      tunnel: w1335 -> [_ w3110]
      tunnel: w1334 -> [_ w3109]
      tunnel: w1262 -> [_ w3102]
      frame False {
      }
      frame True {
        n1651 = Multiply(x=w3102, y=0.15) -> (x*y=w3105:dbl)
        n1652 = local read "Build points"() -> (w3113:dbl)
        n1653 = Add(x=w3110, y=w3109) -> (x+y=w3111:dbl)
        n1654 = Increment(x=w3105) -> (x+1=w3104:dbl)
        n1655 = local write "School level"(w3114) -> ()
        n1656 = local write "School engineer equivalent"(0.03 ("Hut dissent add mod")) -> ()
        n1657 = local write "School invested points"(w3111) -> ()
        n1658 = local write "School SP/EP multiplier"(w3104) -> ()
        n1659 = local write "School dissent mod"(0.94 ("Hut non-land prod mod")) -> ()
        n1660 = Subtract(x=w3113, y=w3110) -> (x-y=w3112:dbl)
        n1661 = local write "School upkeep"(0.01 ("Hut non-land prod mod")) -> ()
        n1662 = local write "Build points"(w3112) -> ()
      }
    }
    n1663 = Greater Or Equal?(x=w813, y=1) -> (x >= y?=w818:bool)
    n1664 = And(x=w818, y=w807) -> (x .and. y?=w819:bool)
    n1665 = And(x="Harbor level 1", y=w819) -> (x .and. y?=w814:bool)
    n1666 = case shown="True" w215 {
      tunnel: w219 -> [_ w2139]
      tunnel: w173 -> [_ w2131]
      tunnel: w172 -> [_ w2132]
      frame False {
      }
      frame True {
        n1667 = local read "Build points"() -> (w2138:dbl)
        n1668 = Add(x=w2131, y=w2132) -> (x+y=w2133:dbl)
        n1669 = local write "Market domestic gold mult"(6.0 ("Hut dissent add mod")) -> ()
        n1670 = local write "Market trade gold mult"(1.6 ("Hut dissent add mod")) -> ()
        n1671 = local write "Market level"(w2139) -> ()
        n1672 = local write "Market\ninvested points"(w2133) -> ()
        n1673 = local write "Market upkeep"(0.4 ("Hut non-land prod mod")) -> ()
        n1674 = Subtract(x=w2138, y=w2131) -> (x-y=w2137:dbl)
        n1675 = local write "Build points"(w2137) -> ()
      }
    }
    n1676 = Not Equal?(x=w835, y=w838) -> (x != y?=w833:bool)
    n1677 = And(x=w836, y=w793) -> (x .and. y?=w837:bool)
    n1678 = And(x="Harbor level 3", y=w837) -> (x .and. y?=w832:bool)
    n1679 = And(x=w833, y=w832) -> (x .and. y?=w834:bool)
    n1680 = And(x=w734, y=w777) -> (x .and. y?=w733:bool)
    n1681 = And(x="Temple\nlevel 3", y=w733) -> (x .and. y?=w738:bool)
    n1682 = And(x=w737, y=w738) -> (x .and. y?=w736:bool)
    n1683 = Not Equal?(x=w817, y=w820) -> (x != y?=w815:bool)
    n1684 = And(x=w815, y=w814) -> (x .and. y?=w816:bool)
    n1685 = case shown="True" w736 {
      tunnel: w732 -> [_ w2880]
      tunnel: w778 -> [_ w2872]
      tunnel: w779 -> [_ w2875]
      frame False {
      }
      frame True {
        n1686 = Add(x=w2872, y=w2875) -> (x+y=w2876:dbl)
        n1687 = local read "Gold dbl"() -> (w2874:dbl)
        n1688 = local write "Temple level"(w2880) -> ()
        n1689 = local write "Temple SP/EP multiplier"(1.0 ("Hut dissent add mod")) -> ()
        n1690 = local write "Temple dissent mod"(0.85 ("Hut dissent add mod")) -> ()
        n1691 = local write "Temple\ninvested points"(w2876) -> ()
        n1692 = local write "Temple upkeep"(0.01 ("Hut non-land prod mod")) -> ()
        n1693 = Subtract(x=w2874, y=w2872) -> (x-y=w2873:dbl)
        n1694 = local write "Gold dbl"(w2873) -> ()
      }
    }
    n1695 = case shown="True" w197 {
      tunnel: w201 -> [_ w2157]
      tunnel: w180 -> [_ w2151]
      tunnel: w187 -> [_ w2149]
      frame False {
      }
      frame True {
        n1696 = local read "Build points"() -> (w2156:dbl)
        n1697 = Add(x=w2149, y=w2151) -> (x+y=w2150:dbl)
        n1698 = local write "Market domestic gold mult"(2.0 ("Hut dissent add mod")) -> ()
        n1699 = local write "Market\ninvested points"(w2150) -> ()
        n1700 = local write "Market trade gold mult"(1.2 ("Hut dissent add mod")) -> ()
        n1701 = local write "Market upkeep"(0.04 ("Hut non-land prod mod")) -> ()
        n1702 = Subtract(x=w2156, y=w2149) -> (x-y=w2155:dbl)
        n1703 = local write "Market level"(w2157) -> ()
        n1704 = local write "Build points"(w2155) -> ()
      }
    }
    n1705 = case shown="True" w754 {
      tunnel: w750 -> [_ w2898]
      tunnel: w771 -> [_ w2894]
      tunnel: w764 -> [_ w2891]
      frame False {
      }
      frame True {
        n1706 = Add(x=w2891, y=w2894) -> (x+y=w2893:dbl)
        n1707 = local read "Gold dbl"() -> (w2892:dbl)
        n1708 = local write "Temple level"(w2898) -> ()
        n1709 = local write "Temple SP/EP multiplier"(1.0 ("Hut dissent add mod")) -> ()
        n1710 = local write "Temple dissent mod"(0.95 ("Hut dissent add mod")) -> ()
        n1711 = local write "Temple\ninvested points"(w2893) -> ()
        n1712 = local write "Temple upkeep"(0.001 ("Hut non-land prod mod")) -> ()
        n1713 = Subtract(x=w2892, y=w2891) -> (x-y=w2890:dbl)
        n1714 = local write "Gold dbl"(w2890) -> ()
      }
    }
    n1715 = Multiply(x=w2006, y=0.01) -> (x*y=w2005:dbl)
    n1716 = Multiply(x=0.99, y=w2006) -> (x*y=w2104:dbl)
    n1717 = case shown="True" w834 {
      tunnel: w838 -> [_ w2911]
      tunnel: w792 -> [_ w2904]
      tunnel: w791 -> [_ w2903]
      frame False {
      }
      frame True {
        n1718 = local read "Build points"() -> (w2910:dbl)
        n1719 = Add(x=w2904, y=w2903) -> (x+y=w2905:dbl)
        n1720 = local write "Harbor level"(w2911) -> ()
        n1721 = local write "Harbor expansion bonus"(0.5 ("Hut dissent add mod")) -> ()
        n1722 = local write "Harbor military mod"(1.3 ("Hut dissent add mod")) -> ()
        n1723 = local write "Harbor\ninvested points"(w2905) -> ()
        n1724 = local write "Harbor upkeep"(0.4 ("Hut non-land prod mod")) -> ()
        n1725 = Subtract(x=w2910, y=w2904) -> (x-y=w2909:dbl)
        n1726 = local write "Build points"(w2909) -> ()
      }
    }
    n1727 = local read "Concrete house\nunlocked"() -> (w365:bool)
    n1728 = case shown="True" w816 {
      tunnel: w820 -> [_ w2929]
      tunnel: w799 -> [_ w2923]
      tunnel: w806 -> [_ w2921]
      frame False {
      }
      frame True {
        n1729 = local read "Build points"() -> (w2928:dbl)
        n1730 = Add(x=w2921, y=w2923) -> (x+y=w2922:dbl)
        n1731 = local write "Harbor level"(w2929) -> ()
        n1732 = local write "Harbor expansion bonus"(0.1 ("Hut dissent add mod")) -> ()
        n1733 = local write "Harbor military mod"(1.1 ("Hut dissent add mod")) -> ()
        n1734 = local write "Harbor\ninvested points"(w2922) -> ()
        n1735 = local write "Harbor upkeep"(0.04 ("Hut non-land prod mod")) -> ()
        n1736 = Subtract(x=w2928, y=w2921) -> (x-y=w2927:dbl)
        n1737 = local write "Build points"(w2927) -> ()
      }
    }
    n1738 = local read "Concrete house\nunlocked"() -> (w362:bool)
    n1739 = Add(x=w2005, y=w638) -> (x+y=w2004:dbl)
    n1740 = Subtract(x=w1885, y=w2004) -> (x-y=w2003:dbl)
    n1741 = local write "Temp land change/s"(w2003) -> ()
    n1742 = local write "Conquered\nland"(w2104) -> ()
    n1743 = And(x=w365, y="Switch to concrete housing") -> (x .and. y?=w364:bool)
    n1744 = And(x=w362, y="Switch to Paved tar roads") -> (x .and. y?=w363:bool)
    n1745 = case shown="True" w364 {
      frame False {
      }
      frame True {
        n1746 = local write "Housing type"("Concrete Housing" ("Housing type")) -> ()
      }
    }
    n1747 = case shown="True" w363 {
      frame False {
      }
      frame True {
        n1748 = local write "Road type"("Paved tar roads" ("Housing type")) -> ()
      }
    }
    n1749 = local read "Construction\nlevel"() -> (w381:i32)
    n1750 = local read "Construction\nlevel"() -> (w386:i32)
    n1751 = local read "Concrete house\nunlocked"() -> (w375:bool)
    n1752 = local read "Brick house\nunlocked"() -> (w394:bool)
    n1753 = Greater Or Equal?(x=w381, y=5) -> (x >= y?=w382:bool)
    n1754 = Greater Or Equal?(x=w386, y=3) -> (x >= y?=w385:bool)
    n1755 = local read "EP"() -> (w374:dbl)
    n1756 = local read "EP"() -> (w395:dbl)
    n1757 = local read "Construction\nlevel"() -> (w347:i32)
    n1758 = local read "Construction\nlevel"() -> (w342:i32)
    n1759 = Greater Or Equal?(x=w374, y=w373) -> (x >= y?=w377:bool)
    n1760 = Greater Or Equal?(x=w395, y=w396) -> (x >= y?=w392:bool)
    n1761 = Subtract(x=w374, y=w373) -> (x-y=w372:dbl)
    n1762 = local read "Mutilayer\nStone roads\nunlocked"() -> (w336:bool)
    n1763 = Subtract(x=w395, y=w396) -> (x-y=w397:dbl)
    n1764 = Equal?(x=w375, y=FALSE) -> (x = y?=w380:bool)
    n1765 = Compound Arithmetic op=AND(w380, "Unlock concrete house", w382, w377) -> (w376:bool)
    n1766 = Equal?(x=w394, y=FALSE) -> (x = y?=w387:bool)
    n1767 = Compound Arithmetic op=AND(w387, "Unlock brick house", w385, w392) -> (w393:bool)
    n1768 = local read "Paved tar roads\nunlocked"() -> (w353:bool)
    n1769 = case shown="True" w376 {
      tunnel: w372 -> [_ w2495]
      frame False {
      }
      frame True {
        n1770 = local write "EP"(w2495) -> ()
        n1771 = local write "Concrete house\nunlocked"(TRUE ("Brick house\nunlocked")) -> ()
      }
    }
    n1772 = case shown="True" w393 {
      tunnel: w397 -> [_ w2498]
      frame False {
      }
      frame True {
        n1773 = local write "EP"(w2498) -> ()
        n1774 = local write "Brick house\nunlocked"(TRUE ("Brick house\nunlocked")) -> ()
      }
    }
    n1775 = Greater Or Equal?(x=w347, y=5) -> (x >= y?=w346:bool)
    n1776 = Greater Or Equal?(x=w342, y=3) -> (x >= y?=w343:bool)
    n1777 = local read "EP"() -> (w354:dbl)
    n1778 = local read "EP"() -> (w335:dbl)
    n1779 = Greater Or Equal?(x=w354, y=w355) -> (x >= y?=w351:bool)
    n1780 = Greater Or Equal?(x=w335, y=w334) -> (x >= y?=w338:bool)
    n1781 = Subtract(x=w354, y=w355) -> (x-y=w356:dbl)
    n1782 = Subtract(x=w335, y=w334) -> (x-y=w333:dbl)
    n1783 = Equal?(x=w353, y=FALSE) -> (x = y?=w348:bool)
    n1784 = Compound Arithmetic op=AND(w348, "Unlock paved tar roads", w346, w351) -> (w352:bool)
    n1785 = Equal?(x=w336, y=FALSE) -> (x = y?=w341:bool)
    n1786 = Compound Arithmetic op=AND(w341, "Unlock multilayer stone roads", w343, w338) -> (w337:bool)
    n1787 = case shown="True" w352 {
      tunnel: w356 -> [_ w2202]
      frame False {
      }
      frame True {
        n1788 = local write "EP"(w2202) -> ()
        n1789 = local write "Paved tar roads\nunlocked"(TRUE ("Brick house\nunlocked")) -> ()
      }
    }
    n1790 = case shown="True" w337 {
      tunnel: w333 -> [_ w2204]
      frame False {
      }
      frame True {
        n1791 = local write "EP"(w2204) -> ()
        n1792 = local write "Mutilayer\nStone roads\nunlocked"(TRUE ("Brick house\nunlocked")) -> ()
      }
    }
    n1793 = local read "University\ninvested points"() -> (w1253:dbl)
    n1794 = local read "Economics\nlevel"() -> (w1492:i32)
    n1795 = local read "Taxation\nlevel"() -> (w1497:dbl)
    n1796 = local read "Military\nScience level"() -> (w471:i32)
    n1797 = local read "Military\nScience level"() -> (w474:i32)
    n1798 = local read "Physics level"() -> (w525:i32)
    n1799 = local read "Physics level"() -> (w487:i32)
    n1800 = local read "Military\nScience level"() -> (w566:i32)
    n1801 = local read "Construction\nlevel"() -> (w1221:i32)
    n1802 = local read "Physics level"() -> (w458:i32)
    n1803 = local read "Physics level"() -> (w406:i32)
    n1804 = local read "Construction\nlevel"() -> (w1201:i32)
    n1805 = local read "University level"() -> (w1206:i32)
    n1806 = local read "Build points"() -> (w1249:dbl)
    n1807 = local read "University level"() -> (w1226:i32)
    n1808 = local read "Governance\nlevel"() -> (w1198:i32)
    n1809 = local read "Physics level"() -> (w432:i32)
    n1810 = local read "Physics level"() -> (w429:i32)
    n1811 = local read "Military\nScience level"() -> (w1879:i32)
    n1812 = local read "Physics level"() -> (w455:i32)
    n1813 = Subtract(x=600000 ("y"), y=w1253) -> (x-y=w1246:dbl)
    n1814 = local read "Governance\nlevel"() -> (w1192:i32)
    n1815 = local read "Vehicle\nlevel"() -> (w416:i32)
    n1816 = local read "Electronics\nlevel"() -> (w477:i32)
    n1817 = local read "Electronics\nlevel"() -> (w468:i32)
    n1818 = local read "Electronics\nlevel"() -> (w551:i32)
    n1819 = Greater Or Equal?(x=w1492, y=1) -> (x >= y?=w1499:bool)
    n1820 = And(x="Taxes level 4", y=w1499) -> (x .and. y?=w1494:bool)
    n1821 = local read "Vehicle\nlevel"() -> (w442:i32)
    n1822 = local read "Vehicle\nlevel"() -> (w419:i32)
    n1823 = local read "Vehicle\nlevel"() -> (w445:i32)
    n1824 = Not Equal?(x=w1497, y=w1498) -> (x != y?=w1495:bool)
    n1825 = And(x=w1495, y=w1494) -> (x .and. y?=w1496:bool)
    n1826 = local read "Biology\nlevel"() -> (w1803:i32)
    n1827 = local read "Physics level"() -> (w1845:i32)
    n1828 = Greater Or Equal?(x=w487, y=5.0) -> (x >= y?=w488:bool)
    n1829 = Max & Min(x=w1246, y=0.0) -> (max(x,y)=w1251:dbl)  [unwired: 1 out]
    n1830 = local read "Physics level"() -> (w573:i32)
    n1831 = Greater Or Equal?(x=w458, y=5.0) -> (x >= y?=w457:bool)
    n1832 = Greater Or Equal?(x=w1249, y=w1251) -> (x >= y?=w1250:bool)
    n1833 = Greater Or Equal?(x=w525, y=5.0) -> (x >= y?=w524:bool)
    n1834 = Greater Or Equal?(x=w474, y=3.0) -> (x >= y?=w473:bool)
    n1835 = Greater Or Equal?(x=w1201, y=2) -> (x >= y?=w1207:bool)
    n1836 = case shown="True" w1496 {
      tunnel: w1498 -> [_ w3166]
      frame False {
      }
      frame True {
        n1837 = local write "Taxation\nlevel"(w3166) -> ()
        n1838 = local write "Taxes dissent mod"(25.0 ("Taxes dissent add mod")) -> ()
      }
    }
    n1839 = Greater Or Equal?(x=w406, y=5.0) -> (x >= y?=w405:bool)
    n1840 = Greater Or Equal?(x=w1221, y=3) -> (x >= y?=w1227:bool)
    n1841 = Greater Or Equal?(x=w1198, y=2) -> (x >= y?=w1197:bool)
    n1842 = Greater Or Equal?(x=w471, y=3.0) -> (x >= y?=w472:bool)
    n1843 = Greater Or Equal?(x=w566, y=3.0) -> (x >= y?=w567:bool)
    n1844 = Not Equal?(x=w1206, y=w1209) -> (x != y?=w1204:bool)
    n1845 = Greater Or Equal?(x=w1192, y=2) -> (x >= y?=w1191:bool)
    n1846 = Greater Or Equal?(x=w432, y=5.0) -> (x >= y?=w431:bool)
    n1847 = Not Equal?(x=w1226, y=w1229) -> (x != y?=w1224:bool)
    n1848 = Greater Or Equal?(x=w429, y=5.0) -> (x >= y?=w430:bool)
    n1849 = local read "EP"() -> (w414:dbl)
    n1850 = Greater Or Equal?(x=w455, y=5.0) -> (x >= y?=w456:bool)
    n1851 = local read "EP"() -> (w479:dbl)
    n1852 = local read "EP"() -> (w440:dbl)
    n1853 = local read "Governance\nlevel"() -> (w2032:i32)
    n1854 = local read "EP"() -> (w421:dbl)
    n1855 = local read "# of level 10 sciences"() -> (w1701:i32)
    n1856 = local read "EP"() -> (w466:dbl)
    n1857 = local read "EP"() -> (w447:dbl)
    n1858 = local read "# of level 5 sciences"() -> (w1706:i32)
    n1859 = local read "# of level 6 sciences"() -> (w1705:i32)
    n1860 = local read "# of level 7 sciences"() -> (w1704:i32)
    n1861 = local read "# of level 8 sciences"() -> (w1703:i32)
    n1862 = local read "# of level 9 sciences"() -> (w1702:i32)
    n1863 = local read "EP"() -> (w549:dbl)
    n1864 = local read "# of level 1 sciences"() -> (w1710:i32)
    n1865 = local read "# of level 2 sciences"() -> (w1709:i32)
    n1866 = local read "# of level 3 sciences"() -> (w1708:i32)
    n1867 = local read "# of level 4 sciences"() -> (w1707:i32)
    n1868 = local read "Governance\nlevel"() -> (w2019:i32)
    n1869 = Greater Or Equal?(x=w414, y=w413) -> (x >= y?=w409:bool)
    n1870 = Compound Arithmetic op=AND(w1207, w1197) -> (w1208:bool)
    n1871 = And(x="University\nlevel 0", y=w1208) -> (x .and. y?=w1203:bool)
    n1872 = And(x=w1204, y=w1203) -> (x .and. y?=w1205:bool)
    n1873 = case shown="True" w1205 {
      tunnel: w1209 -> [_ w3038]
      frame False {
      }
      frame True {
        n1874 = local write "University scientist equivalent"(0.0 ("Hut dissent add mod")) -> ()
        n1875 = local write "University level"(w3038) -> ()
        n1876 = local write "University SP multiplier"(1.0 ("Hut non-land prod mod")) -> ()
        n1877 = local write "University dissent mod"(1.0 ("Hut non-land prod mod")) -> ()
        n1878 = local write "University upkeep"(0.0 ("Hut non-land prod mod")) -> ()
      }
    }
    n1879 = Subtract(x=w414, y=w413) -> (x-y=w412:dbl)
    n1880 = Equal?(x=w416, y=0.0) -> (x = y?=w411:bool)
    n1881 = Compound Arithmetic op=AND(w1227, w1250, w1191) -> (w1228:bool)
    n1882 = And(x="University\nlevel 2", y=w1228) -> (x .and. y?=w1223:bool)
    n1883 = And(x=w1224, y=w1223) -> (x .and. y?=w1225:bool)
    n1884 = Compound Arithmetic op=AND(w411, "Rocket", w405, w409) -> (w408:bool)
    n1885 = Increment(x=w416) -> (x+1=w415:i32)
    n1886 = Greater Or Equal?(x=w1879, y=2.0) -> (x >= y?=w1883:bool)
    n1887 = Greater Or Equal?(x=w479, y=w480) -> (x >= y?=w484:bool)
    n1888 = Subtract(x=w479, y=w480) -> (x-y=w481:dbl)
    n1889 = Equal?(x=w477, y=1.0) -> (x = y?=w482:bool)
    n1890 = Compound Arithmetic op=AND(w482, "Radio", w473, w488, w484) -> (w485:bool)
    n1891 = Greater Or Equal?(x=w440, y=w439) -> (x >= y?=w435:bool)
    n1892 = Increment(x=w477) -> (x+1=w478:i32)
    n1893 = Greater Or Equal?(x=w421, y=w422) -> (x >= y?=w426:bool)
    n1894 = Subtract(x=w440, y=w439) -> (x-y=w438:dbl)
    n1895 = local read "Government"() -> (w2027:string)
    n1896 = Greater Or Equal?(x=w466, y=w465) -> (x >= y?=w461:bool)
    n1897 = Equal?(x=w442, y=0.0) -> (x = y?=w437:bool)
    n1898 = Subtract(x=w421, y=w422) -> (x-y=w423:dbl)
    n1899 = Greater Or Equal?(x=w447, y=w448) -> (x >= y?=w452:bool)
    n1900 = Compound Arithmetic op=AND(w437, "Internal combustion engine (cars)", w431, w435) -> (w434:bool)
    n1901 = Equal?(x=w419, y=0.0) -> (x = y?=w424:bool)
    n1902 = Greater Or Equal?(x=w549, y=w548) -> (x >= y?=w544:bool)
    n1903 = Subtract(x=w466, y=w465) -> (x-y=w464:dbl)
    n1904 = Increment(x=w442) -> (x+1=w441:i32)
    n1905 = Compound Arithmetic op=AND(w424, "Aircraft", w430, w426) -> (w427:bool)
    n1906 = local read "Government"() -> (w2014:string)
    n1907 = Subtract(x=w447, y=w448) -> (x-y=w449:dbl)
    n1908 = Equal?(x=w468, y=2.0) -> (x = y?=w463:bool)
    n1909 = Increment(x=w419) -> (x+1=w420:i32)
    n1910 = Subtract(x=w549, y=w548) -> (x-y=w547:dbl)
    n1911 = Compound Arithmetic op=AND(w463, "Computer", w472, w457, w461) -> (w460:bool)
    n1912 = Equal?(x=w445, y=0.0) -> (x = y?=w450:bool)
    n1913 = Compound Arithmetic op=AND(w450, "Steam Powered Train", w456, w452) -> (w453:bool)
    n1914 = And(x="Bow 1", y=w1883) -> (x .and. y?=w1881:bool)
    n1915 = Equal?(x=w551, y=0.0) -> (x = y?=w546:bool)
    n1916 = Increment(x=w468) -> (x+1=w467:i32)
    n1917 = local read "Farming level"() -> (w1810:i32)
    n1918 = Compound Arithmetic op=AND(w546, "Light bulb", w567, w524, w544) -> (w543:bool)
    n1919 = Increment(x=w445) -> (x+1=w446:i32)
    n1920 = Increment(x=w551) -> (x+1=w550:i32)
    n1921 = Greater Or Equal?(x=w1803, y=3.0) -> (x >= y?=w1802:bool)
    n1922 = Greater Or Equal?(x=w1845, y=3.0) -> (x >= y?=w1846:bool)
    n1923 = local read "Governance\nlevel"() -> (w1194:i32)
    n1924 = local read "Bow level"() -> (w1896:i32)
    n1925 = local read "Boat level"() -> (w1838:i32)
    n1926 = local read "Governance\nlevel"() -> (w2054:i32)
    n1927 = Greater Or Equal?(x=w573, y=3.0) -> (x >= y?=w572:bool)
    n1928 = local read "Boat level"() -> (w580:i32)
    n1929 = local read "Government"() -> (w2041:string)
    n1930 = local read "Spear level"() -> (w2075:i32)
    n1931 = local read "SP"() -> (w2026:dbl)
    n1932 = local read "SP"() -> (w2013:dbl)
    n1933 = case shown="True" w408 {
      tunnel: w415 -> [_ w2786]
      tunnel: w412 -> [_ w2785]
      frame False {
      }
      frame True {
        n1934 = local write "EP"(w2785) -> ()
        n1935 = local write "Vehicle\nlevel"(w2786) -> ()
      }
    }
    n1936 = local read "Net level"() -> (w2068:i32)
    n1937 = case shown="True" w485 {
      tunnel: w478 -> [_ w2796]
      tunnel: w481 -> [_ w2795]
      frame False {
      }
      frame True {
        n1938 = local write "EP"(w2795) -> ()
        n1939 = local write "Electronics\nlevel"(w2796) -> ()
      }
    }
    n1940 = local read "EP"() -> (w1898:dbl)
    n1941 = local read "EP"() -> (w1808:dbl)
    n1942 = local read "EP"() -> (w1840:dbl)
    n1943 = local read "SP"() -> (w2040:dbl)
    n1944 = case shown="True" w434 {
      tunnel: w441 -> [_ w2790]
      tunnel: w438 -> [_ w2789]
      frame False {
      }
      frame True {
        n1945 = local write "EP"(w2789) -> ()
        n1946 = local write "Vehicle\nlevel"(w2790) -> ()
      }
    }
    n1947 = local read "EP"() -> (w578:dbl)
    n1948 = case shown="True" w427 {
      tunnel: w420 -> [_ w2788]
      tunnel: w423 -> [_ w2787]
      frame False {
      }
      frame True {
        n1949 = local write "EP"(w2787) -> ()
        n1950 = local write "Vehicle\nlevel"(w2788) -> ()
      }
    }
    n1951 = local read "EP"() -> (w2082:dbl)
    n1952 = local read "Gov elitist\nbuildings mod"() -> (w1261:dbl)
    n1953 = case shown="True" w1225 {
      tunnel: w1229 -> [_ w3064]
      tunnel: w1251 -> [_ w3060]
      tunnel: w1253 -> [_ w3059]
      tunnel: w1261 -> [_ w3052]
      frame False {
      }
      frame True {
        n1954 = Multiply(x=w3052, y=0.3) -> (x*y=w3055:dbl)
        n1955 = Increment(x=w3055) -> (x+1=w3054:dbl)
        n1956 = local read "Build points"() -> (w3063:dbl)
        n1957 = Add(x=w3060, y=w3059) -> (x+y=w3061:dbl)
        n1958 = local write "University scientist equivalent"(0.04 ("Hut dissent add mod")) -> ()
        n1959 = local write "University level"(w3064) -> ()
        n1960 = local write "University dissent mod"(0.96 ("Hut non-land prod mod")) -> ()
        n1961 = local write "University\ninvested points"(w3061) -> ()
        n1962 = local write "University upkeep"(0.015 ("Hut non-land prod mod")) -> ()
        n1963 = local write "University SP multiplier"(w3054) -> ()
        n1964 = Subtract(x=w3063, y=w3060) -> (x-y=w3062:dbl)
        n1965 = local write "Build points"(w3062) -> ()
      }
    }
    n1966 = case shown="True" w460 {
      tunnel: w467 -> [_ w2794]
      tunnel: w464 -> [_ w2793]
      frame False {
      }
      frame True {
        n1967 = local write "EP"(w2793) -> ()
        n1968 = local write "Electronics\nlevel"(w2794) -> ()
      }
    }
    n1969 = case shown="True" w453 {
      tunnel: w446 -> [_ w2792]
      tunnel: w449 -> [_ w2791]
      frame False {
      }
      frame True {
        n1970 = local write "EP"(w2791) -> ()
        n1971 = local write "Vehicle\nlevel"(w2792) -> ()
      }
    }
    n1972 = local read "University\ninvested points"() -> (w1252:dbl)
    n1973 = local read "EP"() -> (w2059:dbl)
    n1974 = case shown="True" w543 {
      tunnel: w550 -> [_ w2804]
      tunnel: w547 -> [_ w2803]
      frame False {
      }
      frame True {
        n1975 = local write "EP"(w2803) -> ()
        n1976 = local write "Electronics\nlevel"(w2804) -> ()
      }
    }
    n1977 = Greater Or Equal?(x=w2032, y=1) -> (x >= y?=w2023:bool)
    n1978 = Greater Or Equal?(x=w2026, y=0) -> (x >= y?=w2024:bool)
    n1979 = Greater Or Equal?(x=w2019, y=1) -> (x >= y?=w2010:bool)
    n1980 = Greater Or Equal?(x=w2013, y=0) -> (x >= y?=w2011:bool)
    n1981 = Not Equal?(x=w2027, y=w2021) -> (x != y?=w2029:bool)
    n1982 = Greater Or Equal?(x=w1898, y=w1899) -> (x >= y?=w1891:bool)
    n1983 = Greater Or Equal?(x=w1808, y=w1807) -> (x >= y?=w1801:bool)
    n1984 = Greater Or Equal?(x=w1840, y=w1841) -> (x >= y?=w1847:bool)
    n1985 = Greater Or Equal?(x=w2082, y=10000) -> (x >= y?=w2084:bool)
    n1986 = Subtract(x=w1898, y=w1899) -> (x-y=w1900:dbl)
    n1987 = Subtract(x=w1808, y=w1807) -> (x-y=w1806:dbl)
    n1988 = And(x="Net 1", y=w2084) -> (x .and. y?=w2071:bool)
    n1989 = Subtract(x=w1840, y=w1841) -> (x-y=w1842:dbl)
    n1990 = Not Equal?(x=w2014, y=w2008) -> (x != y?=w2016:bool)
    n1991 = Equal?(x=w1896, y=0.0) -> (x = y?=w1894:bool)
    n1992 = And(x=w1894, y=w1881) -> (x .and. y?=w1895:bool)
    n1993 = And(x=w1895, y=w1891) -> (x .and. y?=w1892:bool)
    n1994 = Equal?(x=w1810, y=0.0) -> (x = y?=w1805:bool)
    n1995 = Equal?(x=w1838, y=0.0) -> (x = y?=w1843:bool)
    n1996 = Compound Arithmetic op=AND(w1805, "Farming 1", w1802, w1801) -> (w1800:bool)
    n1997 = Greater Or Equal?(x=w1194, y=2) -> (x >= y?=w1195:bool)
    n1998 = Compound Arithmetic op=AND(w1843, "Raft", w1846, w1847) -> (w1848:bool)
    n1999 = Greater Or Equal?(x=w578, y=w577) -> (x >= y?=w571:bool)
    n2000 = Increment(x=w1896) -> (x+1=w1897:i32)
    n2001 = Increment(x=w1810) -> (x+1=w1809:i32)
    n2002 = Greater Or Equal?(x=w2054, y=1) -> (x >= y?=w2037:bool)
    n2003 = Increment(x=w1838) -> (x+1=w1839:i32)
    n2004 = Subtract(x=w578, y=w577) -> (x-y=w576:dbl)
    n2005 = Greater Or Equal?(x=w2040, y=0) -> (x >= y?=w2038:bool)
    n2006 = Equal?(x=w580, y=2.0) -> (x = y?=w575:bool)
    n2007 = local read "University\ninvested points"() -> (w1260:dbl)
    n2008 = Greater Or Equal?(x=w2059, y=w2058) -> (x >= y?=w2081:bool)
    n2009 = Compound Arithmetic op=AND(w575, "Caravel", w572, w571) -> (w570:bool)
    n2010 = Increment(x=w580) -> (x+1=w579:i32)
    n2011 = Subtract(x=w2059, y=w2058) -> (x-y=w2057:dbl)
    n2012 = Equal?(x=w2075, y=0.0) -> (x = y?=w2078:bool)
    n2013 = And(x=w2078, y="Sharpened stick") -> (x .and. y?=w2076:bool)
    n2014 = And(x=w2076, y=w2081) -> (x .and. y?=w2080:bool)
    n2015 = Build Array(0, w1710, w1709, w1708, w1707, w1706, w1705, w1704, w1703, w1702, w1701) -> (w1700:T2)
    n2016 = local read "Economics\nlevel"() -> (w661:i32)
    n2017 = Increment(x=w2075) -> (x+1=w2074:i32)
    n2018 = Equal?(x=w2068, y=0.0) -> (x = y?=w2070:bool)
    n2019 = And(x=w2070, y=w2071) -> (x .and. y?=w2069:bool)
    n2020 = case shown="True" w1848 {
      tunnel: w1839 -> [_ w3448]
      tunnel: w1842 -> [_ w3447]
      frame False {
      }
      frame True {
        n2021 = local read "Trading level no mod"() -> (w3446:i32)
        n2022 = local read "hunting b"() -> (w3443:dbl)
        n2023 = local write "EP"(w3447) -> ()
        n2024 = local write "Boat level"(w3448) -> ()
        n2025 = Increment(x=w3446) -> (x+1=w3445:i32)
        n2026 = local write "Trading level no mod"(w3445) -> ()
        n2027 = Add(x=0.25, y=w3443) -> (x+y=w3444:dbl)
        n2028 = local write "hunting b"(w3444) -> ()
      }
    }
    n2029 = Not Equal?(x=w2041, y=w2035) -> (x != y?=w2051:bool)
    n2030 = case shown="True" w570 {
      tunnel: w579 -> [_ w2822]
      tunnel: w576 -> [_ w2821]
      frame False {
      }
      frame True {
        n2031 = local read "Trading level no mod"() -> (w2820:i32)
        n2032 = local write "EP"(w2821) -> ()
        n2033 = local read "warrior b"() -> (w2818:dbl)
        n2034 = local write "Boat level"(w2822) -> ()
        n2035 = Increment(x=w2820) -> (x+1=w2816:i32)
        n2036 = Add(x=0.25, y=w2818) -> (x+y=w2819:dbl)
        n2037 = Increment(x=w2816) -> (x+1=w2815:i32)
        n2038 = local write "Trading level no mod"(w2815) -> ()
        n2039 = local write "warrior b"(w2819) -> ()
      }
    }
    n2040 = And(x=w2023, y=w2024) -> (x .and. y?=w2022:bool)
    n2041 = And(x="Theocracy", y=w2022) -> (x .and. y?=w2030:bool)
    n2042 = And(x=w2029, y=w2030) -> (x .and. y?=w2028:bool)
    n2043 = case shown="True" w2028 {
      tunnel: w2021 -> [_ w3523]
      frame False {
      }
      frame True {
        n2044 = local read "SP"() -> (w3520:dbl)
        n2045 = local write "Government"(w3523) -> ()
        n2046 = Subtract(x=w3520, y=0) -> (x-y=w3522:dbl)
        n2047 = local write "SP"(w3522) -> ()
      }
    }
    n2048 = local read "Taxation\nlevel"() -> (w656:dbl)
    n2049 = And(x=w2010, y=w2011) -> (x .and. y?=w2009:bool)
    n2050 = And(x="Warrior\nSociety", y=w2009) -> (x .and. y?=w2017:bool)
    n2051 = And(x=w2016, y=w2017) -> (x .and. y?=w2015:bool)
    n2052 = case shown="True" w1892 {
      tunnel: w1897 -> [_ w3470]
      tunnel: w1900 -> [_ w3469]
      frame False {
      }
      frame True {
        n2053 = local read "Military Modifier"() -> (w3468:dbl)
        n2054 = local write "EP"(w3469) -> ()
        n2055 = local read "hunting b"() -> (w3473:dbl)
        n2056 = local write "Bow level"(w3470) -> ()
        n2057 = Add(x=0.125, y=w3473) -> (x+y=w3471:dbl)
        n2058 = local write "hunting b"(w3471) -> ()
        n2059 = Multiply(x=1.125, y=w3468) -> (x*y=w3467:dbl)
        n2060 = local write "Military Modifier"(w3467) -> ()
      }
    }
    n2061 = case shown="True" w1800 {
      tunnel: w1809 -> [_ w3427]
      tunnel: w1806 -> [_ w3426]
      frame False {
      }
      frame True {
        n2062 = local read "hunting b"() -> (w3424:dbl)
        n2063 = local read "hunting a"() -> (w3421:dbl)
        n2064 = local write "EP"(w3426) -> ()
        n2065 = local write "Farming level"(w3427) -> ()
        n2066 = Add(x=1.0, y=w3421) -> (x+y=w3420:dbl)
        n2067 = Add(x=0.5, y=w3424) -> (x+y=w3425:dbl)
        n2068 = local write "hunting b"(w3425) -> ()
        n2069 = local write "hunting a"(w3420) -> ()
      }
    }
    n2070 = case shown="True" w2015 {
      tunnel: w2008 -> [_ w3519]
      frame False {
      }
      frame True {
        n2071 = local read "SP"() -> (w3518:dbl)
        n2072 = local write "Government"(w3519) -> ()
        n2073 = Subtract(x=w3518, y=0) -> (x-y=w3516:dbl)
        n2074 = local write "SP"(w3516) -> ()
      }
    }
    n2075 = Increment(x=w2068) -> (x+1=w2067:i32)
    n2076 = case shown="True" w2080 {
      tunnel: w2074 -> [_ w4148]
      tunnel: w2057 -> [_ w4147]
      frame False {
      }
      frame True {
        w4152 = 0.25
        n2077 = local write "EP"(w4147) -> ()
        n2078 = local read "warrior a"() -> (w4151:dbl)
        n2079 = local read "hunting a"() -> (w4153:dbl)
        n2080 = local write "Spear level"(w4148) -> ()
        n2081 = Add(x=w4152, y=w4151) -> (x+y=w4150:dbl)
        n2082 = Add(x=w4152, y=w4153) -> (x+y=w4149:dbl)
        n2083 = local write "warrior a"(w4150) -> ()
        n2084 = local write "hunting a"(w4149) -> ()
      }
    }
    n2085 = case shown="True" w2069 {
      tunnel: w2082 -> [_ w4142]
      tunnel: w2067 -> [_ w4140]
      frame False {
      }
      frame True {
        n2086 = local read "hunting b"() -> (w4145:dbl)
        n2087 = local write "Net level"(w4140) -> ()
        n2088 = Subtract(x=w4142, y=10000.0) -> (x-y=w4141:dbl)
        n2089 = local write "EP"(w4141) -> ()
        n2090 = Add(x=w4145, y=0.25) -> (x+y=w4144:dbl)
        n2091 = local write "hunting b"(w4144) -> ()
      }
    }
    n2092 = And(x=w2037, y=w2038) -> (x .and. y?=w2036:bool)
    n2093 = And(x="Democracy", y=w2036) -> (x .and. y?=w2052:bool)
    n2094 = And(x=w2051, y=w2052) -> (x .and. y?=w2050:bool)
    n2095 = call-poly <vilib>:"Matrix To Array.vi"("Real Matrix"=w1700) -> ("Real 2D Array"=w1699:dbl[][])
    n2096 = case shown="True" w2050 {
      tunnel: w2035 -> [_ w3534]
      frame False {
      }
      frame True {
        n2097 = local write "Government"(w3534) -> ()
        n2098 = local read "SP"() -> (w3533:dbl)
        n2099 = Subtract(x=w3533, y=0) -> (x-y=w3531:dbl)
        n2100 = local write "SP"(w3531) -> ()
      }
    }
    n2101 = local read "Construction\nlevel"() -> (w1238:i32)
    n2102 = local read "Build points"() -> (w1243:dbl)
    n2103 = Index Array(array=w1699, index (row)=0) -> (element=w849:dbl[])  [unwired: 1 in]
    n2104 = local read "Military\nScience level"() -> (w2056:i32)
    n2105 = Greater Or Equal?(x=w661, y=1) -> (x >= y?=w654:bool)
    n2106 = And(x="Taxes level 5", y=w654) -> (x .and. y?=w659:bool)
    n2107 = Subtract(x=200000 ("y"), y=w1252) -> (x-y=w1240:dbl)
    n2108 = Not Equal?(x=w656, y=w655) -> (x != y?=w658:bool)
    n2109 = And(x=w658, y=w659) -> (x .and. y?=w657:bool)
    n2110 = local read "Construction\nlevel"() -> (w1218:i32)
    n2111 = local read "University level"() -> (w1213:i32)
    n2112 = local read "University level"() -> (w1233:i32)
    n2113 = local read "Build points"() -> (w1254:dbl)
    n2114 = local read "Governance\nlevel"() -> (w2042:i32)
    n2115 = Subtract(x=2000000 ("y"), y=w1260) -> (x-y=w1257:dbl)
    n2116 = Max & Min(x=w1240, y=0.0) -> (max(x,y)=w1245:dbl)  [unwired: 1 out]
    n2117 = case shown="True" w657 {
      tunnel: w655 -> [_ w2836]
      frame False {
      }
      frame True {
        n2118 = local write "Taxation\nlevel"(w2836) -> ()
        n2119 = local write "Taxes dissent mod"(40.0 ("Taxes dissent add mod")) -> ()
      }
    }
    n2120 = Greater Or Equal?(x=w1243, y=w1245) -> (x >= y?=w1244:bool)
    n2121 = local read "Military\nScience level"() -> (w1932:i32)
    n2122 = Max & Min(x=w1257, y=0.0) -> (max(x,y)=w1259:dbl)  [unwired: 1 out]
    n2123 = Greater Or Equal?(x=w1254, y=w1259) -> (x >= y?=w1258:bool)
    n2124 = Greater Or Equal?(x=w1218, y=3) -> (x >= y?=w1212:bool)
    n2125 = Greater Or Equal?(x=w1238, y=2) -> (x >= y?=w1232:bool)
    n2126 = Compound Arithmetic op=AND(w1232, w1244, w1195) -> (w1231:bool)
    n2127 = And(x="University\nlevel 1", y=w1231) -> (x .and. y?=w1236:bool)
    n2128 = local read "Governance\nlevel"() -> (w1978:i32)
    n2129 = local read "Governance\nlevel"() -> (w1976:i32)
    n2130 = local read "Physics level"() -> (w518:i32)
    n2131 = local read "Physics level"() -> (w491:i32)
    n2132 = local read "Military\nScience level"() -> (w516:i32)
    n2133 = local read "Military\nScience level"() -> (w493:i32)
    n2134 = Not Equal?(x=w1213, y=w1210) -> (x != y?=w1215:bool)
    n2135 = local read "Physics level"() -> (w529:i32)
    n2136 = local read "Physics level"() -> (w523:i32)
    n2137 = local read "Military\nScience level"() -> (w531:i32)
    n2138 = Not Equal?(x=w1233, y=w1230) -> (x != y?=w1235:bool)
    n2139 = And(x=w1235, y=w1236) -> (x .and. y?=w1234:bool)
    n2140 = local read "Military\nScience level"() -> (w563:i32)
    n2141 = local read "SP"() -> (w2061:dbl)
    n2142 = Increment(x=w2056) -> (x+1=w1697:i32)
    n2143 = Index Array(array=w849, index=w1697) -> (element=w1695:dbl)
    n2144 = Power Of 10(x=w2056) -> (10^x=w2065:dbl)
    n2145 = local read "SP"() -> (w2044:dbl)
    n2146 = local read "Governance\nlevel"() -> (w1991:i32)
    n2147 = Power Of 10(x=w2042) -> (10^x=w2048:dbl)
    n2148 = Power Of 2(x=w1695) -> (2^x=w1696:dbl)
    n2149 = local read "Government"() -> (w1996:string)
    n2150 = local read "Governance\nlevel"() -> (w1190:i32)
    n2151 = local read "Government"() -> (w1983:string)
    n2152 = local read "Government"() -> (w1971:string)
    n2153 = local read "Net level"() -> (w1951:i32)
    n2154 = Compound Arithmetic op=MULTIPLY(w2065, 1000, w1696) -> (w2060:dbl)
    n2155 = local read "Military\nScience level"() -> (w1727:i32)
    n2156 = case shown="True" w1234 {
      tunnel: w1230 -> [_ w3077]
      tunnel: w1252 -> [_ w3074]
      tunnel: w1245 -> [_ w3072]
      tunnel: w1261 -> [_ w3065]
      frame False {
      }
      frame True {
        n2157 = Multiply(x=w3065, y=0.15) -> (x*y=w3067:dbl)
        n2158 = Increment(x=w3067) -> (x+1=w3068:dbl)
        n2159 = local read "Build points"() -> (w3076:dbl)
        n2160 = Add(x=w3072, y=w3074) -> (x+y=w3073:dbl)
        n2161 = local write "University level"(w3077) -> ()
        n2162 = local write "University scientist equivalent"(0.02 ("Hut dissent add mod")) -> ()
        n2163 = local write "University\ninvested points"(w3073) -> ()
        n2164 = local write "University SP multiplier"(w3068) -> ()
        n2165 = local write "University dissent mod"(0.98 ("Hut non-land prod mod")) -> ()
        n2166 = local write "University upkeep"(0.005 ("Hut non-land prod mod")) -> ()
        n2167 = Subtract(x=w3076, y=w3072) -> (x-y=w3075:dbl)
        n2168 = local write "Build points"(w3075) -> ()
      }
    }
    n2169 = local read "Military\nScience level"() -> (w596:i32)
    n2170 = local read "EP"() -> (w1945:dbl)
    n2171 = local read "Military\nScience level"() -> (w1878:i32)
    n2172 = Greater?(x=w2061, y=w2060) -> (0:w2063:bool)
    n2173 = And(x="Military science", y=w2063) -> (x .and. y?=w2062:bool)
    n2174 = local read "SP"() -> (w1997:dbl)
    n2175 = local read "SP"() -> (w1984:dbl)
    n2176 = local read "SP"() -> (w1970:dbl)
    n2177 = local read "Physics level"() -> (w1853:i32)
    n2178 = local read "Physics level"() -> (w1826:i32)
    n2179 = Greater Or Equal?(x=w1945, y=100000) -> (x >= y?=w1943:bool)
    n2180 = local read "Physics level"() -> (w592:i32)
    n2181 = local read "Biology\nlevel"() -> (w1785:i32)
    n2182 = And(x="Net 2", y=w1943) -> (x .and. y?=w1948:bool)
    n2183 = Greater Or Equal?(x=w1932, y=1.0) -> (x >= y?=w1931:bool)
    n2184 = case shown="True" w2062 {
      selector: w2062 -> [w4130 w4133]
      tunnel: w2061 -> [_ w4136]
      tunnel: w2060 -> [_ w4135]
      tunnel: w1697 -> [_ w4132]
      tunnel: [w4130 w4133] -> w1712
      tunnel: [0 w4132] -> w1723
      frame False {
      }
      frame True {
        n2185 = local read "warrior c"() -> (w4139:dbl)
        n2186 = Subtract(x=w4136, y=w4135) -> (x-y=w4134:dbl)
        n2187 = local write "SP"(w4134) -> ()
        n2188 = Subtract(x=w4139, y=0.03) -> (x-y=w4138:dbl)
        n2189 = local write "Military\nScience level"(w4132) -> ()
        n2190 = local write "warrior c"(w4138) -> ()
      }
    }
    n2191 = Increment(x=w2042) -> (x+1=w1692:i32)
    n2192 = Index Array(array=w849, index=w1692) -> (element=w1694:dbl)
    n2193 = Power Of 2(x=w1694) -> (2^x=w1693:dbl)
    n2194 = Compound Arithmetic op=MULTIPLY(w2048, 1000, w1693) -> (w2043:dbl)
    n2195 = Greater?(x=w2044, y=w2043) -> (0:w2046:bool)
    n2196 = And(x="Governance", y=w2046) -> (x .and. y?=w2045:bool)
    n2197 = case shown="True" w2045 {
      selector: w2045 -> [w3524 w3527]
      tunnel: w2044 -> [_ w3530]
      tunnel: w2043 -> [_ w3529]
      tunnel: w1692 -> [_ w3526]
      tunnel: [w3524 w3527] -> w1713
      tunnel: [0 w3526] -> w1722
      frame False {
      }
      frame True {
        n2198 = Subtract(x=w3530, y=w3529) -> (x-y=w3528:dbl)
        n2199 = local write "SP"(w3528) -> ()
        n2200 = local write "Governance\nlevel"(w3526) -> ()
      }
    }
    n2201 = Greater Or Equal?(x=w1991, y=2) -> (x >= y?=w2000:bool)
    n2202 = Greater Or Equal?(x=w1997, y=100000) -> (x >= y?=w1999:bool)
    n2203 = local read "Optics\nlevel"() -> (w513:i32)
    n2204 = Greater Or Equal?(x=w1978, y=2) -> (x >= y?=w1987:bool)
    n2205 = Equal?(x=w1951, y=1.0) -> (x = y?=w1949:bool)
    n2206 = And(x=w1949, y=w1948) -> (x .and. y?=w1950:bool)
    n2207 = local read "Optics\nlevel"() -> (w496:i32)
    n2208 = Greater Or Equal?(x=w1976, y=2) -> (x >= y?=w1967:bool)
    n2209 = Greater Or Equal?(x=w1984, y=100000) -> (x >= y?=w1986:bool)
    n2210 = Greater Or Equal?(x=w1970, y=100000) -> (x >= y?=w1968:bool)
    n2211 = And(x="Stone\nspear", y=w1931) -> (x .and. y?=w1929:bool)
    n2212 = local read "Optics\nlevel"() -> (w534:i32)
    n2213 = Greater Or Equal?(x=w1190, y=2) -> (x >= y?=w1188:bool)
    n2214 = Compound Arithmetic op=AND(w1212, w1258, w1188) -> (w1211:bool)
    n2215 = And(x="University\nlevel 3", y=w1211) -> (x .and. y?=w1216:bool)
    n2216 = And(x=w1215, y=w1216) -> (x .and. y?=w1214:bool)
    n2217 = case shown="True" w1214 {
      tunnel: w1210 -> [_ w3051]
      tunnel: w1259 -> [_ w3047]
      tunnel: w1260 -> [_ w3046]
      tunnel: w1261 -> [_ w3039]
      frame False {
      }
      frame True {
        n2218 = Multiply(x=w3039, y=0.45) -> (x*y=w3042:dbl)
        n2219 = local read "Build points"() -> (w3050:dbl)
        n2220 = Add(x=w3047, y=w3046) -> (x+y=w3048:dbl)
        n2221 = Increment(x=w3042) -> (x+1=w3041:dbl)
        n2222 = local write "University level"(w3051) -> ()
        n2223 = local write "University scientist equivalent"(0.06 ("Hut dissent add mod")) -> ()
        n2224 = local write "University\ninvested points"(w3048) -> ()
        n2225 = local write "University dissent mod"(0.94 ("Hut non-land prod mod")) -> ()
        n2226 = local write "University SP multiplier"(w3041) -> ()
        n2227 = local write "University upkeep"(0.05 ("Hut non-land prod mod")) -> ()
        n2228 = Subtract(x=w3050, y=w3047) -> (x-y=w3049:dbl)
        n2229 = local write "Build points"(w3049) -> ()
      }
    }
    n2230 = local read "Economics\nlevel"() -> (w646:i32)
    n2231 = Not Equal?(x=w1996, y=w2002) -> (x != y?=w1994:bool)
    n2232 = local read "Optics\nlevel"() -> (w554:i32)
    n2233 = Not Equal?(x=w1983, y=w1989) -> (x != y?=w1981:bool)
    n2234 = Not Equal?(x=w1971, y=w1965) -> (x != y?=w1973:bool)
    n2235 = local read "Spear level"() -> (w1935:i32)
    n2236 = Greater Or Equal?(x=w518, y=6.0) -> (x >= y?=w520:bool)
    n2237 = Increment(x=w1951) -> (x+1=w1952:i32)
    n2238 = Greater Or Equal?(x=w491, y=6.0) -> (x >= y?=w489:bool)
    n2239 = local read "Taxation\nlevel"() -> (w651:dbl)
    n2240 = case shown="True" w1950 {
      tunnel: w1945 -> [_ w3499]
      tunnel: w1952 -> [_ w3497]
      frame False {
      }
      frame True {
        n2241 = local read "hunting b"() -> (w3502:dbl)
        n2242 = local write "Net level"(w3497) -> ()
        n2243 = Subtract(x=w3499, y=100000.0) -> (x-y=w3498:dbl)
        n2244 = local write "EP"(w3498) -> ()
        n2245 = Add(x=w3502, y=0.125) -> (x+y=w3501:dbl)
        n2246 = local write "hunting b"(w3501) -> ()
      }
    }
    n2247 = Greater Or Equal?(x=w529, y=4.0) -> (x >= y?=w527:bool)
    n2248 = Greater Or Equal?(x=w523, y=6.0) -> (x >= y?=w521:bool)
    n2249 = And(x=w2000, y=w1999) -> (x .and. y?=w2001:bool)
    n2250 = And(x="Democracy 2", y=w2001) -> (x .and. y?=w1993:bool)
    n2251 = And(x=w1994, y=w1993) -> (x .and. y?=w1995:bool)
    n2252 = local read "EP"() -> (w1940:dbl)
    n2253 = case shown="True" w1995 {
      tunnel: w2002 -> [_ w3515]
      frame False {
      }
      frame True {
        n2254 = local write "Government"(w3515) -> ()
        n2255 = local read "SP"() -> (w3512:dbl)
        n2256 = Subtract(x=w3512, y=100000) -> (x-y=w3514:dbl)
        n2257 = local write "SP"(w3514) -> ()
      }
    }
    n2258 = And(x=w1987, y=w1986) -> (x .and. y?=w1988:bool)
    n2259 = And(x="Theocracy 2", y=w1988) -> (x .and. y?=w1980:bool)
    n2260 = And(x=w1981, y=w1980) -> (x .and. y?=w1982:bool)
    n2261 = And(x=w1967, y=w1968) -> (x .and. y?=w1966:bool)
    n2262 = And(x="Warrior\nSociety 2", y=w1966) -> (x .and. y?=w1974:bool)
    n2263 = And(x=w1973, y=w1974) -> (x .and. y?=w1972:bool)
    n2264 = Greater Or Equal?(x=w516, y=4.0) -> (x >= y?=w517:bool)
    n2265 = case shown="True" w1982 {
      tunnel: w1989 -> [_ w3511]
      frame False {
      }
      frame True {
        n2266 = local write "Government"(w3511) -> ()
        n2267 = local read "SP"() -> (w3510:dbl)
        n2268 = Subtract(x=w3510, y=100000) -> (x-y=w3508:dbl)
        n2269 = local write "SP"(w3508) -> ()
      }
    }
    n2270 = Greater Or Equal?(x=w493, y=4.0) -> (x >= y?=w492:bool)
    n2271 = case shown="True" w1972 {
      tunnel: w1965 -> [_ w3507]
      frame False {
      }
      frame True {
        n2272 = local write "Government"(w3507) -> ()
        n2273 = local read "SP"() -> (w3504:dbl)
        n2274 = Subtract(x=w3504, y=100000) -> (x-y=w3506:dbl)
        n2275 = local write "SP"(w3506) -> ()
      }
    }
    n2276 = Greater Or Equal?(x=w531, y=4.0) -> (x >= y?=w530:bool)
    n2277 = Greater Or Equal?(x=w563, y=3.0) -> (x >= y?=w568:bool)
    n2278 = Greater Or Equal?(x=w1940, y=3000) -> (x >= y?=w1942:bool)
    n2279 = And(x=w1929, y=w1942) -> (x .and. y?=w1938:bool)
    n2280 = local read "EP"() -> (w511:dbl)
    n2281 = local read "EP"() -> (w498:dbl)
    n2282 = local read "EP"() -> (w556:dbl)
    n2283 = local read "EP"() -> (w536:dbl)
    n2284 = Equal?(x=w1935, y=1.0) -> (x = y?=w1937:bool)
    n2285 = And(x=w1937, y=w1938) -> (x .and. y?=w1936:bool)
    n2286 = Greater Or Equal?(x=w1853, y=3.0) -> (x >= y?=w1851:bool)
    n2287 = local read "Bow level"() -> (w1876:i32)
    n2288 = local read "Farming level"() -> (w1778:i32)
    n2289 = Greater Or Equal?(x=w1826, y=4.0) -> (x >= y?=w1825:bool)
    n2290 = local read "Boat level"() -> (w1833:i32)
    n2291 = Greater Or Equal?(x=w1727, y=3.0) -> (x >= y?=w1725:bool)
    n2292 = Greater Or Equal?(x=w592, y=4.0) -> (x >= y?=w593:bool)
    n2293 = Greater Or Equal?(x=w1785, y=4.0) -> (x >= y?=w1786:bool)
    n2294 = Greater Or Equal?(x=w646, y=1) -> (x >= y?=w653:bool)
    n2295 = local read "Boat level"() -> (w585:i32)
    n2296 = And(x="Taxes level 6", y=w653) -> (x .and. y?=w648:bool)
    n2297 = Greater Or Equal?(x=w596, y=3.0) -> (x >= y?=w598:bool)
    n2298 = Greater Or Equal?(x=w1878, y=3.0) -> (x >= y?=w1852:bool)
    n2299 = Increment(x=w1935) -> (x+1=w1934:i32)
    n2300 = Not Equal?(x=w651, y=w652) -> (x != y?=w649:bool)
    n2301 = And(x=w649, y=w648) -> (x .and. y?=w650:bool)
    n2302 = Greater Or Equal?(x=w511, y=w510) -> (x >= y?=w506:bool)
    n2303 = Greater Or Equal?(x=w498, y=w499) -> (x >= y?=w503:bool)
    n2304 = Subtract(x=w511, y=w510) -> (x-y=w509:dbl)
    n2305 = Subtract(x=w498, y=w499) -> (x-y=w500:dbl)
    n2306 = Equal?(x=w513, y=2.0) -> (x = y?=w508:bool)
    n2307 = Greater Or Equal?(x=w556, y=w557) -> (x >= y?=w561:bool)
    n2308 = Compound Arithmetic op=AND(w508, "Mechanical\nTelevision", w517, w520, w506) -> (w505:bool)
    n2309 = Equal?(x=w496, y=3.0) -> (x = y?=w501:bool)
    n2310 = Compound Arithmetic op=AND(w501, "LCD monitor", w492, w489, w503) -> (w504:bool)
    n2311 = local read "EP"() -> (w1874:dbl)
    n2312 = Greater Or Equal?(x=w536, y=w537) -> (x >= y?=w541:bool)
    n2313 = Increment(x=w513) -> (x+1=w512:i32)
    n2314 = Subtract(x=w556, y=w557) -> (x-y=w558:dbl)
    n2315 = Increment(x=w496) -> (x+1=w497:i32)
    n2316 = Equal?(x=w554, y=0.0) -> (x = y?=w559:bool)
    n2317 = Subtract(x=w536, y=w537) -> (x-y=w538:dbl)
    n2318 = Compound Arithmetic op=AND(w559, "Telescope", w568, w527, w561) -> (w562:bool)
    n2319 = local read "EP"() -> (w1831:dbl)
    n2320 = Equal?(x=w534, y=1.0) -> (x = y?=w539:bool)
    n2321 = Compound Arithmetic op=AND(w539, "Camera", w530, w521, w541) -> (w542:bool)
    n2322 = case shown="True" w1936 {
      tunnel: w1940 -> [_ w3495]
      tunnel: w1934 -> [_ w3493]
      frame False {
      }
      frame True {
        w3489 = 0.25
        n2323 = local read "warrior a"() -> (w3490:dbl)
        n2324 = local read "hunting a"() -> (w3488:dbl)
        n2325 = local write "Spear level"(w3493) -> ()
        n2326 = Subtract(x=w3495, y=3000.0) -> (x-y=w3494:dbl)
        n2327 = local write "EP"(w3494) -> ()
        n2328 = Add(x=w3489, y=w3490) -> (x+y=w3491:dbl)
        n2329 = Add(x=w3489, y=w3488) -> (x+y=w3492:dbl)
        n2330 = local write "warrior a"(w3491) -> ()
        n2331 = local write "hunting a"(w3492) -> ()
      }
    }
    n2332 = Increment(x=w534) -> (x+1=w535:i32)
    n2333 = local read "EP"() -> (w587:dbl)
    n2334 = local read "EP"() -> (w1780:dbl)
    n2335 = Increment(x=w554) -> (x+1=w555:i32)
    n2336 = case shown="True" w650 {
      tunnel: w652 -> [_ w2834]
      frame False {
      }
      frame True {
        n2337 = local write "Taxation\nlevel"(w2834) -> ()
        n2338 = local write "Taxes dissent mod"(60.0 ("Taxes dissent add mod")) -> ()
      }
    }
    n2339 = Greater Or Equal?(x=w1874, y=w1873) -> (x >= y?=w1850:bool)
    n2340 = Subtract(x=w1874, y=w1873) -> (x-y=w1872:dbl)
    n2341 = Equal?(x=w1876, y=1.0) -> (x = y?=w1857:bool)
    n2342 = Greater Or Equal?(x=w1831, y=w1830) -> (x >= y?=w1824:bool)
    n2343 = Compound Arithmetic op=AND(w1857, "Bow 2", w1852, w1851, w1850) -> (w1849:bool)
    n2344 = Increment(x=w1876) -> (x+1=w1875:i32)
    n2345 = Subtract(x=w1831, y=w1830) -> (x-y=w1829:dbl)
    n2346 = case shown="True" w562 {
      tunnel: w555 -> [_ w2806]
      tunnel: w558 -> [_ w2805]
      frame False {
      }
      frame True {
        n2347 = local write "EP"(w2805) -> ()
        n2348 = local write "Optics\nlevel"(w2806) -> ()
      }
    }
    n2349 = Equal?(x=w1833, y=1.0) -> (x = y?=w1828:bool)
    n2350 = Compound Arithmetic op=AND(w1828, "Trireme", w1825, w1725, w1824) -> (w1823:bool)
    n2351 = Greater Or Equal?(x=w587, y=w588) -> (x >= y?=w594:bool)
    n2352 = Greater Or Equal?(x=w1780, y=w1781) -> (x >= y?=w1787:bool)
    n2353 = Increment(x=w1833) -> (x+1=w1832:i32)
    n2354 = Subtract(x=w587, y=w588) -> (x-y=w589:dbl)
    n2355 = Subtract(x=w1780, y=w1781) -> (x-y=w1782:dbl)
    n2356 = case shown="True" w505 {
      tunnel: w512 -> [_ w2800]
      tunnel: w509 -> [_ w2799]
      frame False {
      }
      frame True {
        n2357 = local write "EP"(w2799) -> ()
        n2358 = local write "Optics\nlevel"(w2800) -> ()
      }
    }
    n2359 = Equal?(x=w585, y=3.0) -> (x = y?=w590:bool)
    n2360 = Equal?(x=w1778, y=1.0) -> (x = y?=w1783:bool)
    n2361 = case shown="True" w504 {
      tunnel: w497 -> [_ w2798]
      tunnel: w500 -> [_ w2797]
      frame False {
      }
      frame True {
        n2362 = local write "EP"(w2797) -> ()
        n2363 = local write "Optics\nlevel"(w2798) -> ()
      }
    }
    n2364 = Compound Arithmetic op=AND(w590, "Steamship", w593, w598, w594) -> (w595:bool)
    n2365 = Compound Arithmetic op=AND(w1783, "Farming 2", w1786, w1787) -> (w1788:bool)
    n2366 = Increment(x=w585) -> (x+1=w586:i32)
    n2367 = Increment(x=w1778) -> (x+1=w1779:i32)
    n2368 = case shown="True" w542 {
      tunnel: w535 -> [_ w2802]
      tunnel: w538 -> [_ w2801]
      frame False {
      }
      frame True {
        n2369 = local write "EP"(w2801) -> ()
        n2370 = local write "Optics\nlevel"(w2802) -> ()
      }
    }
    n2371 = case shown="True" w1823 {
      tunnel: w1832 -> [_ w3441]
      tunnel: w1829 -> [_ w3440]
      frame False {
      }
      frame True {
        n2372 = local read "Trading level no mod"() -> (w3439:i32)
        n2373 = local read "Military Modifier"() -> (w3436:dbl)
        n2374 = local write "EP"(w3440) -> ()
        n2375 = local write "Boat level"(w3441) -> ()
        n2376 = Increment(x=w3439) -> (x+1=w3438:i32)
        n2377 = local write "Trading level no mod"(w3438) -> ()
        n2378 = Multiply(x=1.125, y=w3436) -> (x*y=w3437:dbl)
        n2379 = local write "Military Modifier"(w3437) -> ()
      }
    }
    n2380 = local read "Military\nScience level"() -> (w1263:i32)
    n2381 = case shown="True" w595 {
      tunnel: w586 -> [_ w2814]
      tunnel: w589 -> [_ w2813]
      frame False {
      }
      frame True {
        n2382 = local read "Trading level no mod"() -> (w2807:i32)
        n2383 = local write "EP"(w2813) -> ()
        n2384 = local read "warrior b"() -> (w2811:dbl)
        n2385 = local write "Boat level"(w2814) -> ()
        n2386 = Add(x=0.5, y=w2811) -> (x+y=w2812:dbl)
        n2387 = Increment(x=w2807) -> (x+1=w2808:i32)
        n2388 = Increment(x=w2808) -> (x+1=w2809:i32)
        n2389 = local write "Trading level no mod"(w2809) -> ()
        n2390 = local write "warrior b"(w2812) -> ()
      }
    }
    n2391 = case shown="True" w1849 {
      tunnel: w1875 -> [_ w3465]
      tunnel: w1872 -> [_ w3464]
      frame False {
      }
      frame True {
        w3459 = 0.5 ("x")
        n2392 = local read "hunting a"() -> (w3463:dbl)
        n2393 = local read "warrior a"() -> (w3460:dbl)
        n2394 = local write "EP"(w3464) -> ()
        n2395 = local write "Bow level"(w3465) -> ()
        n2396 = Add(x=w3459, y=w3463) -> (x+y=w3462:dbl)
        n2397 = Add(x=w3459, y=w3460) -> (x+y=w3461:dbl)
        n2398 = local write "hunting a"(w3462) -> ()
        n2399 = local write "warrior a"(w3461) -> ()
      }
    }
    n2400 = case shown="True" w1788 {
      tunnel: w1779 -> [_ w3414]
      tunnel: w1782 -> [_ w3413]
      frame False {
      }
      frame True {
        n2401 = local read "hunting b"() -> (w3411:dbl)
        n2402 = local read "hunting a"() -> (w3408:dbl)
        n2403 = local write "EP"(w3413) -> ()
        n2404 = local write "Farming level"(w3414) -> ()
        n2405 = Add(x=1.0, y=w3408) -> (x+y=w3407:dbl)
        n2406 = Add(x=0.5, y=w3411) -> (x+y=w3412:dbl)
        n2407 = local write "hunting b"(w3412) -> ()
        n2408 = local write "hunting a"(w3407) -> ()
      }
    }
    n2409 = local read "Physics level"() -> (w1274:i32)
    n2410 = local read "Governance\nlevel"() -> (w1470:i32)
    n2411 = local read "Governance\nlevel"() -> (w1472:i32)
    n2412 = local read "Physics level"() -> (w1864:i32)
    n2413 = local read "Governance\nlevel"() -> (w1457:i32)
    n2414 = local read "Construction\nlevel"() -> (w1871:i32)
    n2415 = local read "Government"() -> (w1452:string)
    n2416 = local read "Government"() -> (w1465:string)
    n2417 = local read "Government"() -> (w1477:string)
    n2418 = local read "SP"() -> (w1451:dbl)
    n2419 = local read "SP"() -> (w1464:dbl)
    n2420 = local read "SP"() -> (w1478:dbl)
    n2421 = local read "Military\nScience level"() -> (w1911:i32)
    n2422 = Greater Or Equal?(x=w1274, y=4.0) -> (x >= y?=w1276:bool)
    n2423 = local read "Bow level"() -> (w1265:i32)
    n2424 = Greater Or Equal?(x=w1457, y=4) -> (x >= y?=w1448:bool)
    n2425 = Greater Or Equal?(x=w1911, y=2.0) -> (x >= y?=w1912:bool)
    n2426 = Greater Or Equal?(x=w1451, y=5000000) -> (x >= y?=w1449:bool)
    n2427 = Greater Or Equal?(x=w1470, y=4) -> (x >= y?=w1461:bool)
    n2428 = Greater Or Equal?(x=w1472, y=4) -> (x >= y?=w1481:bool)
    n2429 = Greater Or Equal?(x=w1464, y=5000000) -> (x >= y?=w1462:bool)
    n2430 = Greater Or Equal?(x=w1478, y=5000000) -> (x >= y?=w1480:bool)
    n2431 = Greater Or Equal?(x=w1263, y=5.0) -> (x >= y?=w1275:bool)
    n2432 = Not Equal?(x=w1452, y=w1446) -> (x != y?=w1454:bool)
    n2433 = And(x="Bronze\nSpear", y=w1912) -> (x .and. y?=w1908:bool)
    n2434 = Not Equal?(x=w1465, y=w1459) -> (x != y?=w1467:bool)
    n2435 = Not Equal?(x=w1477, y=w1483) -> (x != y?=w1475:bool)
    n2436 = local read "SP"() -> (w1862:dbl)
    n2437 = local read "EP"() -> (w1267:dbl)
    n2438 = local read "Spear level"() -> (w1922:i32)
    n2439 = Power Of 10(x=w1864) -> (10^x=w1859:dbl)
    n2440 = local read "SP"() -> (w1869:dbl)
    n2441 = And(x=w1448, y=w1449) -> (x .and. y?=w1447:bool)
    n2442 = And(x="Confederacy", y=w1447) -> (x .and. y?=w1455:bool)
    n2443 = And(x=w1454, y=w1455) -> (x .and. y?=w1453:bool)
    n2444 = Power Of 10(x=w1871) -> (10^x=w1866:dbl)
    n2445 = case shown="True" w1453 {
      tunnel: w1446 -> [_ w3164]
      frame False {
      }
      frame True {
        n2446 = local write "Government"(w3164) -> ()
        n2447 = local read "SP"() -> (w3161:dbl)
        n2448 = Subtract(x=w3161, y=5000000) -> (x-y=w3163:dbl)
        n2449 = local write "SP"(w3163) -> ()
      }
    }
    n2450 = And(x=w1461, y=w1462) -> (x .and. y?=w1460:bool)
    n2451 = And(x="Republic", y=w1460) -> (x .and. y?=w1468:bool)
    n2452 = And(x=w1467, y=w1468) -> (x .and. y?=w1466:bool)
    n2453 = And(x=w1481, y=w1480) -> (x .and. y?=w1482:bool)
    n2454 = And(x="Kingdom", y=w1482) -> (x .and. y?=w1474:bool)
    n2455 = And(x=w1475, y=w1474) -> (x .and. y?=w1476:bool)
    n2456 = case shown="True" w1466 {
      tunnel: w1459 -> [_ w3160]
      frame False {
      }
      frame True {
        n2457 = local write "Government"(w3160) -> ()
        n2458 = local read "SP"() -> (w3159:dbl)
        n2459 = Subtract(x=w3159, y=5000000) -> (x-y=w3157:dbl)
        n2460 = local write "SP"(w3157) -> ()
      }
    }
    n2461 = case shown="True" w1476 {
      tunnel: w1483 -> [_ w3156]
      frame False {
      }
      frame True {
        n2462 = local write "Government"(w3156) -> ()
        n2463 = local read "SP"() -> (w3153:dbl)
        n2464 = Subtract(x=w3153, y=5000000) -> (x-y=w3155:dbl)
        n2465 = local write "SP"(w3155) -> ()
      }
    }
    n2466 = local read "EP"() -> (w1927:dbl)
    n2467 = Greater Or Equal?(x=w1267, y=w1268) -> (x >= y?=w1277:bool)
    n2468 = Subtract(x=w1267, y=w1268) -> (x-y=w1269:dbl)
    n2469 = Equal?(x=w1265, y=2.0) -> (x = y?=w1270:bool)
    n2470 = Compound Arithmetic op=AND(w1270, "Longbow", w1275, w1276, w1277) -> (w1278:bool)
    n2471 = Increment(x=w1265) -> (x+1=w1266:i32)
    n2472 = Greater Or Equal?(x=w1927, y=w1901) -> (x >= y?=w1928:bool)
    n2473 = And(x=w1908, y=w1928) -> (x .and. y?=w1925:bool)
    n2474 = Increment(x=w1864) -> (x+1=w1691:i32)
    n2475 = Index Array(array=w849, index=w1691) -> (element=w1690:dbl)
    n2476 = Power Of 2(x=w1690) -> (2^x=w1689:dbl)
    n2477 = Compound Arithmetic op=MULTIPLY(w1859, 1000, w1689) -> (w1863:dbl)
    n2478 = Greater?(x=w1862, y=w1863) -> (0:w1861:bool)
    n2479 = And(x="Physics", y=w1861) -> (x .and. y?=w1714:bool)
    n2480 = Equal?(x=w1922, y=2.0) -> (x = y?=w1924:bool)
    n2481 = And(x=w1924, y=w1925) -> (x .and. y?=w1923:bool)
    n2482 = local read "Physics level"() -> (w865:i32)
    n2483 = local read "Physics level"() -> (w892:i32)
    n2484 = local read "Military\nScience level"() -> (w867:i32)
    n2485 = case shown="True" w1278 {
      tunnel: w1266 -> [_ w3082]
      tunnel: w1269 -> [_ w3081]
      frame False {
      }
      frame True {
        n2486 = local write "EP"(w3081) -> ()
        n2487 = local read "warrior a"() -> (w3079:dbl)
        n2488 = local write "Bow level"(w3082) -> ()
        n2489 = Add(x=0.25, y=w3079) -> (x+y=w3080:dbl)
        n2490 = local write "warrior a"(w3080) -> ()
      }
    }
    n2491 = local read "Military\nScience level"() -> (w890:i32)
    n2492 = local read "Physics level"() -> (w897:i32)
    n2493 = local read "Military\nScience level"() -> (w899:i32)
    n2494 = local read "Physics level"() -> (w956:i32)
    n2495 = local read "Military\nScience level"() -> (w913:i32)
    n2496 = local read "Physics level"() -> (w954:i32)
    n2497 = local read "Military\nScience level"() -> (w948:i32)
    n2498 = case shown="True" w1714 {
      tunnel: w1862 -> [_ w3458]
      tunnel: w1863 -> [_ w3457]
      tunnel: w1691 -> [_ w3455]
      tunnel: [0 w3455] -> w1721
      frame False {
      }
      frame True {
        n2499 = Subtract(x=w3458, y=w3457) -> (x-y=w3456:dbl)
        n2500 = local write "SP"(w3456) -> ()
        n2501 = local write "Physics level"(w3455) -> ()
      }
    }
    n2502 = local read "Physics level"() -> (w950:i32)
    n2503 = Increment(x=w1922) -> (x+1=w1921:i32)
    n2504 = local read "Military\nScience level"() -> (w916:i32)
    n2505 = Increment(x=w1871) -> (x+1=w1688:i32)
    n2506 = Index Array(array=w849, index=w1688) -> (element=w1687:dbl)
    n2507 = Power Of 2(x=w1687) -> (2^x=w1686:dbl)
    n2508 = Compound Arithmetic op=MULTIPLY(w1866, 1000, w1686) -> (w1870:dbl)
    n2509 = Greater?(x=w1869, y=w1870) -> (0:w1868:bool)
    n2510 = And(x="Construction", y=w1868) -> (x .and. y?=w1715:bool)
    n2511 = case shown="True" w1715 {
      tunnel: w1869 -> [_ w3453]
      tunnel: w1870 -> [_ w3452]
      tunnel: w1688 -> [_ w3450]
      tunnel: [0 w3450] -> w1720
      frame False {
      }
      frame True {
        n2512 = Subtract(x=w3453, y=w3452) -> (x-y=w3451:dbl)
        n2513 = local write "SP"(w3451) -> ()
        n2514 = local write "Construction\nlevel"(w3450) -> ()
      }
    }
    n2515 = case shown="True" w1923 {
      tunnel: w1927 -> [_ w3484]
      tunnel: w1921 -> [_ w3482]
      tunnel: w1901 -> [_ w3481]
      frame False {
      }
      frame True {
        n2516 = local read "warrior a"() -> (w3486:dbl)
        n2517 = local write "Spear level"(w3482) -> ()
        n2518 = Subtract(x=w3484, y=w3481) -> (x-y=w3483:dbl)
        n2519 = local write "EP"(w3483) -> ()
        n2520 = Add(x=w3486, y=0.5) -> (x+y=w3485:dbl)
        n2521 = local write "warrior a"(w3485) -> ()
      }
    }
    n2522 = local read "Economics\nlevel"() -> (w1040:i32)
    n2523 = local read "Economics\nlevel"() -> (w1041:i32)
    n2524 = local read "Economics\nlevel"() -> (w1037:i32)
    n2525 = local read "Biology\nlevel"() -> (w1307:i32)
    n2526 = local read "Biology\nlevel"() -> (w609:i32)
    n2527 = local read "Construction\nlevel"() -> (w1279:i32)
    n2528 = local read "Biology\nlevel"() -> (w1308:i32)
    n2529 = local read "Construction\nlevel"() -> (w1520:i32)
    n2530 = local read "Biology\nlevel"() -> (w1333:i32)
    n2531 = local read "Construction\nlevel"() -> (w1521:i32)
    n2532 = local read "Physics level"() -> (w1290:i32)
    n2533 = local read "Military\nScience level"() -> (w1906:i32)
    n2534 = local read "Physics level"() -> (w1509:i32)
    n2535 = local read "Physics level"() -> (w1532:i32)
    n2536 = local read "Siege weapon\nlevel"() -> (w870:i32)
    n2537 = local read "Siege weapon\nlevel"() -> (w887:i32)
    n2538 = local read "Siege weapon\nlevel"() -> (w902:i32)
    n2539 = local read "Siege weapon\nlevel"() -> (w928:i32)
    n2540 = local read "Siege weapon\nlevel"() -> (w945:i32)
    n2541 = local read "Siege weapon\nlevel"() -> (w925:i32)
    n2542 = local read "Construction\ntools level"() -> (w1281:i32)
    n2543 = local read "Tax method\nlevel"() -> (w1008:i32)
    n2544 = local read "Tax method\nlevel"() -> (w1025:i32)
    n2545 = local read "Construction\ntools level"() -> (w1518:i32)
    n2546 = local read "Medicine level"() -> (w1305:i32)
    n2547 = local read "Medicine level"() -> (w611:i32)
    n2548 = Greater Or Equal?(x=w865, y=9.0) -> (x >= y?=w863:bool)
    n2549 = local read "Medicine level"() -> (w1310:i32)
    n2550 = Greater Or Equal?(x=w892, y=9.0) -> (x >= y?=w894:bool)
    n2551 = local read "Tax method\nlevel"() -> (w1028:i32)
    n2552 = local read "Governance\nlevel"() -> (w1421:i32)
    n2553 = Greater Or Equal?(x=w897, y=7.0) -> (x >= y?=w895:bool)
    n2554 = local read "Governance\nlevel"() -> (w1419:i32)
    n2555 = local read "Construction\ntools level"() -> (w1523:i32)
    n2556 = Greater Or Equal?(x=w956, y=6.0) -> (x >= y?=w958:bool)
    n2557 = Greater Or Equal?(x=w954, y=5.0) -> (x >= y?=w955:bool)
    n2558 = local read "Medicine level"() -> (w1331:i32)
    n2559 = Greater Or Equal?(x=w950, y=4.0) -> (x >= y?=w952:bool)
    n2560 = Greater Or Equal?(x=w867, y=9.0) -> (x >= y?=w866:bool)
    n2561 = Greater Or Equal?(x=w890, y=8.0) -> (x >= y?=w891:bool)
    n2562 = Greater Or Equal?(x=w899, y=6.0) -> (x >= y?=w898:bool)
    n2563 = Greater Or Equal?(x=w913, y=3.0) -> (x >= y?=w912:bool)
    n2564 = Greater Or Equal?(x=w948, y=4.0) -> (x >= y?=w949:bool)
    n2565 = local read "Governance\nlevel"() -> (w1434:i32)
    n2566 = Greater Or Equal?(x=w916, y=3.0) -> (x >= y?=w911:bool)
    n2567 = local read "Government"() -> (w1439:string)
    n2568 = local read "Government"() -> (w1426:string)
    n2569 = local read "Government"() -> (w1414:string)
    n2570 = local read "Economics\nlevel"() -> (w1813:i32)
    n2571 = Greater Or Equal?(x=w1040, y=4.0) -> (x >= y?=w1044:bool)
    n2572 = Greater Or Equal?(x=w1041, y=6.0) -> (x >= y?=w1043:bool)
    n2573 = local read "Biology\nlevel"() -> (w1799:i32)
    n2574 = Greater Or Equal?(x=w1290, y=5.0) -> (x >= y?=w1292:bool)
    n2575 = local read "EP"() -> (w872:dbl)
    n2576 = Greater Or Equal?(x=w1037, y=3.0) -> (x >= y?=w1045:bool)
    n2577 = local read "EP"() -> (w885:dbl)
    n2578 = Greater Or Equal?(x=w1307, y=4.0) -> (x >= y?=w1297:bool)
    n2579 = Greater Or Equal?(x=w609, y=6.0) -> (x >= y?=w619:bool)
    n2580 = local read "EP"() -> (w904:dbl)
    n2581 = Greater Or Equal?(x=w1308, y=2.0) -> (x >= y?=w1318:bool)
    n2582 = local read "EP"() -> (w930:dbl)
    n2583 = local read "EP"() -> (w943:dbl)
    n2584 = Greater Or Equal?(x=w1509, y=3.0) -> (x >= y?=w1507:bool)
    n2585 = local read "EP"() -> (w923:dbl)
    n2586 = Greater Or Equal?(x=w1906, y=4.0) -> (x >= y?=w1905:bool)
    n2587 = Greater Or Equal?(x=w1532, y=2.0) -> (x >= y?=w1534:bool)
    n2588 = local read "Military\nScience level"() -> (w636:i32)
    n2589 = Greater Or Equal?(x=w1333, y=1.0) -> (x >= y?=w1323:bool)
    n2590 = local read "SP"() -> (w1440:dbl)
    n2591 = Greater Or Equal?(x=w1279, y=5.0) -> (x >= y?=w1291:bool)
    n2592 = local read "EP"() -> (w1303:dbl)
    n2593 = local read "EP"() -> (w613:dbl)
    n2594 = local read "SP"() -> (w1427:dbl)
    n2595 = local read "SP"() -> (w1413:dbl)
    n2596 = local read "Spear level"() -> (w1919:i32)
    n2597 = local read "EP"() -> (w1312:dbl)
    n2598 = local read "EP"() -> (w1010:dbl)
    n2599 = local read "EP"() -> (w1023:dbl)
    n2600 = Greater Or Equal?(x=w1520, y=3.0) -> (x >= y?=w1508:bool)
    n2601 = local read "EP"() -> (w1030:dbl)
    n2602 = Greater Or Equal?(x=w1521, y=2.0) -> (x >= y?=w1533:bool)
    n2603 = local read "EP"() -> (w1329:dbl)
    n2604 = local read "EP"() -> (w1283:dbl)
    n2605 = local read "Physics level"() -> (w628:i32)
    n2606 = Greater Or Equal?(x=w872, y=w873) -> (x >= y?=w877:bool)
    n2607 = Greater Or Equal?(x=w885, y=w884) -> (x >= y?=w880:bool)
    n2608 = Subtract(x=w872, y=w873) -> (x-y=w874:dbl)
    n2609 = Subtract(x=w885, y=w884) -> (x-y=w883:dbl)
    n2610 = Equal?(x=w870, y=5.0) -> (x = y?=w875:bool)
    n2611 = Greater Or Equal?(x=w904, y=w905) -> (x >= y?=w909:bool)
    n2612 = Compound Arithmetic op=AND(w875, "Rocket artillery", w866, w863, w877) -> (w878:bool)
    n2613 = local read "EP"() -> (w1914:dbl)
    n2614 = Equal?(x=w887, y=4.0) -> (x = y?=w882:bool)
    n2615 = Compound Arithmetic op=AND(w882, "Howitzer", w891, w894, w880) -> (w879:bool)
    n2616 = Increment(x=w870) -> (x+1=w871:i32)
    n2617 = local read "EP"() -> (w1516:dbl)
    n2618 = Greater Or Equal?(x=w930, y=w931) -> (x >= y?=w935:bool)
    n2619 = Subtract(x=w904, y=w905) -> (x-y=w906:dbl)
    n2620 = Greater Or Equal?(x=w943, y=w942) -> (x >= y?=w938:bool)
    n2621 = Increment(x=w887) -> (x+1=w886:i32)
    n2622 = Equal?(x=w902, y=3.0) -> (x = y?=w907:bool)
    n2623 = Subtract(x=w930, y=w931) -> (x-y=w932:dbl)
    n2624 = Compound Arithmetic op=AND(w907, "Cannon", w898, w895, w909) -> (w910:bool)
    n2625 = local read "EP"() -> (w1525:dbl)
    n2626 = Greater Or Equal?(x=w923, y=w922) -> (x >= y?=w918:bool)
    n2627 = Subtract(x=w943, y=w942) -> (x-y=w941:dbl)
    n2628 = Equal?(x=w928, y=1.0) -> (x = y?=w933:bool)
    n2629 = Increment(x=w902) -> (x+1=w903:i32)
    n2630 = Compound Arithmetic op=AND(w933, "Catapult", w912, w955, w935) -> (w936:bool)
    n2631 = Equal?(x=w945, y=2.0) -> (x = y?=w940:bool)
    n2632 = And(x="Iron\nSpear", y=w1905) -> (x .and. y?=w1903:bool)
    n2633 = Subtract(x=w923, y=w922) -> (x-y=w921:dbl)
    n2634 = Compound Arithmetic op=AND(w940, "Trebuchet", w949, w958, w938) -> (w937:bool)
    n2635 = Increment(x=w928) -> (x+1=w929:i32)
    n2636 = Equal?(x=w925, y=0.0) -> (x = y?=w920:bool)
    n2637 = Increment(x=w945) -> (x+1=w944:i32)
    n2638 = Compound Arithmetic op=AND(w920, "Ballista", w911, w952, w918) -> (w917:bool)
    n2639 = Increment(x=w925) -> (x+1=w924:i32)
    n2640 = Greater Or Equal?(x=w1303, y=w1302) -> (x >= y?=w1296:bool)
    n2641 = Greater Or Equal?(x=w613, y=w614) -> (x >= y?=w620:bool)
    n2642 = Greater Or Equal?(x=w1434, y=4) -> (x >= y?=w1443:bool)
    n2643 = Greater Or Equal?(x=w1440, y=5000000) -> (x >= y?=w1442:bool)
    n2644 = Subtract(x=w1303, y=w1302) -> (x-y=w1301:dbl)
    n2645 = Subtract(x=w613, y=w614) -> (x-y=w615:dbl)
    n2646 = Greater Or Equal?(x=w1312, y=w1313) -> (x >= y?=w1319:bool)
    n2647 = Equal?(x=w1305, y=2.0) -> (x = y?=w1300:bool)
    n2648 = Equal?(x=w611, y=3.0) -> (x = y?=w616:bool)
    n2649 = Greater Or Equal?(x=w1010, y=w1011) -> (x >= y?=w1015:bool)
    n2650 = Compound Arithmetic op=AND(w1300, "Medicine 3", w1297, w1296) -> (w1295:bool)
    n2651 = Compound Arithmetic op=AND(w616, "Medicine 4", w619, w620) -> (w621:bool)
    n2652 = Greater Or Equal?(x=w1421, y=4) -> (x >= y?=w1430:bool)
    n2653 = Subtract(x=w1312, y=w1313) -> (x-y=w1314:dbl)
    n2654 = Greater Or Equal?(x=w1419, y=4) -> (x >= y?=w1410:bool)
    n2655 = Increment(x=w1305) -> (x+1=w1304:i32)
    n2656 = Increment(x=w611) -> (x+1=w612:i32)
    n2657 = Greater Or Equal?(x=w1023, y=w1022) -> (x >= y?=w1018:bool)
    n2658 = Subtract(x=w1010, y=w1011) -> (x-y=w1012:dbl)
    n2659 = Greater Or Equal?(x=w1427, y=5000000) -> (x >= y?=w1429:bool)
    n2660 = Equal?(x=w1310, y=1.0) -> (x = y?=w1315:bool)
    n2661 = Greater Or Equal?(x=w1413, y=5000000) -> (x >= y?=w1411:bool)
    n2662 = Compound Arithmetic op=AND(w1315, "Medicine 2", w1318, w1319) -> (w1320:bool)
    n2663 = Equal?(x=w1008, y=2.0) -> (x = y?=w1013:bool)
    n2664 = Subtract(x=w1023, y=w1022) -> (x-y=w1021:dbl)
    n2665 = Compound Arithmetic op=AND(w1013, "Income tax", w1043, w1015) -> (w1016:bool)
    n2666 = Increment(x=w1310) -> (x+1=w1311:i32)
    n2667 = Greater Or Equal?(x=w1030, y=w1031) -> (x >= y?=w1035:bool)
    n2668 = Equal?(x=w1025, y=1.0) -> (x = y?=w1020:bool)
    n2669 = Increment(x=w1008) -> (x+1=w1009:i32)
    n2670 = Compound Arithmetic op=AND(w1020, "Sales tax", w1044, w1018) -> (w1017:bool)
    n2671 = Greater Or Equal?(x=w1329, y=w1328) -> (x >= y?=w1322:bool)
    n2672 = Subtract(x=w1030, y=w1031) -> (x-y=w1032:dbl)
    n2673 = Increment(x=w1025) -> (x+1=w1024:i32)
    n2674 = Greater Or Equal?(x=w1283, y=w1284) -> (x >= y?=w1293:bool)
    n2675 = Equal?(x=w1028, y=0.0) -> (x = y?=w1033:bool)
    n2676 = Subtract(x=w1329, y=w1328) -> (x-y=w1327:dbl)
    n2677 = Compound Arithmetic op=AND(w1033, "Tariffs", w1045, w1035) -> (w1036:bool)
    n2678 = Not Equal?(x=w1439, y=w1445) -> (x != y?=w1437:bool)
    n2679 = Subtract(x=w1283, y=w1284) -> (x-y=w1285:dbl)
    n2680 = Equal?(x=w1331, y=0.0) -> (x = y?=w1326:bool)
    n2681 = Increment(x=w1028) -> (x+1=w1029:i32)
    n2682 = Compound Arithmetic op=AND(w1326, "Medicine 1", w1323, w1322) -> (w1321:bool)
    n2683 = Greater Or Equal?(x=w1914, y=w1902) -> (x >= y?=w1913:bool)
    n2684 = Equal?(x=w1281, y=2.0) -> (x = y?=w1286:bool)
    n2685 = And(x=w1903, y=w1913) -> (x .and. y?=w1916:bool)
    n2686 = Compound Arithmetic op=AND(w1286, "Advanced\nmetal\ntools", w1291, w1292, w1293) -> (w1294:bool)
    n2687 = Increment(x=w1331) -> (x+1=w1330:i32)
    n2688 = Not Equal?(x=w1426, y=w1432) -> (x != y?=w1424:bool)
    n2689 = Not Equal?(x=w1414, y=w1408) -> (x != y?=w1416:bool)
    n2690 = Increment(x=w1281) -> (x+1=w1282:i32)
    n2691 = Greater Or Equal?(x=w1516, y=w1515) -> (x >= y?=w1506:bool)
    n2692 = case shown="True" w878 {
      tunnel: w871 -> [_ w2939]
      tunnel: w874 -> [_ w2938]
      frame False {
      }
      frame True {
        n2693 = local write "EP"(w2938) -> ()
        n2694 = local read "warrior b"() -> (w2935:dbl)
        n2695 = local write "Siege weapon\nlevel"(w2939) -> ()
        n2696 = Add(x=w2935, y=1.0) -> (x+y=w2936:dbl)
        n2697 = local write "warrior b"(w2936) -> ()
      }
    }
    n2698 = case shown="True" w917 {
      tunnel: w924 -> [_ w2964]
      tunnel: w921 -> [_ w2963]
      frame False {
      }
      frame True {
        n2699 = local write "Siege weapon\nlevel"(w2964) -> ()
        n2700 = local write "EP"(w2963) -> ()
        n2701 = local read "warrior b"() -> (w2962:dbl)
        n2702 = Add(x=w2962, y=0.25) -> (x+y=w2961:dbl)
        n2703 = local write "warrior b"(w2961) -> ()
      }
    }
    n2704 = Subtract(x=w1516, y=w1515) -> (x-y=w1514:dbl)
    n2705 = case shown="True" w879 {
      tunnel: w886 -> [_ w2944]
      tunnel: w883 -> [_ w2943]
      frame False {
      }
      frame True {
        n2706 = local write "EP"(w2943) -> ()
        n2707 = local read "warrior b"() -> (w2940:dbl)
        n2708 = local write "Siege weapon\nlevel"(w2944) -> ()
        n2709 = Add(x=w2940, y=1.0) -> (x+y=w2941:dbl)
        n2710 = local write "warrior b"(w2941) -> ()
      }
    }
    n2711 = Greater Or Equal?(x=w1525, y=w1526) -> (x >= y?=w1535:bool)
    n2712 = Equal?(x=w1518, y=1.0) -> (x = y?=w1513:bool)
    n2713 = Compound Arithmetic op=AND(w1513, "Basic\nmetal\ntools", w1508, w1507, w1506) -> (w1505:bool)
    n2714 = Subtract(x=w1525, y=w1526) -> (x-y=w1527:dbl)
    n2715 = case shown="True" w910 {
      tunnel: w903 -> [_ w2949]
      tunnel: w906 -> [_ w2948]
      frame False {
      }
      frame True {
        n2716 = local write "EP"(w2948) -> ()
        n2717 = local read "warrior b"() -> (w2945:dbl)
        n2718 = local write "Siege weapon\nlevel"(w2949) -> ()
        n2719 = Add(x=w2945, y=1.0) -> (x+y=w2946:dbl)
        n2720 = local write "warrior b"(w2946) -> ()
      }
    }
    n2721 = Increment(x=w1518) -> (x+1=w1517:i32)
    n2722 = Equal?(x=w1523, y=0.0) -> (x = y?=w1528:bool)
    n2723 = Equal?(x=w1919, y=3.0) -> (x = y?=w1917:bool)
    n2724 = And(x=w1917, y=w1916) -> (x .and. y?=w1918:bool)
    n2725 = Compound Arithmetic op=AND(w1528, "Stone tools", w1533, w1534, w1535) -> (w1536:bool)
    n2726 = case shown="True" w936 {
      tunnel: w929 -> [_ w2959]
      tunnel: w932 -> [_ w2958]
      frame False {
      }
      frame True {
        n2727 = local write "EP"(w2958) -> ()
        n2728 = local read "warrior b"() -> (w2955:dbl)
        n2729 = local write "Siege weapon\nlevel"(w2959) -> ()
        n2730 = Add(x=w2955, y=0.5) -> (x+y=w2956:dbl)
        n2731 = local write "warrior b"(w2956) -> ()
      }
    }
    n2732 = case shown="True" w1295 {
      tunnel: w1304 -> [_ w3090]
      tunnel: w1301 -> [_ w3089]
      frame False {
      }
      frame True {
        n2733 = local write "EP"(w3089) -> ()
        n2734 = local write "Medicine level"(w3090) -> ()
        n2735 = local write "Medicine dissent mod"(0.8 ("Medicine dissent mod")) -> ()
      }
    }
    n2736 = case shown="True" w621 {
      tunnel: w612 -> [_ w2827]
      tunnel: w615 -> [_ w2826]
      frame False {
      }
      frame True {
        n2737 = local write "EP"(w2826) -> ()
        n2738 = local write "Medicine level"(w2827) -> ()
        n2739 = local write "Medicine dissent mod"(0.75 ("Medicine dissent mod")) -> ()
      }
    }
    n2740 = case shown="True" w937 {
      tunnel: w944 -> [_ w2954]
      tunnel: w941 -> [_ w2953]
      frame False {
      }
      frame True {
        n2741 = local write "EP"(w2953) -> ()
        n2742 = local read "warrior b"() -> (w2952:dbl)
        n2743 = local write "Siege weapon\nlevel"(w2954) -> ()
        n2744 = Add(x=w2952, y=0.5) -> (x+y=w2951:dbl)
        n2745 = local write "warrior b"(w2951) -> ()
      }
    }
    n2746 = Increment(x=w1523) -> (x+1=w1524:i32)
    n2747 = case shown="True" w1320 {
      tunnel: w1311 -> [_ w3093]
      tunnel: w1314 -> [_ w3092]
      frame False {
      }
      frame True {
        n2748 = local write "EP"(w3092) -> ()
        n2749 = local write "Medicine level"(w3093) -> ()
        n2750 = local write "Medicine dissent mod"(0.85 ("Medicine dissent mod")) -> ()
      }
    }
    n2751 = And(x=w1443, y=w1442) -> (x .and. y?=w1444:bool)
    n2752 = And(x="Feudalism", y=w1444) -> (x .and. y?=w1436:bool)
    n2753 = And(x=w1437, y=w1436) -> (x .and. y?=w1438:bool)
    n2754 = And(x=w1430, y=w1429) -> (x .and. y?=w1431:bool)
    n2755 = And(x="Caste system", y=w1431) -> (x .and. y?=w1423:bool)
    n2756 = And(x=w1424, y=w1423) -> (x .and. y?=w1425:bool)
    n2757 = And(x=w1410, y=w1411) -> (x .and. y?=w1409:bool)
    n2758 = And(x="Senate", y=w1409) -> (x .and. y?=w1417:bool)
    n2759 = And(x=w1416, y=w1417) -> (x .and. y?=w1415:bool)
    n2760 = case shown="True" w1036 {
      tunnel: w1029 -> [_ w2985]
      tunnel: w1032 -> [_ w2984]
      frame False {
      }
      frame True {
        n2761 = local write "EP"(w2984) -> ()
        n2762 = local write "Tax method\nlevel"(w2985) -> ()
      }
    }
    n2763 = case shown="True" w1438 {
      tunnel: w1445 -> [_ w3152]
      frame False {
      }
      frame True {
        n2764 = local write "Government"(w3152) -> ()
        n2765 = local read "SP"() -> (w3149:dbl)
        n2766 = Subtract(x=w3149, y=5000000) -> (x-y=w3151:dbl)
        n2767 = local write "SP"(w3151) -> ()
      }
    }
    n2768 = case shown="True" w1321 {
      tunnel: w1330 -> [_ w3096]
      tunnel: w1327 -> [_ w3095]
      frame False {
      }
      frame True {
        n2769 = local write "EP"(w3095) -> ()
        n2770 = local write "Medicine level"(w3096) -> ()
        n2771 = local write "Medicine dissent mod"(0.9 ("Medicine dissent mod")) -> ()
      }
    }
    n2772 = local read "SP"() -> (w1797:dbl)
    n2773 = case shown="True" w1016 {
      tunnel: w1009 -> [_ w2981]
      tunnel: w1012 -> [_ w2980]
      frame False {
      }
      frame True {
        n2774 = local write "EP"(w2980) -> ()
        n2775 = local write "Tax method\nlevel"(w2981) -> ()
      }
    }
    n2776 = local read "SP"() -> (w1815:dbl)
    n2777 = case shown="True" w1425 {
      tunnel: w1432 -> [_ w3148]
      frame False {
      }
      frame True {
        n2778 = local write "Government"(w3148) -> ()
        n2779 = local read "SP"() -> (w3147:dbl)
        n2780 = Subtract(x=w3147, y=5000000) -> (x-y=w3145:dbl)
        n2781 = local write "SP"(w3145) -> ()
      }
    }
    n2782 = case shown="True" w1415 {
      tunnel: w1408 -> [_ w3144]
      frame False {
      }
      frame True {
        n2783 = local write "Government"(w3144) -> ()
        n2784 = local read "SP"() -> (w3141:dbl)
        n2785 = Subtract(x=w3141, y=5000000) -> (x-y=w3143:dbl)
        n2786 = local write "SP"(w3143) -> ()
      }
    }
    n2787 = case shown="True" w1017 {
      tunnel: w1024 -> [_ w2983]
      tunnel: w1021 -> [_ w2982]
      frame False {
      }
      frame True {
        n2788 = local write "EP"(w2982) -> ()
        n2789 = local write "Tax method\nlevel"(w2983) -> ()
      }
    }
    n2790 = Power Of 10(x=w1799) -> (10^x=w1794:dbl)
    n2791 = Power Of 10(x=w1813) -> (10^x=w1819:dbl)
    n2792 = Increment(x=w1919) -> (x+1=w1920:i32)
    n2793 = case shown="True" w1536 {
      tunnel: w1524 -> [_ w3176]
      tunnel: w1527 -> [_ w3175]
      frame False {
      }
      frame True {
        n2794 = local read "Construction multiplier"() -> (w3173:dbl)
        n2795 = local write "Construction\ntools level"(w3176) -> ()
        n2796 = local write "EP"(w3175) -> ()
        n2797 = Add(x=w3173, y=0.25) -> (x+y=w3172:dbl)
        n2798 = local write "Construction multiplier"(w3172) -> ()
      }
    }
    n2799 = case shown="True" w1294 {
      tunnel: w1282 -> [_ w3087]
      tunnel: w1285 -> [_ w3086]
      frame False {
      }
      frame True {
        n2800 = local read "Construction multiplier"() -> (w3084:dbl)
        n2801 = local write "Construction\ntools level"(w3087) -> ()
        n2802 = local write "EP"(w3086) -> ()
        n2803 = Add(x=w3084, y=0.5) -> (x+y=w3085:dbl)
        n2804 = local write "Construction multiplier"(w3085) -> ()
      }
    }
    n2805 = case shown="True" w1918 {
      tunnel: w1914 -> [_ w3477]
      tunnel: w1920 -> [_ w3475]
      tunnel: w1902 -> [_ w3474]
      frame False {
      }
      frame True {
        n2806 = local read "warrior a"() -> (w3479:dbl)
        n2807 = local write "Spear level"(w3475) -> ()
        n2808 = Subtract(x=w3477, y=w3474) -> (x-y=w3476:dbl)
        n2809 = local write "EP"(w3476) -> ()
        n2810 = Add(x=w3479, y=0.5) -> (x+y=w3478:dbl)
        n2811 = local write "warrior a"(w3478) -> ()
      }
    }
    n2812 = case shown="True" w1505 {
      tunnel: w1517 -> [_ w3171]
      tunnel: w1514 -> [_ w3170]
      frame False {
      }
      frame True {
        n2813 = local read "Construction multiplier"() -> (w3168:dbl)
        n2814 = local write "Construction\ntools level"(w3171) -> ()
        n2815 = local write "EP"(w3170) -> ()
        n2816 = Add(x=w3168, y=0.25) -> (x+y=w3169:dbl)
        n2817 = local write "Construction multiplier"(w3169) -> ()
      }
    }
    n2818 = Greater Or Equal?(x=w628, y=5.0) -> (x >= y?=w626:bool)
    n2819 = local read "Bow level"() -> (w623:i32)
    n2820 = Greater Or Equal?(x=w636, y=6.0) -> (x >= y?=w627:bool)
    n2821 = Increment(x=w1799) -> (x+1=w1682:i32)
    n2822 = Index Array(array=w849, index=w1682) -> (element=w1681:dbl)
    n2823 = Power Of 2(x=w1681) -> (2^x=w1680:dbl)
    n2824 = Compound Arithmetic op=MULTIPLY(w1794, 1000, w1680) -> (w1798:dbl)
    n2825 = Greater?(x=w1797, y=w1798) -> (0:w1796:bool)
    n2826 = And(x="Biology", y=w1796) -> (x .and. y?=w1717:bool)
    n2827 = local read "EP"() -> (w634:dbl)
    n2828 = Increment(x=w1813) -> (x+1=w1685:i32)
    n2829 = Index Array(array=w849, index=w1685) -> (element=w1684:dbl)
    n2830 = Power Of 2(x=w1684) -> (2^x=w1683:dbl)
    n2831 = Compound Arithmetic op=MULTIPLY(w1819, 1000, w1683) -> (w1814:dbl)
    n2832 = Greater?(x=w1815, y=w1814) -> (0:w1817:bool)
    n2833 = And(x="Economics", y=w1817) -> (x .and. y?=w1816:bool)
    n2834 = case shown="True" w1717 {
      tunnel: w1797 -> [_ w3419]
      tunnel: w1798 -> [_ w3418]
      tunnel: w1682 -> [_ w3416]
      tunnel: [0 w3416] -> w1718
      frame False {
      }
      frame True {
        n2835 = Subtract(x=w3419, y=w3418) -> (x-y=w3417:dbl)
        n2836 = local write "SP"(w3417) -> ()
        n2837 = local write "Biology\nlevel"(w3416) -> ()
      }
    }
    n2838 = case shown="True" w1816 {
      selector: w1816 -> [w3428 w3431]
      tunnel: w1815 -> [_ w3434]
      tunnel: w1814 -> [_ w3433]
      tunnel: w1685 -> [_ w3430]
      tunnel: [w3428 w3431] -> w1716
      tunnel: [0 w3430] -> w1719
      frame False {
      }
      frame True {
        n2839 = Subtract(x=w3434, y=w3433) -> (x-y=w3432:dbl)
        n2840 = local write "SP"(w3432) -> ()
        n2841 = local write "Economics\nlevel"(w3430) -> ()
      }
    }
    n2842 = Compound Arithmetic op=OR(w1712, w1713, w1714, w1715, w1716, w1717) -> (w1724:bool)
    n2843 = Greater Or Equal?(x=w634, y=w569) -> (x >= y?=w625:bool)
    n2844 = Subtract(x=w634, y=w569) -> (x-y=w633:dbl)
    n2845 = Equal?(x=w623, y=3.0) -> (x = y?=w632:bool)
    n2846 = Compound Arithmetic op=AND(w632, "Crossbow", w627, w626, w625) -> (w624:bool)
    n2847 = Increment(x=w623) -> (x+1=w622:i32)
    n2848 = case shown="True" w624 {
      tunnel: w622 -> [_ w2832]
      tunnel: w633 -> [_ w2831]
      frame False {
      }
      frame True {
        n2849 = local write "EP"(w2831) -> ()
        n2850 = local read "warrior a"() -> (w2829:dbl)
        n2851 = local write "Bow level"(w2832) -> ()
        n2852 = Add(x=0.25, y=w2829) -> (x+y=w2830:dbl)
        n2853 = local write "warrior a"(w2830) -> ()
      }
    }
    n2854 = local read "Governance\nlevel"() -> (w319:i32)
    n2855 = local read "Governance\nlevel"() -> (w321:i32)
    n2856 = local read "Governance\nlevel"() -> (w307:i32)
    n2857 = local read "Government"() -> (w302:string)
    n2858 = local read "Military\nScience level"() -> (w1051:i32)
    n2859 = local read "Military\nScience level"() -> (w1050:i32)
    n2860 = local read "Biology\nlevel"() -> (w1062:i32)
    n2861 = local read "Government"() -> (w314:string)
    n2862 = local read "Government"() -> (w326:string)
    n2863 = local read "Biology\nlevel"() -> (w1057:i32)
    n2864 = local read "Physics level"() -> (w961:i32)
    n2865 = local read "Military\nScience level"() -> (w1004:i32)
    n2866 = local read "Physics level"() -> (w963:i32)
    n2867 = local read "Military\nScience level"() -> (w1054:i32)
    n2868 = local read "Biology\nlevel"() -> (w1060:i32)
    n2869 = local read "Physics level"() -> (w967:i32)
    n2870 = local read "Military\nScience level"() -> (w1001:i32)
    n2871 = local read "Economics\nlevel"() -> (w969:i32)
    n2872 = local read "SP"() -> (w301:dbl)
    n2873 = local read "SP"() -> (w313:dbl)
    n2874 = local read "SP"() -> (w327:dbl)
    n2875 = local read "Production\nlevel"() -> (w852:i32)
    n2876 = local read "Animal\ndomestication\nlevel"() -> (w1095:i32)
    n2877 = local read "Animal\ndomestication\nlevel"() -> (w1112:i32)
    n2878 = local read "Animal\ndomestication\nlevel"() -> (w1115:i32)
    n2879 = local read "Writing level"() -> (w600:i32)
    n2880 = local read "Writing level"() -> (w1152:i32)
    n2881 = Greater Or Equal?(x=w307, y=6) -> (x >= y?=w299:bool)
    n2882 = Greater Or Equal?(x=w301, y=w294) -> (x >= y?=w300:bool)
    n2883 = local read "Writing level"() -> (w1135:i32)
    n2884 = Greater Or Equal?(x=w319, y=6) -> (x >= y?=w311:bool)
    n2885 = Greater Or Equal?(x=w321, y=6) -> (x >= y?=w329:bool)
    n2886 = Greater Or Equal?(x=w313, y=w295) -> (x >= y?=w312:bool)
    n2887 = Greater Or Equal?(x=w327, y=w296) -> (x >= y?=w328:bool)
    n2888 = Not Equal?(x=w302, y=w297) -> (x != y?=w304:bool)
    n2889 = local read "Writing level"() -> (w1132:i32)
    n2890 = Not Equal?(x=w314, y=w309) -> (x != y?=w316:bool)
    n2891 = Not Equal?(x=w326, y=w331) -> (x != y?=w324:bool)
    n2892 = local read "Sword level"() -> (w1092:i32)
    n2893 = local read "Sword level"() -> (w1075:i32)
    n2894 = local read "Chariot level"() -> (w989:i32)
    n2895 = local read "Chariot level"() -> (w972:i32)
    n2896 = And(x=w299, y=w300) -> (x .and. y?=w298:bool)
    n2897 = And(x="Free market capitalism", y=w298) -> (x .and. y?=w305:bool)
    n2898 = And(x=w304, y=w305) -> (x .and. y?=w303:bool)
    n2899 = local read "Sword level"() -> (w1072:i32)
    n2900 = local read "Chariot level"() -> (w992:i32)
    n2901 = And(x=w311, y=w312) -> (x .and. y?=w310:bool)
    n2902 = And(x="Imperialism", y=w310) -> (x .and. y?=w317:bool)
    n2903 = And(x=w316, y=w317) -> (x .and. y?=w315:bool)
    n2904 = And(x=w329, y=w328) -> (x .and. y?=w330:bool)
    n2905 = And(x="Empire", y=w330) -> (x .and. y?=w323:bool)
    n2906 = And(x=w324, y=w323) -> (x .and. y?=w325:bool)
    n2907 = case shown="True" w303 {
      tunnel: w297 -> [_ w2200]
      tunnel: w294 -> [_ w2197]
      frame False {
      }
      frame True {
        n2908 = local write "Government"(w2200) -> ()
        n2909 = local read "SP"() -> (w2198:dbl)
        n2910 = Subtract(x=w2198, y=w2197) -> (x-y=w2199:dbl)
        n2911 = local write "SP"(w2199) -> ()
      }
    }
    n2912 = case shown="True" w315 {
      tunnel: w309 -> [_ w2196]
      tunnel: w295 -> [_ w2193]
      frame False {
      }
      frame True {
        n2913 = local write "Government"(w2196) -> ()
        n2914 = local read "SP"() -> (w2195:dbl)
        n2915 = Subtract(x=w2195, y=w2193) -> (x-y=w2194:dbl)
        n2916 = local write "SP"(w2194) -> ()
      }
    }
    n2917 = case shown="True" w325 {
      tunnel: w331 -> [_ w2192]
      tunnel: w296 -> [_ w2189]
      frame False {
      }
      frame True {
        n2918 = local write "Government"(w2192) -> ()
        n2919 = local read "SP"() -> (w2190:dbl)
        n2920 = Subtract(x=w2190, y=w2189) -> (x-y=w2191:dbl)
        n2921 = local write "SP"(w2191) -> ()
      }
    }
    n2922 = Greater Or Equal?(x=w1062, y=1.0) -> (x >= y?=w1061:bool)
    n2923 = Greater Or Equal?(x=w1057, y=3.0) -> (x >= y?=w1055:bool)
    n2924 = Greater Or Equal?(x=w961, y=4.0) -> (x >= y?=w959:bool)
    n2925 = Greater Or Equal?(x=w963, y=4.0) -> (x >= y?=w962:bool)
    n2926 = Greater Or Equal?(x=w1060, y=2.0) -> (x >= y?=w1056:bool)
    n2927 = Greater Or Equal?(x=w967, y=3.0) -> (x >= y?=w965:bool)
    n2928 = Greater Or Equal?(x=w1051, y=4.0) -> (x >= y?=w1047:bool)
    n2929 = Greater Or Equal?(x=w1050, y=6.0) -> (x >= y?=w1048:bool)
    n2930 = local read "EP"() -> (w1150:dbl)
    n2931 = local read "EP"() -> (w602:dbl)
    n2932 = Greater Or Equal?(x=w1004, y=3.0) -> (x >= y?=w1005:bool)
    n2933 = Greater Or Equal?(x=w969, y=4.0) -> (x >= y?=w968:bool)
    n2934 = Greater Or Equal?(x=w1054, y=3.0) -> (x >= y?=w1046:bool)
    n2935 = local read "EP"() -> (w1137:dbl)
    n2936 = local read "SP"() -> (w854:dbl)
    n2937 = local read "EP"() -> (w1130:dbl)
    n2938 = Greater Or Equal?(x=w1001, y=3.0) -> (x >= y?=w1006:bool)
    n2939 = Power Of 10(x=w852) -> (10^x=w857:dbl)
    n2940 = local read "EP"() -> (w1097:dbl)
    n2941 = local read "EP"() -> (w1110:dbl)
    n2942 = local read "EP"() -> (w1117:dbl)
    n2943 = local read "EP"() -> (w1090:dbl)
    n2944 = local read "EP"() -> (w1077:dbl)
    n2945 = local read "EP"() -> (w1070:dbl)
    n2946 = local read "EP"() -> (w987:dbl)
    n2947 = local read "EP"() -> (w974:dbl)
    n2948 = Greater Or Equal?(x=w1150, y=w1149) -> (x >= y?=w1145:bool)
    n2949 = Greater Or Equal?(x=w602, y=w603) -> (x >= y?=w607:bool)
    n2950 = local read "EP"() -> (w994:dbl)
    n2951 = Subtract(x=w1150, y=w1149) -> (x-y=w1148:dbl)
    n2952 = Subtract(x=w602, y=w603) -> (x-y=w604:dbl)
    n2953 = Equal?(x=w1152, y=2.0) -> (x = y?=w1147:bool)
    n2954 = Equal?(x=w600, y=3.0) -> (x = y?=w605:bool)
    n2955 = Compound Arithmetic op=AND(w1147, "Movable typeset", w1145) -> (w1144:bool)
    n2956 = Compound Arithmetic op=AND(w605, "Printing\nPress", w607) -> (w608:bool)
    n2957 = Greater Or Equal?(x=w1137, y=w1138) -> (x >= y?=w1142:bool)
    n2958 = Increment(x=w1152) -> (x+1=w1151:i32)
    n2959 = Increment(x=w600) -> (x+1=w601:i32)
    n2960 = Subtract(x=w1137, y=w1138) -> (x-y=w1139:dbl)
    n2961 = Greater Or Equal?(x=w1130, y=w1129) -> (x >= y?=w1125:bool)
    n2962 = Equal?(x=w1135, y=1.0) -> (x = y?=w1140:bool)
    n2963 = Compound Arithmetic op=AND(w1140, "Paper", w1142) -> (w1143:bool)
    n2964 = Subtract(x=w1130, y=w1129) -> (x-y=w1128:dbl)
    n2965 = Greater Or Equal?(x=w1097, y=w1098) -> (x >= y?=w1102:bool)
    n2966 = Increment(x=w1135) -> (x+1=w1136:i32)
    n2967 = Equal?(x=w1132, y=0.0) -> (x = y?=w1127:bool)
    n2968 = Compound Arithmetic op=AND(w1127, "Parchment", w1125) -> (w1124:bool)
    n2969 = Greater Or Equal?(x=w1110, y=w1109) -> (x >= y?=w1105:bool)
    n2970 = Increment(x=w1132) -> (x+1=w1131:i32)
    n2971 = Equal?(x=w1095, y=2.0) -> (x = y?=w1100:bool)
    n2972 = Subtract(x=w1097, y=w1098) -> (x-y=w1099:dbl)
    n2973 = Subtract(x=w1110, y=w1109) -> (x-y=w1108:dbl)
    n2974 = Compound Arithmetic op=AND(w1100, "Selective\nbreeding", w1055, w1102) -> (w1103:bool)
    n2975 = Greater Or Equal?(x=w1117, y=w1118) -> (x >= y?=w1122:bool)
    n2976 = Equal?(x=w1112, y=1.0) -> (x = y?=w1107:bool)
    n2977 = Increment(x=w1095) -> (x+1=w1096:i32)
    n2978 = Compound Arithmetic op=AND(w1107, "Horses", w1105, w1056) -> (w1104:bool)
    n2979 = Subtract(x=w1117, y=w1118) -> (x-y=w1119:dbl)
    n2980 = Increment(x=w1112) -> (x+1=w1111:i32)
    n2981 = Equal?(x=w1115, y=0.0) -> (x = y?=w1120:bool)
    n2982 = Compound Arithmetic op=AND(w1120, "Livestock", w1122, w1061) -> (w1123:bool)
    n2983 = Increment(x=w852) -> (x+1=w859:i32)
    n2984 = Index Array(array=w849, index=w859) -> (element=w860:dbl)
    n2985 = Power Of 2(x=w860) -> (2^x=w861:dbl)
    n2986 = Compound Arithmetic op=MULTIPLY(w857, 1000, w861) -> (w853:dbl)
    n2987 = Greater?(x=w854, y=w853) -> (0:w855:bool)
    n2988 = And(x="Production", y=w855) -> (x .and. y?=w850:bool)
    n2989 = Increment(x=w1115) -> (x+1=w1116:i32)
    n2990 = Greater Or Equal?(x=w1090, y=w1089) -> (x >= y?=w1085:bool)
    n2991 = Greater Or Equal?(x=w1077, y=w1078) -> (x >= y?=w1082:bool)
    n2992 = Subtract(x=w1090, y=w1089) -> (x-y=w1088:dbl)
    n2993 = Equal?(x=w1092, y=2.0) -> (x = y?=w1087:bool)
    n2994 = Subtract(x=w1077, y=w1078) -> (x-y=w1079:dbl)
    n2995 = Compound Arithmetic op=AND(w1087, "Steel sword", w1048, w1085) -> (w1084:bool)
    n2996 = Greater Or Equal?(x=w1070, y=w1069) -> (x >= y?=w1065:bool)
    n2997 = Equal?(x=w1075, y=1.0) -> (x = y?=w1080:bool)
    n2998 = Increment(x=w1092) -> (x+1=w1091:i32)
    n2999 = Compound Arithmetic op=AND(w1080, "Iron sword", w1047, w1082) -> (w1083:bool)
    n3000 = Subtract(x=w1070, y=w1069) -> (x-y=w1068:dbl)
    n3001 = Greater Or Equal?(x=w987, y=w986) -> (x >= y?=w982:bool)
    n3002 = Increment(x=w1075) -> (x+1=w1076:i32)
    n3003 = Greater Or Equal?(x=w974, y=w975) -> (x >= y?=w979:bool)
    n3004 = Equal?(x=w1072, y=0.0) -> (x = y?=w1067:bool)
    n3005 = Compound Arithmetic op=AND(w1067, "Bronze sword", w1046, w1065) -> (w1064:bool)
    n3006 = Subtract(x=w987, y=w986) -> (x-y=w985:dbl)
    n3007 = Greater Or Equal?(x=w994, y=w995) -> (x >= y?=w999:bool)
    n3008 = Subtract(x=w974, y=w975) -> (x-y=w976:dbl)
    n3009 = Increment(x=w1072) -> (x+1=w1071:i32)
    n3010 = Equal?(x=w989, y=1.0) -> (x = y?=w984:bool)
    n3011 = Compound Arithmetic op=AND(w984, "Reinforced\nchariot", w1005, w962, w982) -> (w981:bool)
    n3012 = Equal?(x=w972, y=2.0) -> (x = y?=w977:bool)
    n3013 = Subtract(x=w994, y=w995) -> (x-y=w996:dbl)
    n3014 = Compound Arithmetic op=AND(w977, "Caravan", w968, w959, w979) -> (w980:bool)
    n3015 = case shown="True" w1124 {
      tunnel: w1131 -> [_ w3027]
      tunnel: w1128 -> [_ w3026]
      frame False {
      }
      frame True {
        n3016 = local write "EP"(w3026) -> ()
        n3017 = local write "Writing level"(w3027) -> ()
      }
    }
    n3018 = Increment(x=w989) -> (x+1=w988:i32)
    n3019 = Equal?(x=w992, y=0.0) -> (x = y?=w997:bool)
    n3020 = Increment(x=w972) -> (x+1=w973:i32)
    n3021 = Compound Arithmetic op=AND(w997, "Simple\nchariot", w1006, w965, w999) -> (w1000:bool)
    n3022 = Increment(x=w992) -> (x+1=w993:i32)
    n3023 = case shown="True" w1144 {
      tunnel: w1151 -> [_ w3023]
      tunnel: w1148 -> [_ w3022]
      frame False {
      }
      frame True {
        n3024 = local write "EP"(w3022) -> ()
        n3025 = local write "Writing level"(w3023) -> ()
      }
    }
    n3026 = case shown="True" w608 {
      tunnel: w601 -> [_ w2824]
      tunnel: w604 -> [_ w2823]
      frame False {
      }
      frame True {
        n3027 = local write "EP"(w2823) -> ()
        n3028 = local write "Writing level"(w2824) -> ()
      }
    }
    n3029 = case shown="True" w1123 {
      tunnel: w1116 -> [_ w3021]
      tunnel: w1119 -> [_ w3020]
      frame False {
      }
      frame True {
        n3030 = local write "Animal\ndomestication\nlevel"(w3021) -> ()
        n3031 = local read "hunting b"() -> (w3019:dbl)
        n3032 = local write "EP"(w3020) -> ()
        n3033 = Add(x=w3019, y=0.25) -> (x+y=w3018:dbl)
        n3034 = local write "hunting b"(w3018) -> ()
      }
    }
    n3035 = case shown="True" w1103 {
      tunnel: w1096 -> [_ w3008]
      tunnel: w1099 -> [_ w3007]
      frame False {
      }
      frame True {
        n3036 = local write "Animal\ndomestication\nlevel"(w3008) -> ()
        n3037 = local read "warrior a"() -> (w3004:dbl)
        n3038 = local read "Construction multiplier"() -> (w3002:dbl)
        n3039 = local write "EP"(w3007) -> ()
        n3040 = Add(x=w3002, y=0.25) -> (x+y=w3003:dbl)
        n3041 = Add(x=w3004, y=0.25) -> (x+y=w3006:dbl)
        n3042 = local write "Construction multiplier"(w3003) -> ()
        n3043 = local write "warrior a"(w3006) -> ()
      }
    }
    n3044 = case shown="True" w1143 {
      tunnel: w1136 -> [_ w3025]
      tunnel: w1139 -> [_ w3024]
      frame False {
      }
      frame True {
        n3045 = local write "EP"(w3024) -> ()
        n3046 = local write "Writing level"(w3025) -> ()
      }
    }
    n3047 = case shown="True" w1104 {
      tunnel: w1111 -> [_ w3016]
      tunnel: w1108 -> [_ w3015]
      frame False {
      }
      frame True {
        n3048 = local write "Animal\ndomestication\nlevel"(w3016) -> ()
        n3049 = local write "EP"(w3015) -> ()
        n3050 = local read "warrior b"() -> (w3012:dbl)
        n3051 = local read "Construction multiplier"() -> (w3010:dbl)
        n3052 = Add(x=w3010, y=0.25) -> (x+y=w3009:dbl)
        n3053 = Add(x=w3012, y=0.25) -> (x+y=w3013:dbl)
        n3054 = local write "Construction multiplier"(w3009) -> ()
        n3055 = local write "warrior b"(w3013) -> ()
      }
    }
    n3056 = case shown="True" w850 {
      tunnel: w854 -> [_ w2934]
      tunnel: w853 -> [_ w2933]
      tunnel: w859 -> [_ w2931]
      tunnel: [0 w2931] -> w851
      frame False {
      }
      frame True {
        n3057 = Subtract(x=w2934, y=w2933) -> (x-y=w2932:dbl)
        n3058 = local write "SP"(w2932) -> ()
        n3059 = local write "Production\nlevel"(w2931) -> ()
      }
    }
    n3060 = case shown="True" w1724 {
      tunnel: w1723 -> [_ w3229]
      tunnel: w1722 -> [_ w3232]
      tunnel: w1721 -> [_ w3235]
      tunnel: w1720 -> [_ w3238]
      tunnel: w1719 -> [_ w3241]
      tunnel: w1718 -> [_ w3244]
      tunnel: w1717 -> [_ w3243]
      tunnel: w1716 -> [_ w3240]
      tunnel: w1715 -> [_ w3237]
      tunnel: w1714 -> [_ w3234]
      tunnel: w1713 -> [_ w3231]
      tunnel: w1712 -> [_ w3228]
      tunnel: w851 -> [_ w3217]
      tunnel: w850 -> [_ w3216]
      frame False {
      }
      frame True {
        n3061 = Boolean To (0,1)(Boolean=w3228) -> (0, 1=w3227:i16)
        n3062 = Boolean To (0,1)(Boolean=w3231) -> (0, 1=w3230:i16)
        n3063 = Boolean To (0,1)(Boolean=w3234) -> (0, 1=w3233:i16)
        n3064 = Boolean To (0,1)(Boolean=w3243) -> (0, 1=w3242:i16)
        n3065 = Boolean To (0,1)(Boolean=w3237) -> (0, 1=w3236:i16)
        n3066 = Boolean To (0,1)(Boolean=w3240) -> (0, 1=w3239:i16)
        n3067 = Boolean To (0,1)(Boolean=w3216) -> (0, 1=w3219:i16)
        n3068 = Multiply(x=w3227, y=w3229) -> (x*y=w3226:i32)
        n3069 = Multiply(x=w3230, y=w3232) -> (x*y=w3225:i32)
        n3070 = Multiply(x=w3233, y=w3235) -> (x*y=w3224:i32)
        n3071 = Multiply(x=w3242, y=w3244) -> (x*y=w3221:i32)
        n3072 = Multiply(x=w3236, y=w3238) -> (x*y=w3223:i32)
        n3073 = Multiply(x=w3239, y=w3241) -> (x*y=w3222:i32)
        n3074 = Multiply(x=w3219, y=w3217) -> (x*y=w3218:i32)
        n3075 = Compound Arithmetic op=ADD(w3226, w3225, w3224, w3223, w3222, w3221, w3218) -> (w3220:i32)
        n3076 = case shown="1" w3220 {
          frame 0, Default {
          }
          frame 1 {
            n3077 = local read "# of level 1 sciences"() -> (w3246:i32)
            n3078 = Increment(x=w3246) -> (x+1=w3245:i32)
            n3079 = local write "# of level 1 sciences"(w3245) -> ()
          }
          frame 2 {
            n3080 = local read "# of level 2 sciences"() -> (w3248:i32)
            n3081 = Increment(x=w3248) -> (x+1=w3247:i32)
            n3082 = local write "# of level 2 sciences"(w3247) -> ()
          }
          frame 3 {
            n3083 = local read "# of level 3 sciences"() -> (w3250:i32)
            n3084 = Increment(x=w3250) -> (x+1=w3249:i32)
            n3085 = local write "# of level 3 sciences"(w3249) -> ()
          }
          frame 4 {
            n3086 = local read "# of level 4 sciences"() -> (w3252:i32)
            n3087 = Increment(x=w3252) -> (x+1=w3251:i32)
            n3088 = local write "# of level 4 sciences"(w3251) -> ()
          }
          frame 5 {
            n3089 = local read "# of level 5 sciences"() -> (w3254:i32)
            n3090 = Increment(x=w3254) -> (x+1=w3253:i32)
            n3091 = local write "# of level 5 sciences"(w3253) -> ()
          }
          frame 6 {
            n3092 = local read "# of level 6 sciences"() -> (w3256:i32)
            n3093 = Increment(x=w3256) -> (x+1=w3255:i32)
            n3094 = local write "# of level 6 sciences"(w3255) -> ()
          }
          frame 7 {
            n3095 = local read "# of level 7 sciences"() -> (w3258:i32)
            n3096 = Increment(x=w3258) -> (x+1=w3257:i32)
            n3097 = local write "# of level 7 sciences"(w3257) -> ()
          }
          frame 8 {
            n3098 = local read "# of level 8 sciences"() -> (w3260:i32)
            n3099 = Increment(x=w3260) -> (x+1=w3259:i32)
            n3100 = local write "# of level 8 sciences"(w3259) -> ()
          }
          frame 9 {
            n3101 = local read "# of level 9 sciences"() -> (w3262:i32)
            n3102 = Increment(x=w3262) -> (x+1=w3261:i32)
            n3103 = local write "# of level 9 sciences"(w3261) -> ()
          }
          frame 10 {
            n3104 = local read "# of level 10 sciences"() -> (w3264:i32)
            n3105 = Increment(x=w3264) -> (x+1=w3263:i32)
            n3106 = local write "# of level 10 sciences"(w3263) -> ()
          }
        }
      }
    }
    n3107 = case shown="True" w1064 {
      tunnel: w1071 -> [_ w3000]
      tunnel: w1068 -> [_ w2999]
      frame False {
      }
      frame True {
        n3108 = local write "EP"(w2999) -> ()
        n3109 = local read "warrior b"() -> (w2998:dbl)
        n3110 = local write "Sword level"(w3000) -> ()
        n3111 = Add(x=w2998, y=0.25) -> (x+y=w2996:dbl)
        n3112 = local write "warrior b"(w2996) -> ()
      }
    }
    n3113 = case shown="True" w1084 {
      tunnel: w1091 -> [_ w2990]
      tunnel: w1088 -> [_ w2989]
      frame False {
      }
      frame True {
        n3114 = local read "warrior a"() -> (w2986:dbl)
        n3115 = local write "EP"(w2989) -> ()
        n3116 = local write "Sword level"(w2990) -> ()
        n3117 = Add(x=w2986, y=0.25) -> (x+y=w2988:dbl)
        n3118 = local write "warrior a"(w2988) -> ()
      }
    }
    n3119 = case shown="True" w1000 {
      tunnel: w993 -> [_ w2979]
      tunnel: w996 -> [_ w2978]
      frame False {
      }
      frame True {
        n3120 = local write "EP"(w2978) -> ()
        n3121 = local read "warrior b"() -> (w2977:dbl)
        n3122 = local write "Chariot level"(w2979) -> ()
        n3123 = Add(x=w2977, y=0.25) -> (x+y=w2976:dbl)
        n3124 = local write "warrior b"(w2976) -> ()
      }
    }
    n3125 = case shown="True" w1083 {
      tunnel: w1076 -> [_ w2995]
      tunnel: w1079 -> [_ w2994]
      frame False {
      }
      frame True {
        n3126 = local write "EP"(w2994) -> ()
        n3127 = local read "warrior a"() -> (w2991:dbl)
        n3128 = local write "Sword level"(w2995) -> ()
        n3129 = Add(x=w2991, y=0.25) -> (x+y=w2992:dbl)
        n3130 = local write "warrior a"(w2992) -> ()
      }
    }
    n3131 = case shown="True" w981 {
      tunnel: w988 -> [_ w2974]
      tunnel: w985 -> [_ w2973]
      frame False {
      }
      frame True {
        n3132 = local write "EP"(w2973) -> ()
        n3133 = local read "warrior a"() -> (w2970:dbl)
        n3134 = local write "Chariot level"(w2974) -> ()
        n3135 = Add(x=w2970, y=0.25) -> (x+y=w2971:dbl)
        n3136 = local write "warrior a"(w2971) -> ()
      }
    }
    n3137 = case shown="True" w980 {
      tunnel: w973 -> [_ w2969]
      tunnel: w976 -> [_ w2968]
      frame False {
      }
      frame True {
        n3138 = local read "Trading level no mod"() -> (w2967:i32)
        n3139 = local write "EP"(w2968) -> ()
        n3140 = local write "Chariot level"(w2969) -> ()
        n3141 = Increment(x=w2967) -> (x+1=w2966:i32)
        n3142 = Increment(x=w2966) -> (x+1=w2965:i32)
        n3143 = local write "Trading level no mod"(w2965) -> ()
      }
    }
  }
  "warrior a" <- 1.0 ("warrior a")
  "hunting b" <- 2.0 ("hunting b")
  "hunting a" <- 1.0 ("hunting a")
  "warrior b" <- 1.0 ("warrior b")
  "Food" <- 5000.0
  "People" <- 1000
  "Permanent\nland" <- 100.0 ("Permanent\nland")
  "Conquered\nland" <- 300.0 ("Temporary\nland")
  "warrior c" <- 2.0 ("Numeric")
  "Hunters" <- 10 ("Hunters")
  "Unassigned workers" <- 0 ("Unassigned workers")
  "Builders" <- 0 ("Builders")
  "Warriors" <- 0 ("Warriors")
  "Scientists" <- 0 ("Hunters")
  "Crafters" <- 0 ("Builders")
  "Engineers" <- 0 ("Warriors")
  "EP" <- 0.0 ("Engineering\nPoints")
  "Spear level" <- 0 ("Spear level")
  "Net level" <- 0 ("Net level")
  "SP" <- 1000000000000.0 ("Numeric")
  "Military\nScience level" <- 0 ("Military level")
  "Dissent" <- 0.0 ("Dissent")
  "Government" <- "Democracy" ("String")
  "Governance\nlevel" <- 0 ("Numeric")
  "Warrior b Gov mult" <- 1 ("Warrior a Gov mult")
  "Land conv mult" <- 0 ("Land conv mult")
  "Temp land change/s" <- 0 ("Temp land captured/s")
  "1-Dissent/100" <- 1.0 ("1-Dissent/100")
  "Bow level" <- 0 ("Numeric")
  "Military Modifier" <- 1.0 ("Military Modifier")
  "Physics level" <- 0 ("Military level")
  "Construction\nlevel" <- 0 ("Numeric")
  "Boat level" <- 0 ("Spear level")
  "Trading level no mod" <- 0 ("Spear level")
  "Economics\nlevel" <- 0 ("Economic\nlevel")
  "Gold dbl" <- 0.0 ("Gold")
  "Taxation\nlevel" <- 0.0 ("Numeric")
  "Taxation\nModifier" <- 1.0 ("Numeric")
  "Farming level" <- 0 ("Numeric")
  "Biology\nlevel" <- 0 ("Numeric")
  "Hut level" <- 0 ("Numeric")
  "Road level" <- 0 ("Numeric")
  "Build points" <- 0 ("Numeric")
  "Non-land production multiplier" <- 1 ("Numeric")
  "Dissent \nmultiplication\nmodifier" <- 1.0 ("Dissent multiplication modifiers")
  "Hut non-land prod mod" <- 1 ("Numeric")
  "Hut upkeep" <- 0 ("Numeric")
  "Hut dissent mod" <- 1 ("Numeric")
  "Road land prod mod" <- 1 ("Numeric")
  "Road upkeep" <- 0 ("Numeric")
  "Road expansion bonus" <- 0 ("Numeric")
  "Trading level" <- 0 ("Spear level")
  "Gov building\nupkeep mod" <- 1 ("Numeric")
  "BP upkeep" <- 0.0 ("BP/s")
  "# of level 1 sciences" <- 0 ("Numeric")
  "# of level 2 sciences" <- 0 ("Numeric")
  "# of level 3 sciences" <- 0 ("Numeric")
  "# of level 4 sciences" <- 0 ("Numeric")
  "# of level 5 sciences" <- 0 ("Numeric")
  "# of level 6 sciences" <- 0 ("Numeric")
  "# of level 7 sciences" <- 0 ("Numeric")
  "# of level 8 sciences" <- 0 ("Numeric")
  "# of level 9 sciences" <- 0 ("Numeric")
  "# of level 10 sciences" <- 0 ("Numeric")
  "Hut invested points" <- 0 ("Numeric")
  "Road invested points" <- 0 ("Numeric")
  "Taxes dissent mod" <- 0 ("Numeric")
  "Gold income/s" <- 0.0 ("Gold income/s")
  "Barracks level" <- 0 ("Numeric")
  "Barracks military bonus" <- 1 ("Numeric")
  "Barracks upkeep" <- 0 ("Numeric")
  "Walls level" <- 0 ("Numeric")
  "Wall warrior % equivalent" <- 0 ("Numeric")
  "Wall upkeep" <- 0 ("Numeric")
  "Wall dissent mod" <- 1 ("Numeric")
  "Barracks\ninvested points" <- 0 ("Numeric")
  "Wall invested points" <- 0 ("Numeric")
  "Construction\ntools level" <- 0 ("Numeric")
  "Gold upkeep" <- 0 ("Land conv mult")
  "Construction multiplier" <- 1 ("Construction multiplier")
  "BP income" <- 0.0 ("Construction multiplier")
  "School level" <- 0 ("Numeric")
  "School engineer equivalent" <- 0 ("Numeric")
  "School upkeep" <- 0 ("Numeric")
  "School dissent mod" <- 1 ("Numeric")
  "School invested points" <- 0 ("Numeric")
  "School SP/EP multiplier" <- 1 ("Numeric")
  "Medicine level" <- 0 ("Spear level")
  "Medicine dissent mod" <- 1 ("Spear level")
  "University level" <- 0 ("Numeric")
  "University scientist equivalent" <- 0 ("Numeric")
  "University upkeep" <- 0 ("Numeric")
  "University dissent mod" <- 1 ("Numeric")
  "University\ninvested points" <- 0 ("Numeric")
  "University SP multiplier" <- 1 ("Numeric")
  "Gov populist\nbuildings mod" <- 1 ("Numeric")
  "Gov elitist\nbuildings mod" <- 1 ("Numeric")
  "Dissent mult per\nmilitary building" <- 1 ("Numeric")
  "Gov Economy\nbuildings mod" <- 1 ("Numeric")
  "Food dissent mod" <- 1 ("Numeric")
  "Food consumption\nmultiplier" <- 1 ("Numeric")
  "Food income" <- 0 ("food check")
  "EP income" <- 0.0 ("Construction multiplier")
  "SP income" <- 0.0 ("Construction multiplier")
  "Animal\ndomestication\nlevel" <- 0 ("Numeric")
  "Sword level" <- 0 ("Numeric")
  "Tax method\nlevel" <- 0 ("Numeric")
  "Chariot level" <- 0 ("Numeric")
  "Siege weapon\nlevel" <- 0 ("Numeric")
  "Writing level" <- 0 ("Numeric")
  "Aqueduct level" <- 0 ("Numeric")
  "Aqueduct upkeep" <- 0 ("Numeric")
  "Aqueduct dissent mod" <- 1 ("Numeric")
  "Aqueduct\ninvested points" <- 0 ("Numeric")
  "Police force level" <- 0 ("Numeric")
  "Police force upkeep" <- 0 ("Numeric")
  "Police force dissent mult" <- 1 ("Numeric")
  "Police force\ninvested points" <- 0 ("Numeric")
  "Harbor level" <- 0 ("Numeric")
  "Harbor upkeep" <- 0 ("Numeric")
  "Harbor expansion bonus" <- 0 ("Numeric")
  "Harbor\ninvested points" <- 0 ("Numeric")
  "Market level" <- 0 ("Numeric")
  "Market upkeep" <- 0 ("Numeric")
  "Market trade gold mult" <- 1 ("Numeric")
  "Market\ninvested points" <- 0 ("Numeric")
  "Temple level" <- 0 ("Numeric")
  "Temple upkeep" <- 0 ("Numeric")
  "Temple dissent mod" <- 1 ("Numeric")
  "Temple\ninvested points" <- 0 ("Numeric")
  "SP/EP multiplier" <- 0.0 ("Construction multiplier")
  "Harbor military mod" <- 1 ("Numeric")
  "Production\nlevel" <- 0 ("Numeric")
  "Tier 1\nproducts" <- 0.0 ("Gold")
  "Tier 2\nproducts" <- 0.0 ("Gold")
  "Tier 3\nproducts" <- 0.0 ("Gold")
  "Tier 4\nproducts" <- 0.0 ("Gold")
  "Tier 1\nproducts\nupkeep" <- 0.0 ("Gold")
  "Tier 2\nproducts\nupkeep" <- 0.0 ("Gold")
  "Tier 3\nproducts\nupkeep" <- 0.0 ("Gold")
  "Tier 4\nproducts\nupkeep" <- 0.0 ("Gold")
  "Temple SP/EP multiplier" <- 1 ("Numeric")
  "Aqueduct food multiplier" <- 1 ("Numeric")
  "Gold" <- 0 ("Gold")
  "Optics\nlevel" <- 0 ("Optics\nlevel")
  "Electronics\nlevel" <- 0 ("Optics\nlevel")
  "Vehicle\nlevel" <- 0 ("Optics\nlevel")
  "Brick house\nunlocked" <- FALSE ("Brick house\nunlocked")
  "Concrete house\nunlocked" <- FALSE ("Brick house\nunlocked")
  "Housing type" <- "Hut" ("Housing type")
  "Mutilayer\nStone roads\nunlocked" <- FALSE ("Brick house\nunlocked")
  "Paved tar roads\nunlocked" <- FALSE ("Brick house\nunlocked")
  "Road type" <- "Stone" ("Housing type")
  "Road trade modifier" <- 0 ("Numeric")
  "Gov food mult" <- 1.0 ("Gov food bonus")
  "Police force base dissent mod" <- 0 ("Numeric")
  "Market domestic gold mult" <- 0 ("Numeric")
